vi "main 1.17b DEBUG.vi"() -> ()   [LabVIEW 2015]
uses:
  subvi/PHOIBOS/DEFINITIONS/DEF_dev_state.ctl
  subvi/PHOIBOS/DEFINITIONS/DEF_dev_type.ctl
  <vilib>/Analysis/_algsub.llb/Real Vector Norm.vi
  <vilib>/Analysis/1siggen.llb/Ramp Pattern by Samples.vi
  <vilib>/DAQmx/create/channels.llb/DAQmx Create Channel (DI-Digital Input).vi
  <userlib>/caLab/Private/Put_DBL_PV.vi
  <vilib>/Utility/file.llb/Write Delimited Spreadsheet (string).vi
  <vilib>/Utility/file.llb/Read Delimited Spreadsheet (string).vi
  <userlib>/caLab/Private/Get_PV.vi
  <vilib>/Utility/file.llb/Write Delimited Spreadsheet (DBL).vi
  subvi/Newport ESP301/Newport ESP301.lvlib
  subvi/sp_manip.llb/sp_manip_lib.lvlib
  subvi/sp_manip.llb/tcp_gateway.lvlib
  <vilib>/Analysis/NI_AALBase.lvlib
  <vilib>/Analysis/NI_AALPro.lvlib
  subvi/ZaberTSeries/ZaberTSeries.lvlib
panel:
  in  "file path (use dialog)":path=path "C:/Users/femtolab_admin/Desktop/debug.txt"
  out "Pics L":i32=200
  out "Waveform Chart":dbl(graph)
  out "G2 X":cluster{dbl[], "Ramp Pattern":dbl[]}(graph)={array[344 elements], "Ramp Pattern"=[0.0, 0.0, 0.0, 0.0, 0.0, 0.0, 0.0, 0.0, 0.0, 0.0, 0.0, 0.0, 0.0, 0.0, 0.0, 0.0, 0.0, 0.0, 0.0, 0.0, 0.0, 12.377241379310345, 41.64689655172414, 18.335172413793103, 0.0, 0.0, 0.0, 0.0, 0.0, 0.0, 0.0, 0.0, 0.0, 0.0, 0.0, 0.0, 0.0, 0.0, 0.0, 0.0, 0.0, 0.0, 0.0, 0.0, 0.0, 0.0, 0.0, 0.0, 0.0, 0.0, 0.0, 0.0, 0.0, 0.0, 0.0, 0.0, 0.0, 0.0, 0.0, 0.0, 0.0, 0.0, 0.0, 0.0, 0.0, 0.0, 0.0, 0.0, 0.0, 0.0, 0.0, 0.0, 0.0, 0.0, 0.0, 0.0, 0.0, 0.0, 0.0, 0.0, 0.0, 0.0, 0.0, 0.0, 0.0, 0.0, 0.0, 0.0, 0.0, 0.0, 0.0, 0.0, 0.0, 0.0, 0.0, 0.0, 0.0, 0.0, 0.0, 0.0, 0.0, 0.0, 0.0, 0.0, 0.0, 0.0, 0.0, 0.0, 0.0, 0.0, 0.0, 0.0, 0.0, 0.0, 0.0, 17.495517241379314, 48.13413793103449, 27.429999999999996, 0.0, 0.0, 0.0, 0.0, 0.0, 0.0, 0.0, 0.0, 0.0, 0.0, 0.0, 0.0, 0.0, 0.0, 0.0, 0.0, 0.0, 0.0, 0.0, 0.0, 0.0, 0.0, 0.0, 0.0, 0.0, 0.0, 0.0, 0.0, 0.0, 0.0, 0.0, 0.0, 0.0, 0.0, 0.0, 0.0, 0.0, 0.0, 0.0, 0.0, 0.0, 0.0, 0.0, 0.0, 0.0, 0.0, 0.0, 0.0, 0.0, 0.0, 0.0, 0.0, 0.0, 0.0, 0.0, 0.0, 0.0, 0.0, 0.0, 0.0, 0.0, 0.0, 0.0, 0.0, 17.760344827586206, 28.923448275862068, 17.532068965517244, 0.0, 0.0, 0.0, 0.0, 0.0, 0.0, 0.0, 0.0, 0.0, 0.0, 0.0, 0.0, 0.0, 0.0, 0.0, 0.0, 0.0, 0.0, 0.0, 0.0, 0.0, 0.0, 0.0, 0.0, 0.0, 0.0, 0.0, 0.0, 0.0, 0.0, 0.0, 0.0, 0.0, 0.0, 0.0, 0.0, 0.0, 0.0, 0.0, 0.0, 0.0, 0.0, 0.0, 0.0, 0.0, 2.201724137931034, 1.9948275862068956, 0.0, 0.0, 0.0, 0.0, 0.0, 0.0, 0.0, 0.0, 0.0, 0.0, 0.0, 0.0, 0.0, 0.0, 0.0, 0.0, 0.0, 0.0, 0.0, 0.0, 0.0, 0.0, 0.0, 0.0, 0.0, 0.0, 0.0, 0.0, 0.0, 0.0, 0.0, 0.0, 0.0, 0.0, 0.0, 0.0, 0.0, 0.0, 0.0, 0.0, 0.0, 0.0, 0.0, 0.0, 0.0, 0.0, 0.0, 0.0, 0.0, 0.0, 0.0, 0.0, 0.0, 0.0, 0.0, 0.0, 0.0, 0.0, 0.0, 0.0, 0.0, 0.0, 0.0, 0.0, 0.0, 0.0, 0.0, 0.0, 0.0, 0.0, 0.0, 0.0, 0.0, 0.0, 0.0, 0.0, 0.0, 0.0, 0.0, 0.0, 0.0, 0.0, 0.0, 0.0, 0.0, 0.0, 0.0, 0.0, 0.0, 0.0, 0.0, 0.0, 0.0, 0.0, 0.0, 0.0, 0.0, 0.0, 0.0, 0.0, 0.0, 0.0, 0.0, 0.0, 0.0, 0.0, 0.0, 0.0, 0.0, 0.0, 0.0, 0.0]}
  in  "reset every n pics":bool=TRUE
  in  "pics2avg":i32=50
  in  "abort acq.":bool
  out "G2 Y":cluster{dbl[], "Ramp Pattern":dbl[]}(graph)={[0.0, 0.0, 0.0, 0.0, 0.0, 0.0, 0.0, 0.0, 0.0, 0.0, 0.0, 0.0, 0.0, 0.0, 0.0, 0.0, 0.0, 0.0, 0.0, 0.0, 0.0, 0.0, 0.0, 0.0, 0.0, 0.0, 0.0, 0.0, 0.0, 0.0, 0.0, 0.0, 0.0, 0.0, 0.0, 0.0, 0.0, 0.0, 0.0, 0.0, 0.0, 0.0, 0.0, 0.0, 0.0, 0.0, 0.0, 0.0, 0.0, 0.0, 0.0, 0.0, 0.0, 0.0, 0.0, 0.0, 0.0, 0.0, 0.0, 0.0, 0.0, 0.0, 0.0, 0.0, 0.0, 0.0, 0.0, 0.0, 0.0, 0.0, 0.0, 0.0, 0.0, 0.0, 0.0, 0.0, 0.0, 0.0, 0.0, 0.0, 0.0, 0.0, 0.0, 0.0, 0.0, 0.0, 0.0, 0.0, 0.0, 0.0, 0.0, 0.0, 0.0, 0.0, 0.0, 0.0, 0.0, 0.0, 0.0, 0.0, 0.0, 0.0, 0.0, 0.0, 0.0, 0.0, 0.0, 0.0, 0.0, 0.0, 0.0, 0.0, 0.0, 0.0, 0.0, 0.0, 0.0, 0.0, 0.0, 0.0, 0.0, 0.0, 0.0, 0.0, 0.0, 0.0, 0.0, 0.0, 0.0, 0.0, 0.0, 0.0, 0.0, 0.0, 0.0, 0.0, 0.0, 0.0, 0.0, 0.0, 0.0, 0.0, 0.0, 0.0, 0.0, 0.0, 0.0, 0.0, 0.0, 0.0, 0.0, 0.0, 0.0, 0.0, 0.0, 0.0, 0.0, 0.0, 0.0, 0.0, 0.0, 0.0, 0.0, 0.0, 0.0, 0.0, 0.0, 0.0, 0.0, 0.0, 0.0, 0.0, 0.0, 0.0, 0.0, 0.0, 0.0, 0.0, 0.0, 0.0, 0.0, 0.0, 0.0, 0.0, 0.0, 0.0, 0.0, 0.0, 0.0, 0.0, 0.0, 0.0, 0.0, 0.0, 0.0, 0.0, 0.0, 0.0, 0.0, 0.0, 0.0, 0.0, 0.0, 0.0, 0.0, 0.0, 0.0, 0.0, 0.0, 0.0, 0.0, 0.0, 0.0, 0.0, 0.0, 0.0, 0.0, 0.0, 0.0, 0.0, 0.0, 0.0, 0.0, 0.0, 0.0, 0.0, 0.0, 0.0, 0.0, 0.0, 0.0, 0.0, 0.0, 0.0, 0.0, 0.0, 0.0, 0.0, 0.0, 0.0, 0.0, 0.0, 0.0, 0.0, 0.0, 0.0, 0.0, 0.0, 0.0, 0.0, 0.0, 0.0, 0.0, 0.0, 0.0, 0.0], "Ramp Pattern"=[0.0, 1.003921568627451, 2.007843137254902, 3.011764705882353, 4.015686274509804, 5.019607843137255, 6.023529411764706, 7.027450980392157, 8.031372549019608, 9.035294117647059, 10.03921568627451, 11.04313725490196, 12.047058823529412, 13.050980392156863, 14.054901960784314, 15.058823529411764, 16.062745098039215, 17.066666666666666, 18.070588235294117, 19.07450980392157, 20.07843137254902, 21.08235294117647, 22.08627450980392, 23.090196078431372, 24.094117647058823, 25.098039215686274, 26.101960784313725, 27.105882352941176, 28.109803921568627, 29.113725490196078, 30.11764705882353, 31.12156862745098, 32.12549019607843, 33.129411764705885, 34.13333333333333, 35.13725490196079, 36.141176470588235, 37.14509803921569, 38.14901960784314, 39.15294117647059, 40.15686274509804, 41.16078431372549, 42.16470588235294, 43.168627450980395, 44.17254901960784, 45.1764705882353, 46.180392156862744, 47.1843137254902, 48.188235294117646, 49.1921568627451, 50.19607843137255, 51.2, 52.20392156862745, 53.207843137254905, 54.21176470588235, 55.21568627450981, 56.219607843137254, 57.22352941176471, 58.227450980392156, 59.23137254901961, 60.23529411764706, 61.23921568627451, 62.24313725490196, 63.247058823529414, 64.25098039215686, 65.25490196078431, 66.25882352941177, 67.26274509803922, 68.26666666666667, 69.27058823529411, 70.27450980392157, 71.27843137254902, 72.28235294117647, 73.28627450980392, 74.29019607843138, 75.29411764705883, 76.29803921568627, 77.30196078431372, 78.30588235294118, 79.30980392156863, 80.31372549019608, 81.31764705882352, 82.32156862745099, 83.32549019607843, 84.32941176470588, 85.33333333333333, 86.33725490196079, 87.34117647058824, 88.34509803921569, 89.34901960784313, 90.3529411764706, 91.35686274509804, 92.36078431372549, 93.36470588235294, 94.3686274509804, 95.37254901960785, 96.37647058823529, 97.38039215686274, 98.3843137254902, 99.38823529411765, 100.3921568627451, 101.39607843137254, 102.4, 103.40392156862745, 104.4078431372549, 105.41176470588235, 106.41568627450981, 107.41960784313726, 108.4235294117647, 109.42745098039215, 110.43137254901961, 111.43529411764706, 112.43921568627451, 113.44313725490196, 114.44705882352942, 115.45098039215686, 116.45490196078431, 117.45882352941176, 118.46274509803922, 119.46666666666667, 120.47058823529412, 121.47450980392156, 122.47843137254903, 123.48235294117647, 124.48627450980392, 125.49019607843137, 126.49411764705883, 127.49803921568628, 128.50196078431372, 129.50588235294117, 130.50980392156862, 131.51372549019607, 132.51764705882354, 133.521568627451, 134.52549019607844, 135.52941176470588, 136.53333333333333, 137.53725490196078, 138.54117647058823, 139.54509803921567, 140.54901960784315, 141.5529411764706, 142.55686274509804, 143.5607843137255, 144.56470588235294, 145.5686274509804, 146.57254901960783, 147.57647058823528, 148.58039215686276, 149.5843137254902, 150.58823529411765, 151.5921568627451, 152.59607843137255, 153.6, 154.60392156862744, 155.6078431372549, 156.61176470588236, 157.6156862745098, 158.61960784313726, 159.6235294117647, 160.62745098039215, 161.6313725490196, 162.63529411764705, 163.6392156862745, 164.64313725490197, 165.64705882352942, 166.65098039215687, 167.65490196078431, 168.65882352941176, 169.6627450980392, 170.66666666666666, 171.6705882352941, 172.67450980392158, 173.67843137254903, 174.68235294117648, 175.68627450980392, 176.69019607843137, 177.69411764705882, 178.69803921568626, 179.7019607843137, 180.7058823529412, 181.70980392156864, 182.71372549019608, 183.71764705882353, 184.72156862745098, 185.72549019607843, 186.72941176470587, 187.73333333333332, 188.7372549019608, 189.74117647058824, 190.7450980392157, 191.74901960784314, 192.75294117647059, 193.75686274509803, 194.76078431372548, 195.76470588235293, 196.7686274509804, 197.77254901960785, 198.7764705882353, 199.78039215686275, 200.7843137254902, 201.78823529411764, 202.7921568627451, 203.79607843137254, 204.8, 205.80392156862746, 206.8078431372549, 207.81176470588235, 208.8156862745098, 209.81960784313725, 210.8235294117647, 211.82745098039214, 212.83137254901962, 213.83529411764707, 214.8392156862745, 215.84313725490196, 216.8470588235294, 217.85098039215686, 218.8549019607843, 219.85882352941175, 220.86274509803923, 221.86666666666667, 222.87058823529412, 223.87450980392157, 224.87843137254902, 225.88235294117646, 226.8862745098039, 227.89019607843136, 228.89411764705883, 229.89803921568628, 230.90196078431373, 231.90588235294118, 232.90980392156862, 233.91372549019607, 234.91764705882352, 235.92156862745097, 236.92549019607844, 237.9294117647059, 238.93333333333334, 239.93725490196078, 240.94117647058823, 241.94509803921568, 242.94901960784313, 243.95294117647057, 244.95686274509805, 245.9607843137255, 246.96470588235294, 247.9686274509804, 248.97254901960784, 249.9764705882353, 250.98039215686273, 251.98431372549018, 252.98823529411766, 253.9921568627451, 254.99607843137255, 256.0]}
  out "ETA":timestamp=timestamp(3655133644.4615793 s since 1904-01-01) format="%<%H:%M:%S>T"
  out "acq. imgs":i32=200
  out "snap_prog":dbl(slide)=1.0 scale=0.0..1.0
  in  "BasePath":path=path "T:/trARPES/PESData"
  in  "cam_liveavg":bool=TRUE caption="live average"
  out "cam_fps":dbl=19.690658487387566 caption="FPS" format="%.1g"
  out "sideimg":dbl[][](graph)
  out "RunNumber":u16=3091
  out "sum":dbl format="%#.2g"
  out "max":dbl=22.774482758620692
  out "mainimg":dbl[][](graph)
  out "ESP_con?":bool=TRUE caption="ESP301"
  out "phoib_con?":bool caption="PHOIBOS"
  out "manip_con?":bool=TRUE caption="manipulator"
  out "cam_con?":bool caption="camera"
  in  "main_close":bool=TRUE
  in  "Tab Control":enum32{"live", "scan", "devices"}(tab)=enum."devices"
  in  "wattpilot_set":bool
  out "Readback_wattpilot":dbl=304.89
  in  "Set Powet (%)":dbl
  out "Readback":dbl=340.0
  out "In Range":bool
  in  "setpoint_set":bool
  in  "Setpoint":dbl=302.0
  out "TB":dbl=304.91
  out "TA":dbl=304.49
  in  "phoib_I_10s":dbl
  out "phoib_I_10":dbl caption="Mesh Back"
  in  "mirr_go":bool
  in  "ESP_opent0file":bool
  in  "mirr_rel":i32=1 caption="relative [steps]"
  in  "mirr_Y-":bool
  in  "mirr_Y+":bool
  in  "mirr_X+":bool
  in  "mirr_X-":bool
  in  "manip_deltas":dbl[](array[numeric])=[0.0, 0.0, 5.0, 0.0, 0.0, 0.0] caption="delta" format="%#.5g"
  in  "aq.mode":enum32{"Radio Selection 1", "Radio Selection 2"}(radio)=enum."Radio Selection 2"
  in  "dark avg":i32=100
  in  "cam_avgs":i32=20 caption="N"
  in  "ESP_delta":dbl caption="relative [mm]"
  in  "ESP_-":bool
  in  "ESP_+":bool
  in  "ESP_go":bool
  in  "ESP_dest_t":dbl=728236.1319443199 caption="[fs]"
  in  "ESP_dest":dbl=-35.84015 caption="[mm]"
  in  "ESP_set_t0":bool
  in  "phoib_I_6s":dbl=3200.0
  in  "phoib_I_5s":dbl=1500.0
  in  "phoib_I_4s":dbl=4.558
  in  "phoib_I_3s":dbl=-10.0
  in  "phoib_I_2s":dbl=35.0
  in  "phoib_I_1s":dbl=21.0
  in  "phoib_standby":bool
  in  "phoib_set":bool
  out "phoib_I_6":dbl=3200.0 caption="Screen Voltage"
  out "phoib_I_5":dbl=1500.0 caption="Detctor Voltage"
  out "phoib_I_4":dbl=4.558 caption="Work Function"
  out "phoib_I_3":dbl=-10.0 caption="Coil Current"
  out "phoib_I_2":dbl=35.0 caption="Pass Energy"
  out "phoib_I_1":dbl=21.0 caption="Kinetic Energy"
  out "Saved Positions":string[][](table)=[["ertwertwert", "-2.299945", "-2.030214", "38.900024", "50.000762", "0.000887", "-97.998082"], ["uztgugt", "-14.999451", "-13.638894", "442.380066", "13.998380", "-1.893758", "-76.305838"], ["asdf", "-14.999451", "-13.638894", "442.380066", "13.998380", "-1.893758", "-76.305838"], ["test3", "-14.999451", "-13.638894", "441.380066", "13.998380", "-1.893758", "-76.305838"]]
  in  "Save Pos":bool
  in  "Load":bool
  in  "Delete":bool
  in  "ManipRel +":bool
  in  "ManipRel -":bool
  in  "Move Abs":bool
  in  "stop manip":bool
  in  "dest":dbl[](array[numeric])=[1.794011231344732, -4.007411134769244, 35.099853515625, 337.9843004481455, 2.0, 140.61656469713384] caption="destination" format="%#.5g"
  out "axis":string[](array[string])=["x", "y", "z", "polar", "tilt", "azimut"]
  out "pos":dbl[](array[numeric])=[1.794011231344732, -4.007411134769244, 35.099853515625, 337.9843004481455, 1.998632949125299, 140.61656469713384] caption="position" format="%.5f"
  in  "ana_mode":T1(ring)=enum."WideAngleMode"
  in  "ana_voltrange":enum16{"3.5kV", "1.5kV", "400V", "100V", "10V"}(ring)=enum."400V"
  out "ESP_pos":dbl=-35.84015 caption="Position"
  out "ESP_delay":dbl=-0.3335640952092252 caption="Delay"
  out "ESP_t0":dbl=-35.8401 caption="Time Zero @"
  out "phoib_I_7":dbl=-30.0 caption="Conversion Voltage"
  in  "phoib_I_7s":dbl=-30.0
  in  "phoib_I_8s":dbl=0.0039
  in  "phoib_I_9s":dbl
  out "phoib_I_8":dbl=0.0039 caption="FD1"
  out "phoib_I_9":dbl caption="Mesh Front"
  in  "gain":bool
  in  "cam_exp":u32=50 caption="exposure [ms]"
  in  "binning":u16(ring)=2 items=["X 1", "X 2", "X 4", "X 8"]
  in  "cam_dark?":bool=TRUE caption="subtract dark?"
  in  "cam_dark":bool
  in  "cam_saveimg":bool
  in  "e-size":u8
  in  "lower threshold":i32=50
  in  "count?":bool
  in  "ROI Left":i32=1
  in  "ROI Right":i32=43
  in  "ROI Top":i32=1
  in  "ROI Bottom":i32=33
  out "moving?":bool[](array[boolean])
  out "mirr_posX":i32=1955 caption="X"
  out "mirr_posY":i32=2950 caption="Y"
  in  "mirr_dest":i32[](array[numeric])=[60782, 121383]
  out "waveplate position":dbl format="%.6g"
  out "stage2 position":dbl format="%.6g"
  out "current scan 2":i32=3
  out "scan 1":dbl(slide)=1.0 scale=0.0..1.0
  in  "Tab Control 2":enum32{"setup", "data"}(tab)
  in  "scan_selector 2":T2(tab)
  in  "scan_manip_start 2":dbl[](array[numeric])=[1.794011231344732, -4.007411134769244, 35.099853515625, 337.9843004481455, 2.000390761745462, 140.61656469713384] caption="start position" format="%#.5g"
  in  "scan_manip_deltas 2":dbl[](array[numeric])=[0.0, 0.0, 0.0, 0.0, 1.0, 0.0] caption="direction vector\n(gets normalized)" format="%#.5g"
  in  "scan_manip_setstart 2":bool
  in  "scan_mirr_start 2":i32[](array[numeric])=[60782, 121383] caption="scan_mirr_start"
  in  "scan_mirr_deltas 2":i32[](array[numeric])=[1, 0] caption="direction vector\n(gets normalized)"
  in  "scan_mirr_setstart 2":bool
  in  "wait addional  2":dbl caption="s"
  in  "Wait for T 2":bool=TRUE
  in  "scan_volt_parameter 2":string(combo)="Kinetic Energy"
  in  "waypointsD2":string[][](table)
  in  "waypointsD1":string[][](table)=[["302", "1"], ["304", ""], ["", ""]]
  in  "load waypoints 1":bool
  in  "meas_iter":i32=1 caption="Iterations"
  in  "scan_selector":T2(tab)=enum."delay"
  in  "scan_manip_setstart":bool
  in  "scan_manip_start":dbl[](array[numeric])=[1.794011231344732, -4.007411134769244, 35.099853515625, 337.9843004481455, 2.000390761745462, 140.61656469713384] caption="start position" format="%#.5g"
  in  "scan_manip_deltas":dbl[](array[numeric])=[0.0, 0.0, 0.0, 0.0, 1.0, 0.0] caption="direction vector\n(gets normalized)" format="%#.5g"
  in  "scan_mirr_start":i32[](array[numeric])=[60782, 121383]
  in  "scan_mirr_deltas":i32[](array[numeric])=[1, 0] caption="direction vector\n(gets normalized)"
  in  "scan_mirr_setstart":bool
  in  "wait addional":dbl caption="s"
  in  "Wait for T":bool=TRUE
  in  "scan_volt_parameter":string(combo)="Kinetic Energy"
  in  "clear waypoints 1":bool
  in  "load waypoints 2":bool
  in  "clear waypoints 2":bool
  out "intensitygraph":cluster{"Array":dbl[], "Intensity Chart":dbl[]}(graph)={"Array"=[302.0, 303.0, 304.0], "Intensity Chart"=[1937.88, 12704.590000000002, 4640.840000000001]}
  out "energygraph":dbl[][](graph)=[[0.0, 0.0, 0.0, 64.28999999999999, 120.06, 0.0, 0.0, 0.0, 0.0, 0.0, 0.0, 0.0, 0.0, 0.0, 0.0, 0.0, 0.0, 0.0, 0.0, 0.0, 0.0, 0.0, 0.0, 0.0, 0.0, 0.0, 0.0, 0.0, 0.0, 0.0, 0.0, 0.0, 0.0, 0.0, 0.0, 0.0, 0.0, 0.0, 0.0, 0.0, 0.0, 0.0, 0.0, 0.0, 0.0, 0.0, 0.0, 0.0, 0.0, 384.53999999999996, 1103.3799999999999, 448.21000000000004, 0.0, 0.0, 0.0, 0.0, 0.0, 0.0, 0.0, 0.0, 0.0, 0.0, 0.0, 0.0, 0.0, 0.0, 0.0, 0.0, 0.0, 120.82, 0.0, 261.04, 195.1, 253.87, 199.70999999999998, 127.75, 87.50999999999999, 0.0, 52.54, 0.0, 0.0, 51.78, 55.73, 0.0, 0.0, 0.0, 0.0, 0.0, 0.0, 0.0, 0.0, 0.0, 0.0, 0.0, 0.0, 0.0, 0.0, 0.0, 0.0, 0.0, 0.0, 0.0, 0.0, 0.0, 0.0, 0.0, 0.0, 0.0, 0.0, 0.0, 0.0, 0.0, 0.0, 332.90999999999997, 1106.25, 934.74, 0.0, 156.76, 62.65, 0.0, 0.0, 0.0, 0.0, 0.0, 0.0, 54.62, 0.0, 0.0, 0.0, 0.0, 0.0, 0.0, 0.0, 0.0, 0.0, 0.0, 0.0, 0.0, 0.0, 0.0, 0.0, 0.0, 0.0, 0.0, 65.85, 165.75, 0.0, 0.0, 0.0, 0.0, 0.0, 0.0, 0.0, 0.0, 0.0, 0.0, 0.0, 0.0, 0.0, 0.0, 0.0, 0.0, 0.0, 266.63, 591.5, 261.64, 0.0, 391.9, 527.29, 82.87, 123.75, 286.74, 151.72, 0.0, 0.0, 0.0, 0.0, 0.0, 0.0, 0.0, 0.0, 0.0, 0.0, 0.0, 0.0, 0.0, 0.0, 0.0, 0.0, 0.0, 0.0, 0.0, 396.37, 721.0900000000001, 353.5, 83.97999999999999, 104.77000000000001, 0.0, 57.83, 60.98, 182.28, 128.78, 0.0, 0.0, 0.0, 465.25, 624.3399999999999, 348.62, 0.0, 0.0, 0.0, 0.0, 0.0, 0.0, 0.0, 0.0, 0.0, 0.0, 0.0, 0.0, 119.7, 217.91, 120.56, 0.0, 0.0, 0.0, 0.0, 0.0, 0.0, 0.0, 58.89, 0.0, 0.0, 0.0, 202.23999999999998, 149.79000000000002, 0.0, 117.82, 212.51999999999998, 534.74, 421.98, 50.97, 0.0, 0.0, 0.0, 0.0, 362.15999999999997, 656.04, 265.02, 0.0, 0.0, 0.0, 0.0, 0.0, 0.0, 0.0, 0.0, 0.0, 0.0, 0.0, 0.0, 0.0, 0.0, 0.0, 0.0, 0.0, 0.0, 0.0, 0.0, 0.0, 0.0, 0.0, 0.0, 0.0, 0.0, 0.0, 0.0, 0.0, 0.0, 0.0, 0.0, 0.0, 0.0, 0.0, 0.0, 0.0, 0.0, 0.0, 0.0, 0.0, 0.0, 0.0, 0.0, 0.0, 0.0, 0.0, 0.0, 0.0, 0.0, 0.0, 0.0, 0.0, 0.0, 0.0, 0.0, 0.0, 0.0, 0.0, 0.0, 0.0, 0.0, 0.0, 0.0, 237.67999999999998, 286.08, 130.9, 0.0, 0.0, 0.0, 0.0, 0.0, 0.0, 0.0, 0.0, 0.0, 0.0, 0.0, 0.0, 0.0, 0.0, 0.0, 0.0, 0.0, 0.0, 0.0, 0.0, 0.0, 0.0, 0.0, 0.0, 0.0, 0.0, 0.0, 0.0], [0.0, 0.0, 0.0, 0.0, 0.0, 0.0, 0.0, 0.0, 0.0, 0.0, 0.0, 0.0, 0.0, 0.0, 0.0, 0.0, 0.0, 485.13, 1279.2, 234.71, 0.0, 0.0, 0.0, 0.0, 0.0, 0.0, 0.0, 0.0, 0.0, 0.0, 0.0, 0.0, 50.5, 654.4200000000001, 511.98, 0.0, 0.0, 0.0, 0.0, 0.0, 0.0, 0.0, 0.0, 0.0, 0.0, 0.0, 0.0, 0.0, 0.0, 0.0, 0.0, 0.0, 0.0, 0.0, 0.0, 0.0, 0.0, 0.0, 63.72, 693.84, 574.54, 0.0, 0.0, 0.0, 68.68, 1054.28, 1010.9499999999999, 0.0, 0.0, 0.0, 0.0, 0.0, 0.0, 0.0, 0.0, 0.0, 0.0, 0.0, 56.57, 971.76, 1333.73, 330.0, 0.0, 0.0, 0.0, 0.0, 0.0, 349.33000000000004, 292.7, 0.0, 0.0, 0.0, 0.0, 0.0, 0.0, 82.77000000000001, 1059.23, 1069.87, 156.47, 0.0, 0.0, 0.0, 0.0, 293.91, 333.47, 551.4, 493.64, 73.72999999999999, 0.0, 0.0, 0.0, 0.0, 0.0, 0.0, 0.0, 0.0, 0.0, 0.0, 0.0, 0.0, 0.0, 0.0, 286.01, 543.0699999999999, 251.94, 0.0, 0.0, 0.0, 0.0, 0.0, 233.63, 968.4799999999999, 771.53, 109.94, 0.0, 123.07, 499.72999999999996, 431.4, 0.0, 0.0, 60.85, 69.5, 0.0, 0.0, 0.0, 0.0, 0.0, 0.0, 0.0, 0.0, 0.0, 0.0, 0.0, 0.0, 0.0, 0.0, 52.01, 0.0, 0.0, 0.0, 0.0, 0.0, 0.0, 0.0, 0.0, 0.0, 0.0, 0.0, 0.0, 0.0, 0.0, 0.0, 0.0, 0.0, 0.0, 0.0, 0.0, 0.0, 0.0, 0.0, 0.0, 0.0, 0.0, 0.0, 0.0, 0.0, 0.0, 0.0, 0.0, 0.0, 52.95, 478.8, 870.47, 572.83, 61.67, 268.19, 1143.4, 1804.2599999999998, 1145.6100000000001, 739.22, 904.59, 1109.3000000000002, 1233.6599999999999, 212.92, 0.0, 0.0, 105.95, 448.76000000000005, 1306.3500000000001, 1005.5900000000001, 68.8, 0.0, 57.94, 0.0, 0.0, 0.0, 0.0, 0.0, 0.0, 0.0, 0.0, 0.0, 0.0, 0.0, 0.0, 0.0, 0.0, 0.0, 0.0, 0.0, 0.0, 0.0, 0.0, 0.0, 0.0, 0.0, 0.0, 159.01, 520.94, 925.5600000000001, 1641.53, 2261.26, 1259.83, 0.0, 0.0, 0.0, 0.0, 0.0, 0.0, 136.69, 398.81, 382.02, 0.0, 0.0, 0.0, 0.0, 0.0, 0.0, 421.01, 1376.5800000000002, 1425.75, 268.07, 0.0, 345.84000000000003, 396.77, 0.0, 0.0, 0.0, 0.0, 0.0, 216.93, 727.65, 830.9, 774.2299999999999, 839.3900000000001, 309.97, 0.0, 0.0, 0.0, 0.0, 0.0, 0.0, 0.0, 100.57, 459.66, 305.86, 0.0, 0.0, 0.0, 0.0, 0.0, 0.0, 0.0, 0.0, 0.0, 0.0, 0.0, 0.0, 0.0, 0.0, 0.0, 0.0, 0.0, 0.0, 0.0, 0.0, 0.0, 0.0, 0.0, 0.0, 0.0, 64.97999999999999, 379.62, 337.15999999999997, 83.6, 463.66, 399.03999999999996, 0.0, 0.0, 0.0, 0.0, 0.0, 0.0, 0.0, 0.0, 0.0, 0.0, 0.0, 0.0, 0.0, 0.0, 0.0, 0.0, 0.0, 0.0, 0.0, 0.0, 0.0, 0.0, 0.0, 0.0, 0.0, 0.0, 0.0], [0.0, 0.0, 0.0, 0.0, 0.0, 0.0, 0.0, 0.0, 0.0, 0.0, 0.0, 0.0, 0.0, 0.0, 0.0, 165.83, 124.99, 78.27000000000001, 0.0, 0.0, 0.0, 765.77, 1457.88, 293.67, 0.0, 0.0, 0.0, 0.0, 0.0, 0.0, 0.0, 0.0, 0.0, 0.0, 0.0, 0.0, 0.0, 0.0, 0.0, 0.0, 0.0, 0.0, 0.0, 0.0, 0.0, 0.0, 0.0, 0.0, 0.0, 85.5, 116.32, 0.0, 0.0, 0.0, 0.0, 0.0, 0.0, 0.0, 0.0, 0.0, 0.0, 0.0, 0.0, 0.0, 0.0, 0.0, 0.0, 0.0, 179.01, 123.78999999999999, 64.69, 0.0, 433.57000000000005, 1457.15, 661.49, 0.0, 0.0, 0.0, 0.0, 0.0, 0.0, 171.38, 497.28999999999996, 835.47, 1797.0300000000002, 1202.25, 169.95, 0.0, 0.0, 0.0, 0.0, 383.74, 496.08, 196.89999999999998, 0.0, 0.0, 0.0, 0.0, 719.08, 1717.5100000000002, 1360.8, 163.65, 118.56, 798.75, 610.32, 0.0, 0.0, 0.0, 0.0, 73.12, 51.75, 0.0, 0.0, 0.0, 0.0, 0.0, 0.0, 0.0, 0.0, 0.0, 0.0, 0.0, 233.35000000000002, 1128.3, 1138.8400000000001, 207.43, 0.0, 0.0, 50.52, 0.0, 0.0, 0.0, 0.0, 0.0, 0.0, 0.0, 0.0, 0.0, 0.0, 0.0, 0.0, 0.0, 0.0, 0.0, 0.0, 0.0, 0.0, 0.0, 0.0, 0.0, 0.0, 122.82, 66.93, 184.87, 606.35, 1065.2, 616.33, 82.97, 0.0, 0.0, 0.0, 0.0, 0.0, 0.0, 0.0, 0.0, 0.0, 0.0, 0.0, 210.77, 369.49, 0.0, 0.0, 0.0, 0.0, 0.0, 0.0, 0.0, 0.0, 0.0, 0.0, 0.0, 0.0, 0.0, 0.0, 0.0, 0.0, 0.0, 0.0, 61.71, 492.70000000000005, 501.67999999999995, 50.9, 0.0, 0.0, 0.0, 0.0, 0.0, 0.0, 0.0, 0.0, 0.0, 0.0, 0.0, 0.0, 0.0, 0.0, 0.0, 0.0, 0.0, 0.0, 0.0, 0.0, 0.0, 0.0, 0.0, 0.0, 0.0, 0.0, 0.0, 0.0, 0.0, 0.0, 0.0, 0.0, 0.0, 0.0, 0.0, 0.0, 0.0, 0.0, 0.0, 0.0, 0.0, 0.0, 0.0, 0.0, 0.0, 0.0, 0.0, 0.0, 0.0, 0.0, 0.0, 0.0, 0.0, 0.0, 0.0, 0.0, 0.0, 0.0, 0.0, 0.0, 0.0, 0.0, 0.0, 0.0, 0.0, 0.0, 0.0, 0.0, 0.0, 0.0, 0.0, 0.0, 0.0, 0.0, 0.0, 0.0, 0.0, 191.69, 347.02, 262.31, 325.89, 168.79, 0.0, 0.0, 52.9, 53.13, 0.0, 0.0, 0.0, 0.0, 0.0, 0.0, 0.0, 0.0, 0.0, 0.0, 0.0, 0.0, 0.0, 0.0, 0.0, 0.0, 0.0, 0.0, 0.0, 0.0, 0.0, 0.0, 0.0, 0.0, 0.0, 0.0, 327.12, 491.83000000000004, 242.02999999999997, 0.0, 0.0, 0.0, 0.0, 0.0, 0.0, 0.0, 676.6, 975.77, 229.86, 0.0, 144.15, 151.75, 0.0, 0.0, 0.0, 0.0, 0.0, 0.0, 0.0, 0.0, 0.0, 0.0, 0.0, 0.0, 0.0, 0.0, 0.0, 0.0, 0.0, 0.0, 0.0, 0.0, 0.0, 0.0, 0.0]]
  out "anglegraph":dbl[][](graph)=[[0.0, 0.0, 0.0, 0.0, 0.0, 0.0, 0.0, 0.0, 0.0, 0.0, 0.0, 0.0, 0.0, 0.0, 0.0, 0.0, 0.0, 0.0, 0.0, 0.0, 0.0, 0.0, 0.0, 0.0, 0.0, 0.0, 0.0, 307.98, 204.45, 0.0, 0.0, 0.0, 0.0, 0.0, 0.0, 0.0, 0.0, 0.0, 0.0, 0.0, 0.0, 0.0, 0.0, 0.0, 0.0, 0.0, 0.0, 0.0, 0.0, 0.0, 0.0, 0.0, 0.0, 0.0, 0.0, 0.0, 0.0, 0.0, 0.0, 0.0, 0.0, 0.0, 0.0, 0.0, 0.0, 0.0, 0.0, 0.0, 0.0, 0.0, 0.0, 0.0, 0.0, 0.0, 0.0, 0.0, 0.0, 0.0, 0.0, 0.0, 0.0, 0.0, 0.0, 0.0, 0.0, 0.0, 0.0, 0.0, 0.0, 0.0, 0.0, 0.0, 0.0, 0.0, 0.0, 0.0, 0.0, 0.0, 0.0, 0.0, 0.0, 0.0, 0.0, 0.0, 0.0, 0.0, 0.0, 0.0, 0.0, 0.0, 0.0, 0.0, 0.0, 0.0, 0.0, 0.0, 0.0, 0.0, 0.0, 0.0, 0.0, 0.0, 0.0, 0.0, 0.0, 0.0, 0.0, 0.0, 0.0, 0.0, 0.0, 0.0, 0.0, 0.0, 0.0, 0.0, 0.0, 0.0, 0.0, 0.0, 0.0, 0.0, 0.0, 0.0, 0.0, 0.0, 0.0, 0.0, 0.0, 0.0, 0.0, 0.0, 0.0, 0.0, 0.0, 0.0, 640.8800000000001, 550.45, 91.89, 0.0, 0.0, 0.0, 0.0, 0.0, 0.0, 0.0, 0.0, 0.0, 0.0, 0.0, 0.0, 0.0, 0.0, 0.0, 0.0, 69.94, 60.96, 0.0, 0.0, 0.0, 0.0, 0.0, 0.0, 0.0, 0.0, 0.0, 0.0, 0.0, 0.0, 0.0, 0.0, 0.0, 0.0, 0.0, 0.0, 0.0, 115.87, 235.84, 172.04999999999998, 0.0, 0.0, 0.0, 0.0, 0.0, 0.0, 0.0, 0.0, 0.0, 0.0, 0.0, 0.0, 0.0, 0.0, 0.0, 0.0, 0.0, 0.0, 0.0, 0.0, 0.0, 0.0, 0.0, 0.0, 0.0, 0.0, 0.0, 0.0, 0.0, 0.0, 0.0, 0.0, 0.0, 0.0, 0.0, 0.0, 0.0, 0.0, 0.0, 0.0, 0.0, 0.0, 0.0, 0.0, 0.0, 0.0, 0.0, 0.0, 0.0, 0.0, 0.0, 0.0, 0.0, 0.0, 0.0, 0.0, 0.0], [0.0, 0.0, 0.0, 0.0, 0.0, 0.0, 0.0, 0.0, 0.0, 0.0, 0.0, 0.0, 0.0, 0.0, 0.0, 0.0, 54.97, 1426.6399999999999, 1312.94, 180.81, 0.0, 0.0, 0.0, 0.0, 0.0, 0.0, 0.0, 465.48, 989.61, 293.56, 0.0, 0.0, 0.0, 0.0, 0.0, 0.0, 0.0, 0.0, 0.0, 0.0, 0.0, 0.0, 0.0, 0.0, 0.0, 0.0, 0.0, 0.0, 0.0, 0.0, 0.0, 0.0, 0.0, 0.0, 0.0, 0.0, 0.0, 0.0, 0.0, 331.78, 944.91, 463.28, 0.0, 0.0, 0.0, 0.0, 143.70999999999998, 402.81, 196.09, 0.0, 0.0, 0.0, 483.82, 433.7, 0.0, 0.0, 0.0, 0.0, 0.0, 0.0, 89.85, 513.2, 263.03999999999996, 0.0, 0.0, 0.0, 0.0, 0.0, 0.0, 0.0, 0.0, 104.84, 0.0, 226.86, 214.93, 235.13, 0.0, 0.0, 0.0, 0.0, 0.0, 0.0, 0.0, 0.0, 0.0, 0.0, 0.0, 0.0, 0.0, 0.0, 0.0, 0.0, 0.0, 0.0, 0.0, 0.0, 0.0, 0.0, 0.0, 0.0, 0.0, 0.0, 0.0, 0.0, 0.0, 0.0, 0.0, 0.0, 0.0, 0.0, 0.0, 0.0, 0.0, 0.0, 0.0, 0.0, 0.0, 0.0, 0.0, 380.83, 649.96, 229.04, 0.0, 0.0, 0.0, 276.21000000000004, 441.79999999999995, 228.29, 0.0, 0.0, 0.0, 0.0, 0.0, 0.0, 0.0, 0.0, 0.0, 0.0, 0.0, 0.0, 0.0, 0.0, 0.0, 0.0, 0.0, 0.0, 0.0, 0.0, 123.92000000000002, 1311.81, 1454.81, 600.87, 0.0, 0.0, 0.0, 0.0, 0.0, 0.0, 0.0, 0.0, 0.0, 0.0, 0.0, 0.0, 0.0, 0.0, 0.0, 0.0, 0.0, 0.0, 0.0, 0.0, 0.0, 0.0, 0.0, 0.0, 0.0, 0.0, 0.0, 0.0, 0.0, 0.0, 654.53, 894.22, 410.35, 0.0, 0.0, 0.0, 0.0, 0.0, 0.0, 0.0, 0.0, 0.0, 0.0, 0.0, 0.0, 0.0, 0.0, 0.0, 0.0, 0.0, 0.0, 0.0, 0.0, 0.0, 0.0, 0.0, 0.0, 0.0, 0.0, 0.0, 0.0, 0.0, 0.0, 0.0, 0.0, 0.0, 0.0, 0.0, 0.0, 0.0, 0.0, 0.0, 0.0, 0.0, 0.0, 0.0, 0.0, 0.0, 0.0, 0.0, 0.0, 0.0, 0.0, 0.0], [0.0, 0.0, 0.0, 0.0, 0.0, 0.0, 0.0, 0.0, 0.0, 0.0, 0.0, 0.0, 0.0, 0.0, 0.0, 0.0, 0.0, 0.0, 0.0, 0.0, 0.0, 0.0, 0.0, 0.0, 0.0, 0.0, 0.0, 0.0, 0.0, 125.9, 1017.51, 504.48, 0.0, 0.0, 0.0, 0.0, 0.0, 0.0, 0.0, 0.0, 0.0, 0.0, 0.0, 0.0, 0.0, 0.0, 0.0, 0.0, 0.0, 0.0, 0.0, 0.0, 0.0, 0.0, 0.0, 0.0, 0.0, 0.0, 0.0, 0.0, 0.0, 0.0, 0.0, 0.0, 0.0, 0.0, 0.0, 0.0, 0.0, 0.0, 0.0, 0.0, 109.81, 66.88, 0.0, 0.0, 733.48, 806.32, 342.43, 0.0, 0.0, 0.0, 0.0, 0.0, 0.0, 0.0, 0.0, 0.0, 0.0, 0.0, 0.0, 0.0, 0.0, 0.0, 0.0, 0.0, 0.0, 0.0, 0.0, 0.0, 0.0, 0.0, 0.0, 0.0, 0.0, 174.07999999999998, 275.74, 429.21, 301.15999999999997, 0.0, 0.0, 0.0, 0.0, 0.0, 0.0, 0.0, 0.0, 0.0, 0.0, 0.0, 0.0, 0.0, 0.0, 0.0, 0.0, 0.0, 0.0, 0.0, 0.0, 0.0, 0.0, 0.0, 0.0, 0.0, 0.0, 0.0, 0.0, 0.0, 0.0, 0.0, 0.0, 0.0, 0.0, 0.0, 0.0, 0.0, 0.0, 0.0, 0.0, 0.0, 0.0, 0.0, 0.0, 0.0, 0.0, 0.0, 0.0, 0.0, 0.0, 0.0, 0.0, 0.0, 0.0, 0.0, 0.0, 0.0, 0.0, 0.0, 0.0, 0.0, 0.0, 0.0, 0.0, 0.0, 0.0, 252.98000000000002, 303.56, 60.91, 52.9, 53.13, 0.0, 0.0, 0.0, 0.0, 0.0, 0.0, 0.0, 0.0, 0.0, 0.0, 0.0, 0.0, 0.0, 0.0, 0.0, 0.0, 0.0, 0.0, 0.0, 0.0, 0.0, 0.0, 0.0, 0.0, 0.0, 0.0, 0.0, 0.0, 0.0, 0.0, 0.0, 0.0, 0.0, 61.05, 350.49, 266.71000000000004, 0.0, 0.0, 0.0, 0.0, 0.0, 0.0, 0.0, 0.0, 0.0, 0.0, 0.0, 0.0, 0.0, 0.0, 0.0, 0.0, 0.0, 0.0, 0.0, 0.0, 0.0, 0.0, 0.0, 0.0, 0.0, 0.0, 0.0, 0.0, 0.0, 0.0, 0.0, 0.0, 0.0, 0.0, 0.0, 0.0, 0.0, 0.0, 0.0, 0.0]]
  in  "stop after iteration":bool
  in  "time/step [s]":dbl=10.787117004394531
  out "current iteration":i32=1
  out "current scan":i32=3
  out "iteration":dbl(slide)=1.0 scale=0.0..1.0
  out "scan 2":dbl(slide)=1.0 scale=0.0..1.0
  in  "stop after step":bool
  in  "scan_go":bool
  out "measpoints":i32=3
  out "total steps":i32=3
  out "RAM [MB]":dbl=1.6590000000000003
  out "disk [MB]":dbl=1.6590000000000003
  out "duration [HH:MM:SS]":dbl=32.361351013183594 format="%<%H:%M:%S>t"
  out "ETA 2":timestamp
  in  "WattPilot EPICS chanel readback":string="trARPES:Wattpilot:PumpPercent_RBV"
  in  "WattPilot EPICS chanel set":string="trARPES:Wattpilot:PumpPercent"
  in  "ESP patch":i32[](array[numeric])=[3, 2, 1]
  in  "LS310  EPICS Heater":string="trARPES:Carving:HT-RNG"
  in  "LS310  EPICS SP":string="trARPES:Carving:TEMP"
  in  "LS310  EPICS chanel B":string="trARPES:Carving:TEMP-B"
  in  "mm/s":dbl
  in  "Set Speed to":bool
  in  "ESP Axis waveplate":i32=2 min=1 max=3
  in  "mirr_init":bool
  in  "mirr_release":bool
  in  "mirr_Y#":u8=2
  in  "manip_init":bool
  in  "manip_release":bool
  in  "phoib_init":bool
  in  "phoib_release":bool
  in  "ESP_init":bool
  in  "ESP_release":bool
  in  "ESP301 VISA":refnum<visa-resource-name>="COM4"
  in  "board number":i32
  in  "cam_init":bool
  in  "cam_release":bool
  out "cam_error":errorcluster
  out "phoib_error":errorcluster
  out "state":T3=1 items=["Off"=-1, "Standby"=0, "On"=1]
  in  "ESP Axis delay":i32=3 min=1 max=3
  out "error out":errorcluster={"status"=FALSE, "code"=1073676418, "source"="VISA Close in Newport ESP301.lvlib:Close.vi->main 1.17a beta.vi"}
  out "error out 2":errorcluster={"status"=TRUE, "code"=1, "source"="TCP Write in sp_manip_lib.lvlib:sp_manip_disconnect.vi->main 1.17a beta.vi"}
  out "mirr_Error":errorcluster={"status"=FALSE, "code"=1073676418, "source"="VISA Close in ZaberTSeries.lvlib:Close.vi->main 1.17a beta.vi"}
  in  "mirr_VISA":refnum<visa-resource-name>="COM7"
  in  "mirr_X#":u8=1
  in  "Operating mode\nHP & QE / HS & DiCam Pro":u32=1
  in  "Frame trigger \n(High Performance and QE only)":u16
  in  "LS310  EPICS chanel A":string="trARPES:Carving:TEMP_RBV"
  in  "Status EPICS chanel":string="trARPES:Carving:TEMP-STAT"
  # "camera"
  # "analyzer"
  # "manipulator"
  # "temperature"
  # "aquisition"
  # "delay stage"
  # "Position"
  # "Destination"
  # "WattPilot"
  # "- no settings -"
  # "waypoints are absolute values"
  # "- no settings -"
  # "waypoints are absolute values"
  # "- no settings -"
  # "waypoints are absolute values"
  # "- no settings -"
  # "waypoints are absolute values"
  # "X\nY\nZ\npolar\ntilt\nazimut"
  # "waypoint \"0\" is start position"
  # "X\nY"
  # "waypoint \"0\" is start position"
  # "waypoints are absolute values"
  # "- no settings -"
  # "waypoints are absolute values"
  # "- no settings -"
  # "waypoints are absolute values"
  # "- no settings -"
  # "waypoints are absolute values"
  # "- no settings -"
  # "waypoints are absolute values"
  # "X\nY\nZ\npolar\ntilt\nazimut"
  # "waypoint \"0\" is start position"
  # "X\nY"
  # "waypoint \"0\" is start position"
  # "waypoints are absolute values"
  # "camera"
  # "phoibos"
  # "ESP301"
  # "manipulator"
  # "mirror"
  # "delay"
  # "waveplate"
  # "stage2"
  # "0 = sequential\n1 = simultaneous"
  # "0 = internal\n1 = external rising\n2 = external falling"
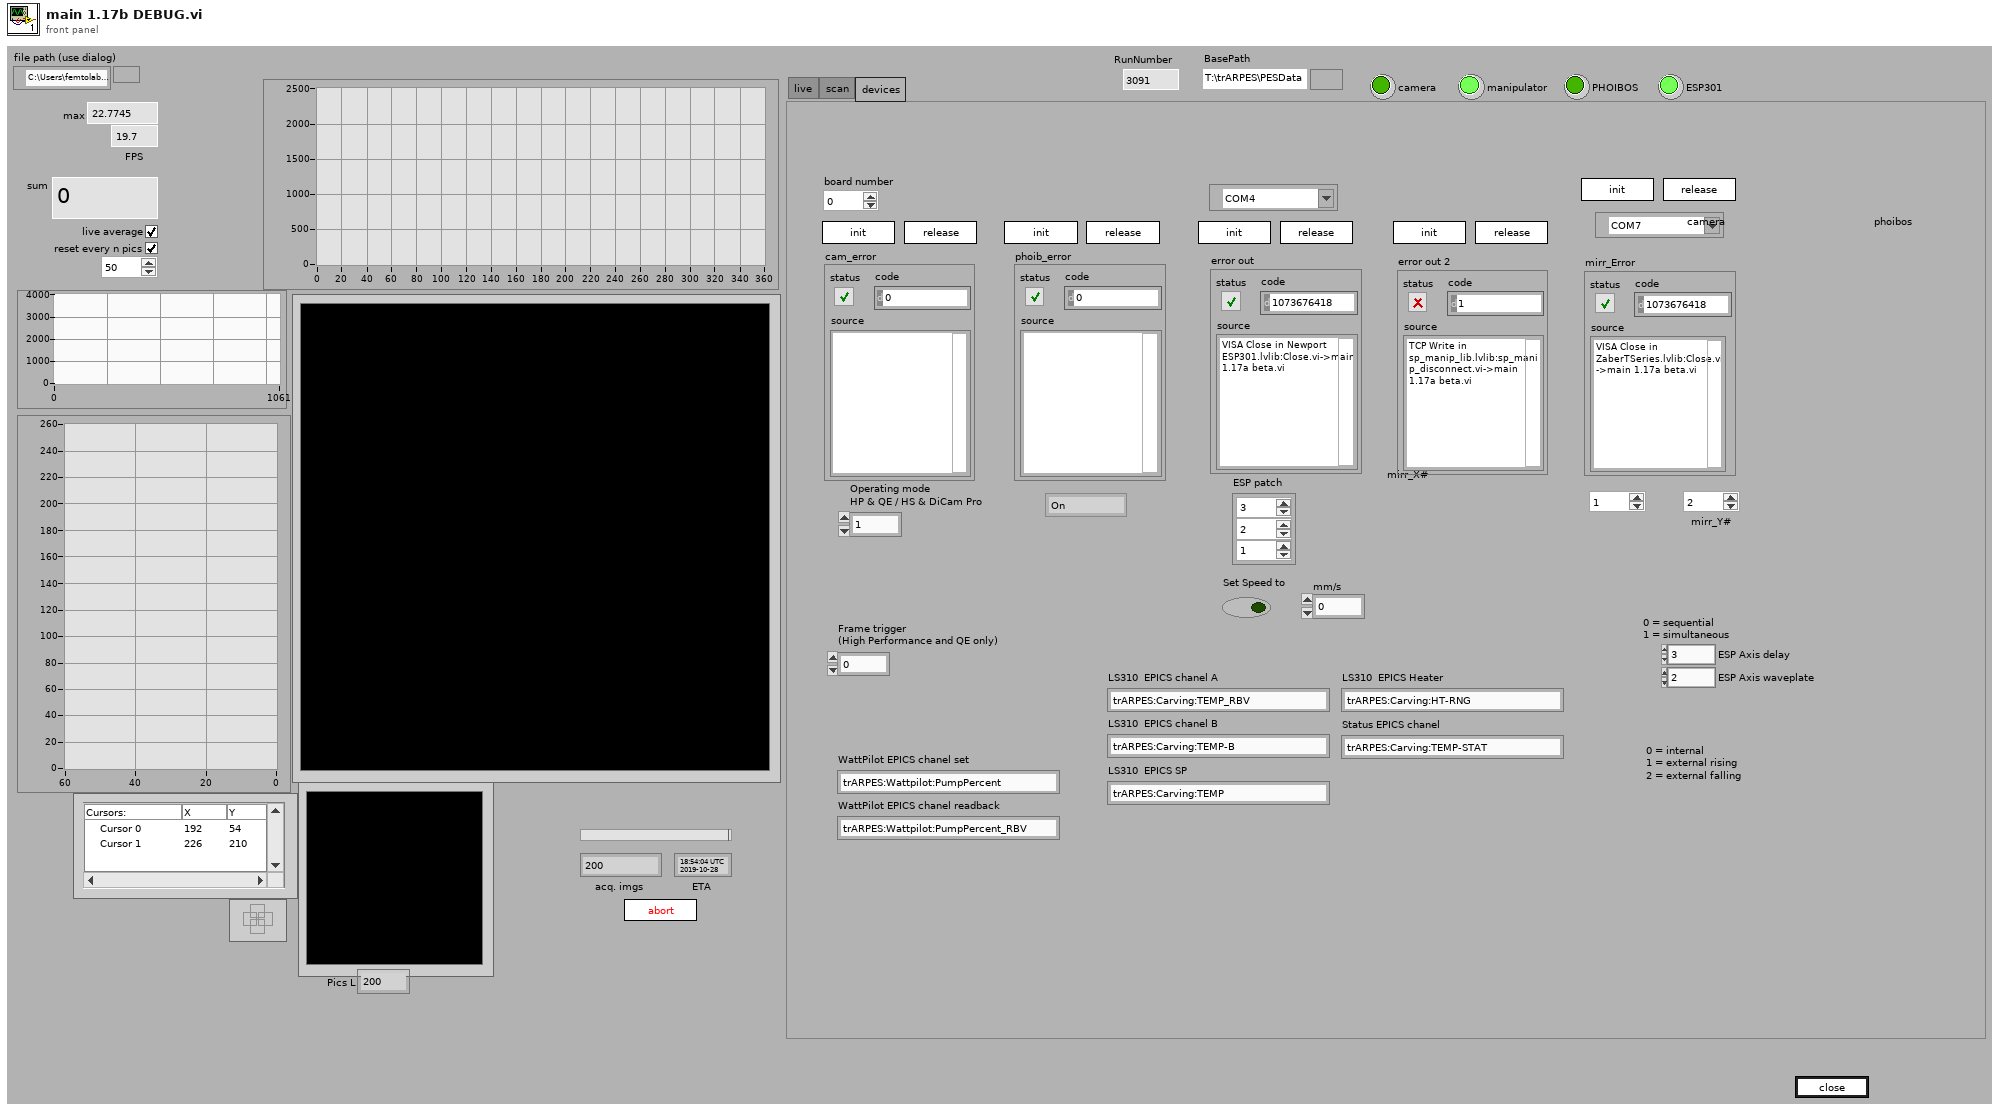
[diagram p1: front panel]
types:
  T1 = enum16{"HighMagnification", "MediumMagnification", "LowMagnification", "HighAngularDispersion", "MediumAngularDispersion", "LowAngularDispersion", "WideAngleMode", "LargeArea", "MediumArea", "SmallArea", "HighMagnification2", "SmallArea2"}
  T2 = enum32{"none", "delay", "wattpilot", "waveplate", "stage2", "manipulator", "mirror", "temperature", "voltage"}
  T3 = typedef "DEF_dev_state.ctl" = i32
  T4 = cluster{"queue out":refnum<queue>, "queue out":refnum<queue>, "queue out":refnum<queue>, "queue out":refnum<queue>, "queue out":refnum<queue>, "queue out":refnum<queue>, "queue out":refnum<queue>}
  T5 = typedef "LVCursorListTypeDef.ctl" = cluster{"Name":string, "Color":u32, "Style":u8, "Point Style":u8, "Name Visible":bool, "Allow Drag":bool, "Cursor Mode":u32, "Plot":i32, "Index":i32, "Position":cluster{"X":dbl, "Y":dbl}, "X Scale":u32, "Y Scale":u32, "Watch Plots":i32[], "Watch All Plots":bool, "Plot Area":i32, "Label Offset":cluster{"X":dbl, "Y":dbl}}[]
  T6 = cluster{"mirr_X#":u8, "Command":u8, dbl, "Response Count":i32}
  T7 = cluster{"mirr_Y#":u8, "Command":u8, dbl, "Response Count":i32}
  T8 = cluster{i32, "Command":u8, i32, "Response Count":i32}
  T9 = cluster{"Axis_Name":string, "Axis_Type":string, "Axis_Position":dbl, "continous":bool, "moving":bool}[]
  T10 = typedef "DEF_dev_type.ctl" = enum32{"devA (analyzer)", "devD (detector)"}
  T11 = cluster{"Camera type":u32, "Operating mode\nHP & QE / HS & DiCam Pro ":u32, "Frame trigger \n(High Performance and QE only)":u16, "Sequence trigger":u16, "Low Light\n(QE only)":bool, "Gain":bool, "Horzontal\nbinning":u16, "Vertical\nbinning ":u16, "ROI Left":i32, "ROI Right":i32, "ROI Top":i32, "ROI Bottom":i32}
  T12 = cluster{"Name":string, "Color":u32, "Style":u8, "Point Style":u8, "Name Visible":bool, "Allow Drag":bool, "Cursor Mode":u32, "Plot":i32, "Index":i32, "Position":cluster{"X":dbl, "Y":dbl}, "X Scale":u32, "Y Scale":u32, "Watch Plots":i32[], "Watch All Plots":bool, "Plot Area":i32, "Label Offset":cluster{"X":dbl, "Y":dbl}}
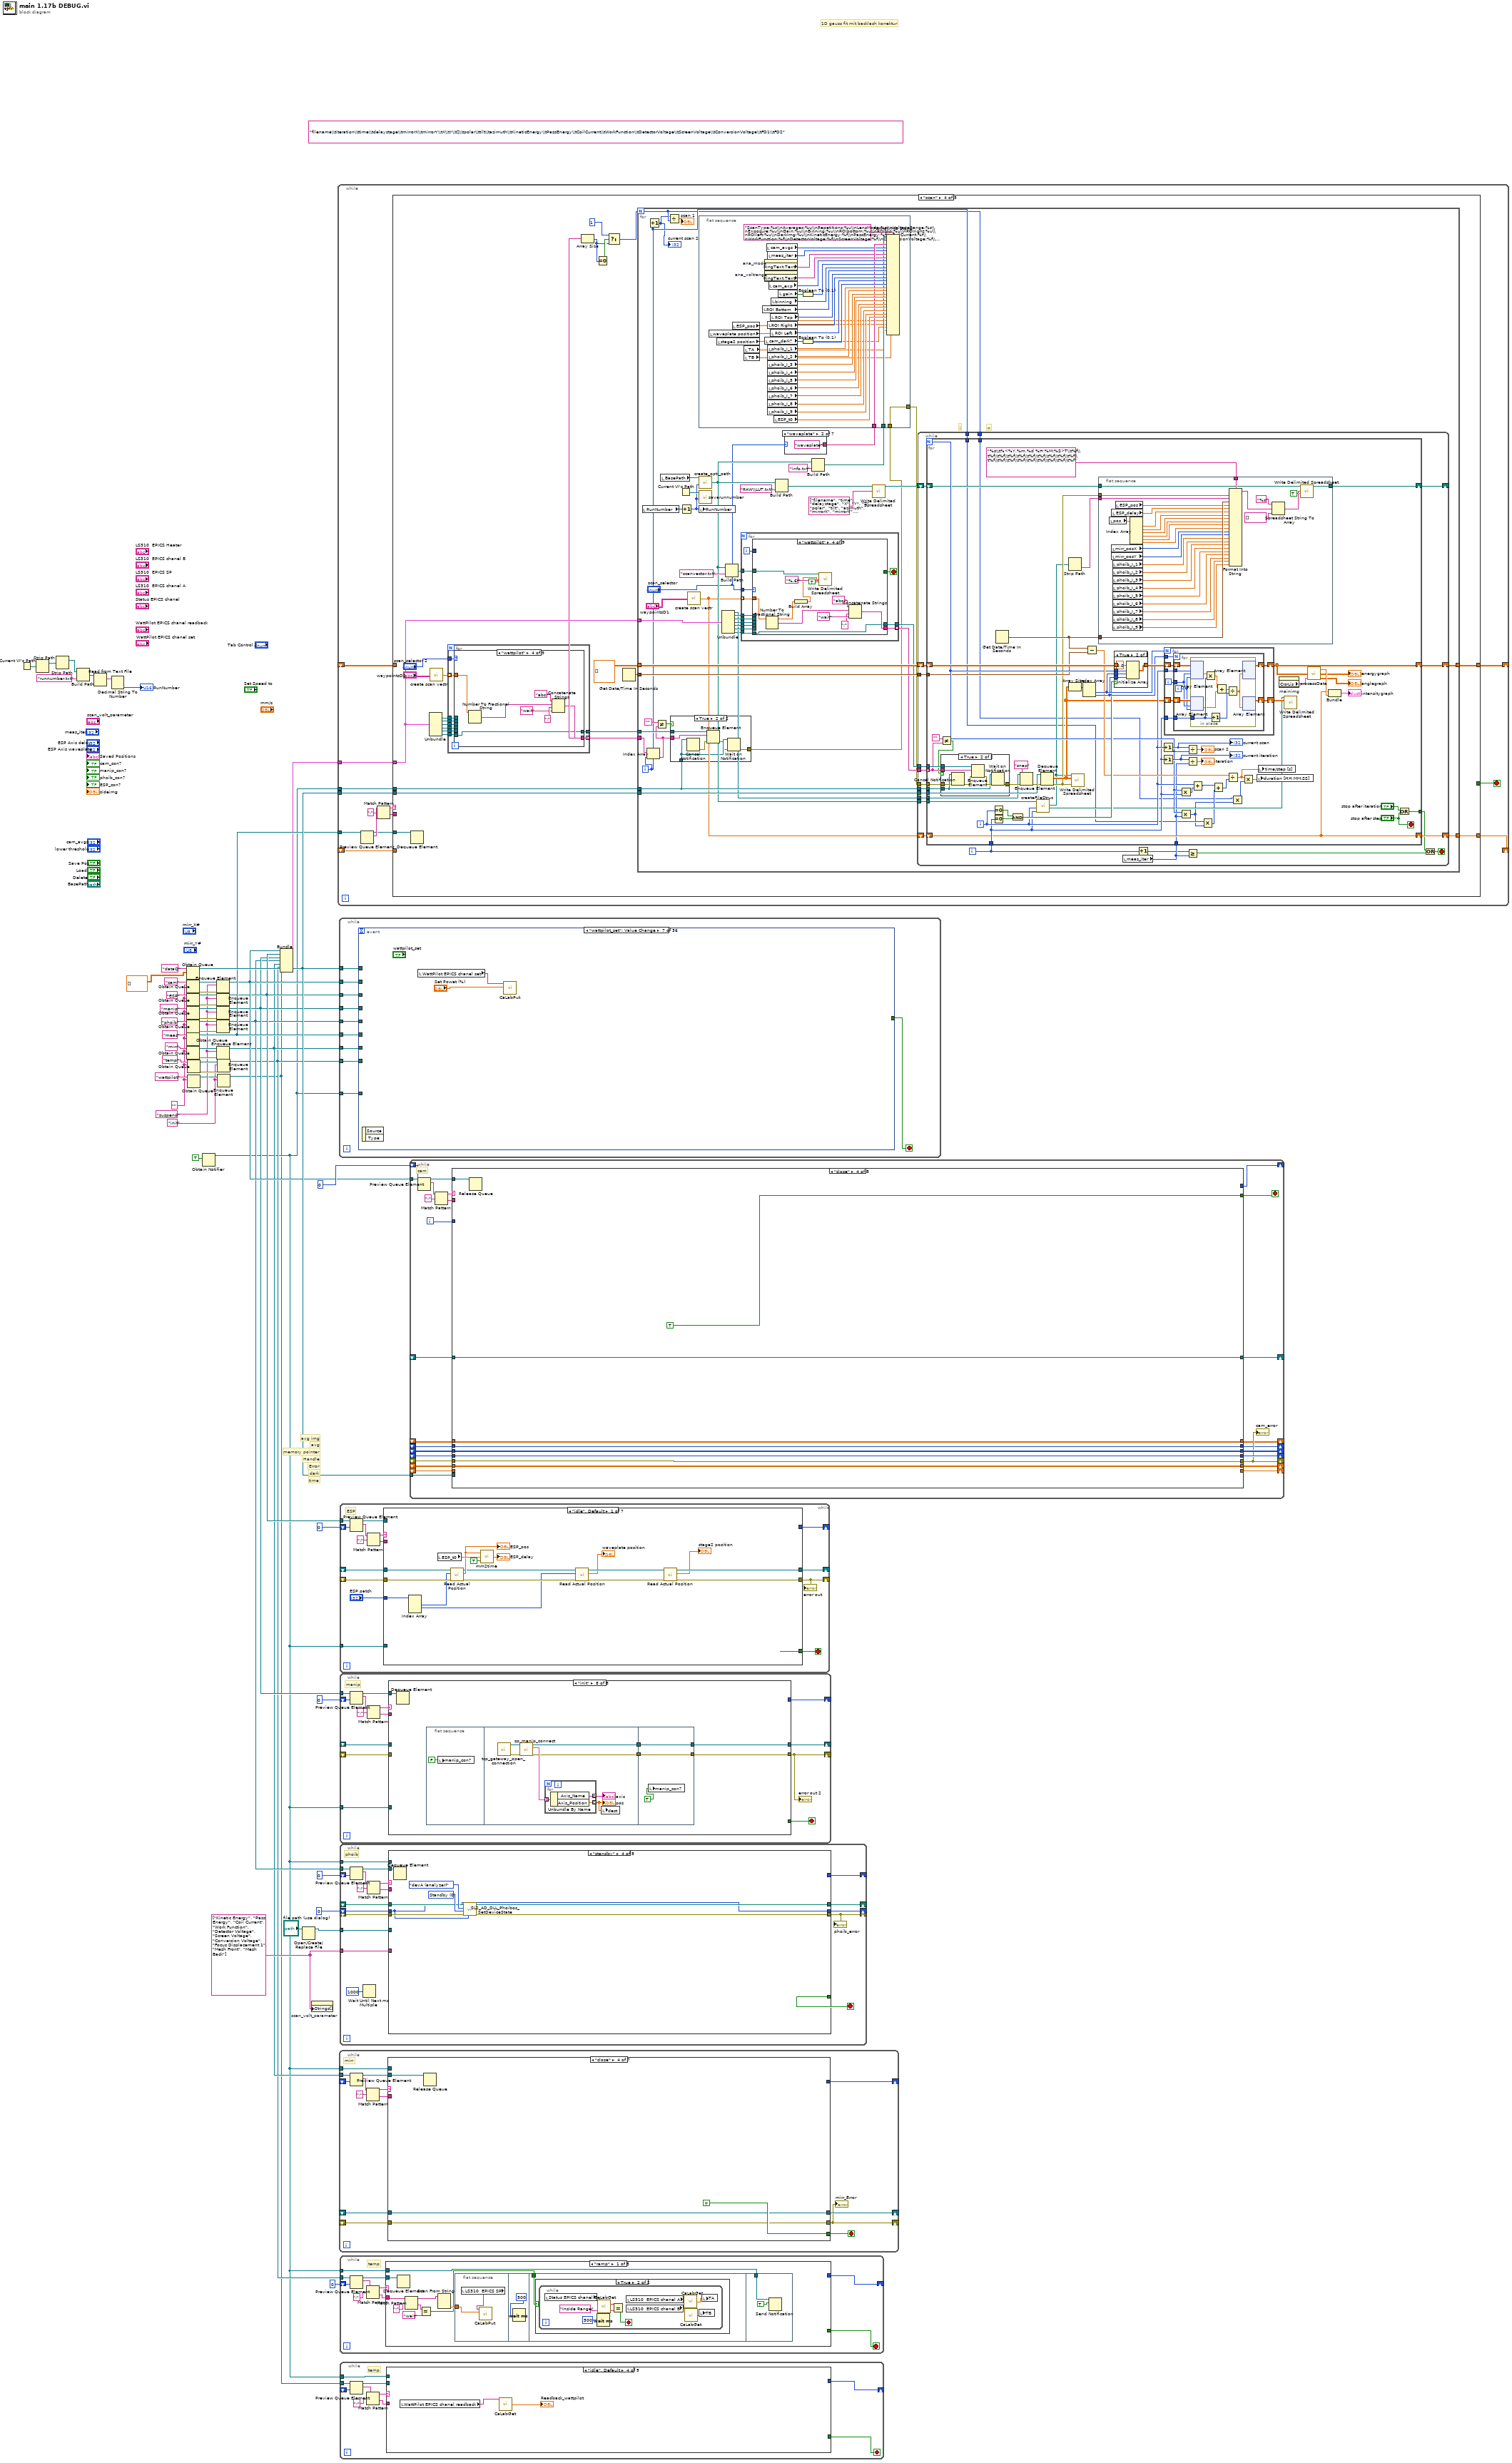
[diagram p0: block diagram]
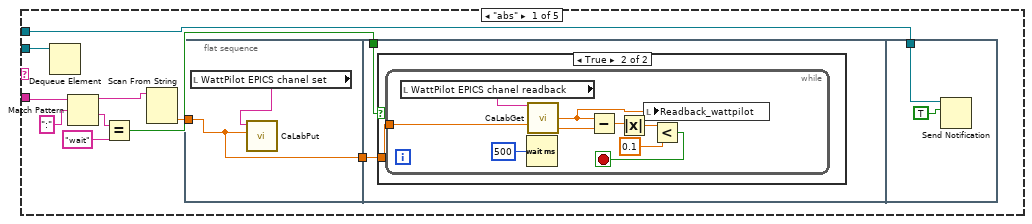
[diagram p2: hidden frame]
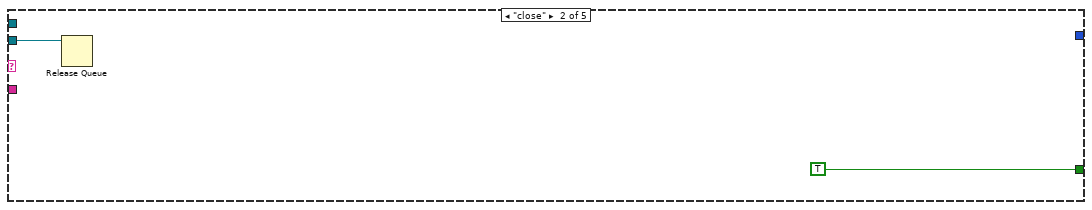
[diagram p4: hidden frame]
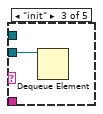
[diagram p5: hidden frame]
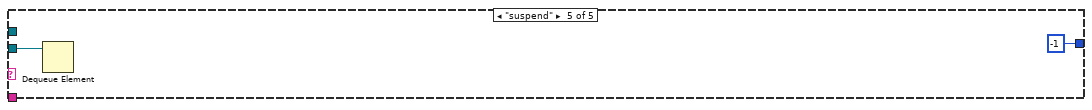
[diagram p6: hidden frame]
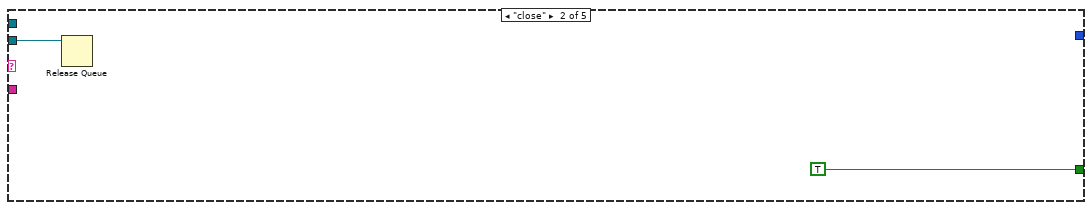
[diagram p8: hidden frame]
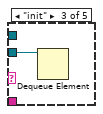
[diagram p9: hidden frame]
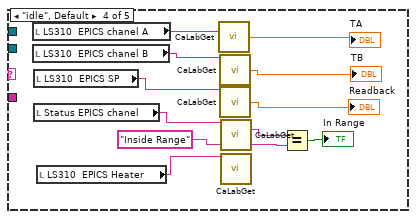
[diagram p10: hidden frame]
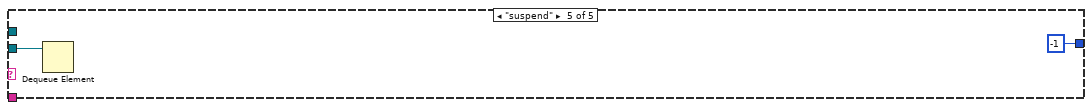
[diagram p11: hidden frame]
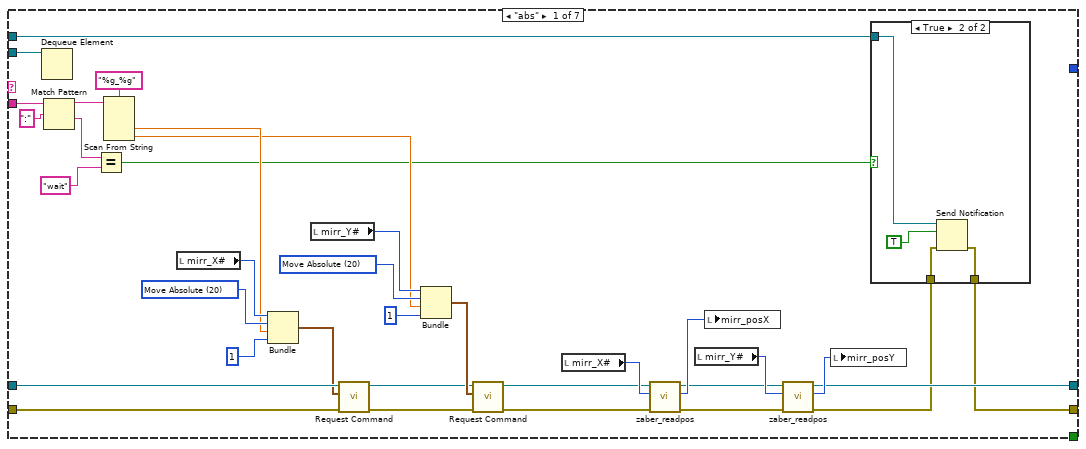
[diagram p12: hidden frame]
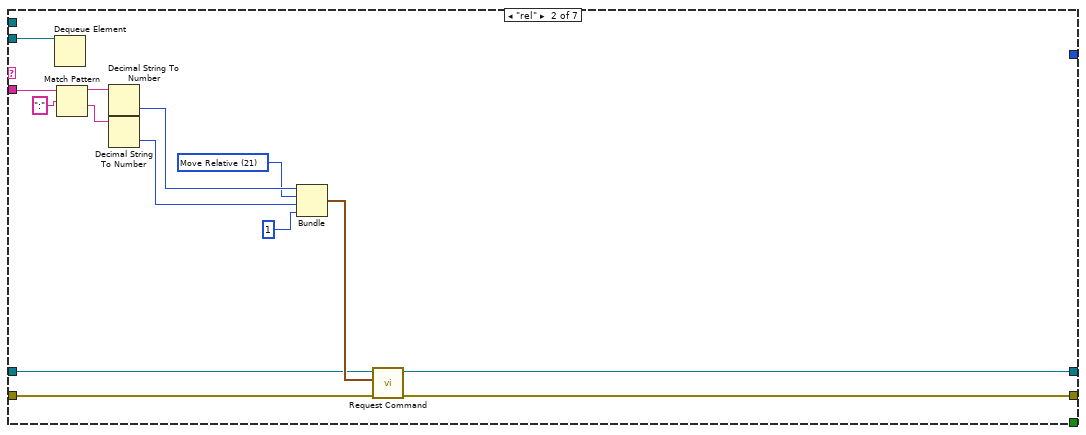
[diagram p14: hidden frame]
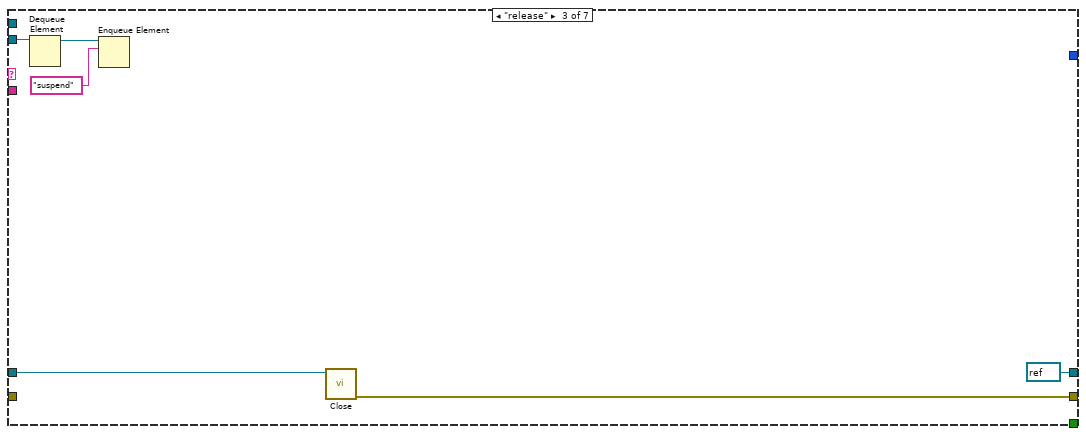
[diagram p15: hidden frame]
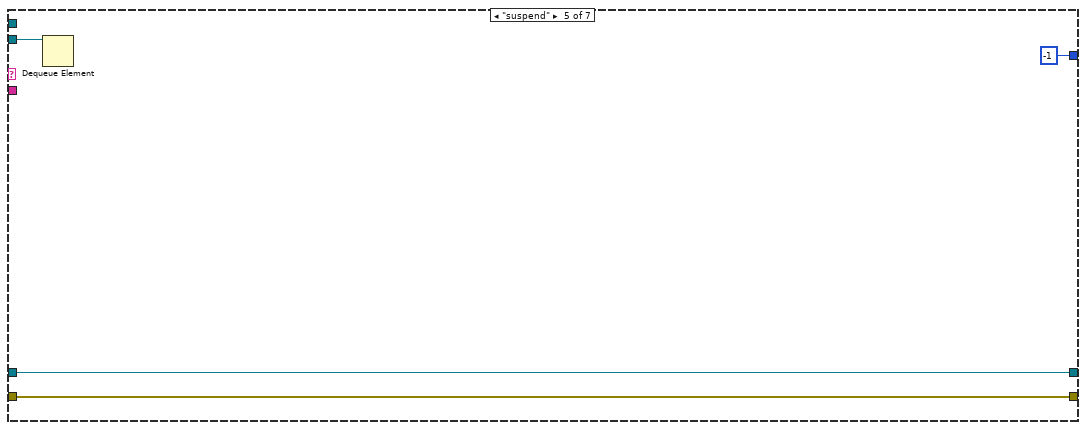
[diagram p16: hidden frame]
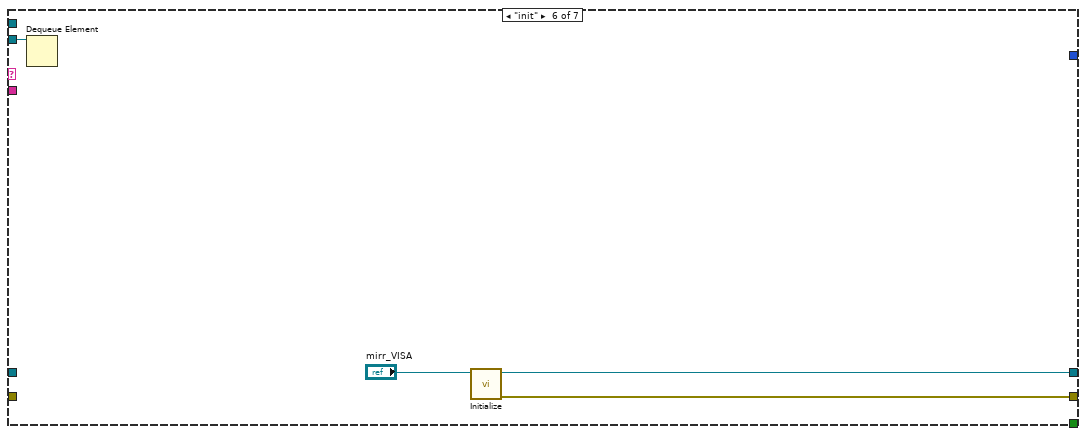
[diagram p17: hidden frame]
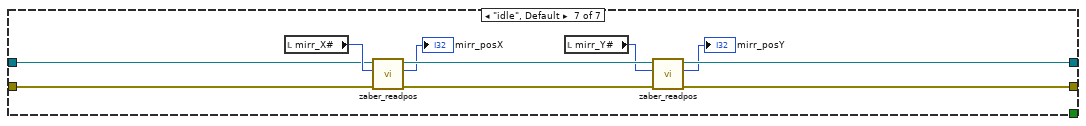
[diagram p18: hidden frame]
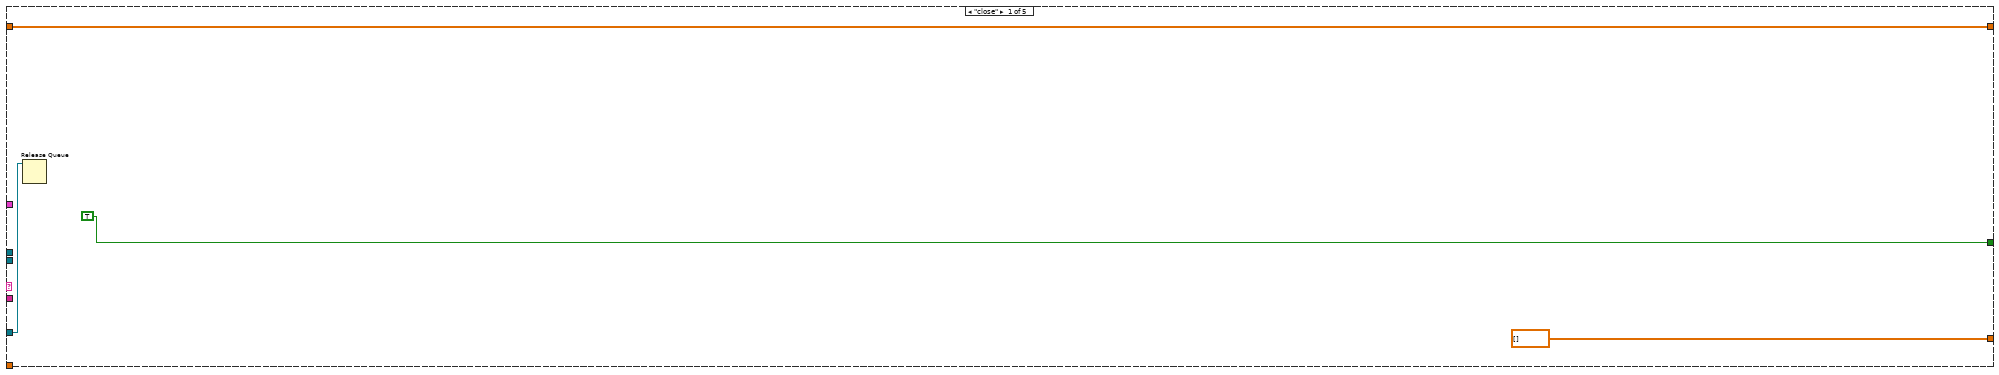
[diagram p19: hidden frame]
diagram:
  (unwired) "filename\\titeration\\ttime\\tdelaystage\\tmirrorX\\tmirrorY\\tX\\tY\\tZ\\tpolar\\ttilt\\tazimuth\\tKineticEnergy\\tPassEnergy\\tCoilCurrent\\tWorkFunction\\tDetectorVoltage\\tScreenVoltage\\tConversionVoltage\\tFD1\\tFD2"
  w20 = string[] ["Kinetic Energy", "Pass Energy", "Coil Current", "Work Function", "Detector Voltage", "Screen Voltage", "Conversion Voltage", "Focus Displacement 1", "Mesh Front", "Mesh Back"]
  w3 = "init" ("name (unnamed)")
  w10 = "suspend" ("name (unnamed)")
  w4 = "" ("name (unnamed)")
  # "1D gauss fit mit backlash korrektur"
  # "avg img"
  # "avg"
  # "time"
  # "dark"
  # "Error"
  # "Handle"
  # "memory pointer"
  n1 = Current VI's Path() -> (path=w28:path)
  n2 = Strip Path(path=w28) -> (stripped path=w32:path)  [unwired: 1 out]
  n3 = Strip Path(path=w32) -> (stripped path=w33:path)  [unwired: 1 out]
  n4 = Build Path(base path=w33, name or relative path="runnumber.txt") -> (appended path=w30:path)
  n5 = Read from Text File(file (use dialog)=w30) -> (text=w31:string)  [unwired: 3 in, 3 out]
  n6 = Decimal String To Number(string=w31) -> (number=→"RunNumber":i32)  [unwired: 2 in, 1 out]
  n7 = Obtain Queue(name (unnamed)="dataQ", element data type=dbl[][] []) -> (queue out=w34:refnum<queue>)  [unwired: 3 in, 2 out]
  n8 = Obtain Queue(name (unnamed)="cam", element data type=w4) -> (queue out=w53:refnum<queue>, error out=w52:errorcluster)  [unwired: 3 in, 1 out]
  n9 = Obtain Queue(name (unnamed)="ESP", element data type=w4) -> (queue out=w50:refnum<queue>, error out=w51:errorcluster)  [unwired: 3 in, 1 out]
  n10 = Obtain Queue(name (unnamed)="manip", element data type=w4) -> (queue out=w47:refnum<queue>, error out=w46:errorcluster)  [unwired: 3 in, 1 out]
  n11 = Obtain Queue(name (unnamed)="phoib", element data type=w4) -> (queue out=w44:refnum<queue>, error out=w45:errorcluster)  [unwired: 3 in, 1 out]
  n12 = Obtain Queue(name (unnamed)="meas", element data type=w4) -> (queue out=w27:refnum<queue>)  [unwired: 3 in, 2 out]
  n13 = Obtain Queue(name (unnamed)="mirr", element data type=w4) -> (queue out=w18:refnum<queue>, error out=w17:errorcluster)  [unwired: 3 in, 1 out]
  n14 = Obtain Queue(name (unnamed)="temp", element data type=w4) -> (queue out=w13:refnum<queue>, error out=w12:errorcluster)  [unwired: 3 in, 1 out]
  n15 = Obtain Queue(name (unnamed)="wattpilot", element data type=w4) -> (queue out=w7:refnum<queue>)  [unwired: 3 in, 2 out]
  n16 = Obtain Notifier(notification data type=TRUE) -> (notifier out=w8:refnum<notifier>)  [unwired: 3 in, 2 out]
  n17 = Enqueue Element(queue=w53, element=w10, error in (no error)=w52) -> (queue out=w25:refnum<queue>)  [unwired: 1 in, 2 out]
  n18 = Enqueue Element(queue=w50, element=w10, error in (no error)=w51) -> (queue out=w24:refnum<queue>)  [unwired: 1 in, 2 out]
  n19 = Enqueue Element(queue=w47, element=w10, error in (no error)=w46) -> (queue out=w23:refnum<queue>)  [unwired: 1 in, 2 out]
  n20 = Enqueue Element(queue=w44, element=w10, error in (no error)=w45) -> (queue out=w22:refnum<queue>)  [unwired: 1 in, 2 out]
  n21 = Enqueue Element(queue=w18, element=w10, error in (no error)=w17) -> (queue out=w15:refnum<queue>)  [unwired: 1 in, 2 out]
  n22 = Enqueue Element(queue=w13, element=w3, error in (no error)=w12) -> (queue out=w9:refnum<queue>)  [unwired: 1 in, 2 out]
  n23 = Enqueue Element(queue=w7, element=w3) -> (queue out=w6:refnum<queue>)  [unwired: 2 in, 2 out]
  n24 = Bundle("queue out"=w25, "queue out"=w24, "queue out"=w23, "queue out"=w22, "queue out"=w15, "queue out"=w9, "queue out"=w6) -> (w26:T4)  [unwired: 1 in]
  n25 = Open/Create/Replace File(file path (use dialog)="file path (use dialog)") -> (refnum out=w1:refnum<file>)  [unwired: 5 in, 2 out]
  n26 = property on="scan_volt_parameter" class="CmbBox"("Strings[]"=w20) -> ()  [unwired: 2 in, 2 out]
  n27 = while {
    tunnel: w34 -> [w68]
    tunnel: w27 -> [w65]
    tunnel: w26 -> [w61]
    shift-right: [w59] -> _
    shift-left: _ -> [w58]
    tunnel: w8 -> [w57]
    shift-right: [w56] -> _
    shift-left: _ -> [w55]
    stop <- w60 stop-if-true
    n28 = Preview Queue Element(queue=w65) -> (queue out=w62:refnum<queue>, element=w67:string)  [unwired: 2 in, 2 out]
    n29 = Match Pattern(string=w67, regular expression=":") -> (before substring=w64:string, after substring=w63:string)  [unwired: 1 in, 2 out]
    n30 = case shown="\"scan\"" w64 {
      tunnel: w68 -> [_ _ w124 w148 _]
      tunnel: w63 -> [_ _ _ _ _]
      tunnel: w62 -> [w72 _ w125 w144 w628]
      tunnel: [TRUE _ _ _ _] -> w60
      tunnel: w61 -> [_ _ w112 w141 _]
      tunnel: [w70 w74 w110 w146 w634] -> w59
      tunnel: w58 -> [w70 w74 w110 _ w634]
      tunnel: w57 -> [_ _ _ w145 _]
      tunnel: [dbl[] [] ("Array") w73 w82 w142 w630] -> w56
      tunnel: w55 -> [_ w73 w82 _ w630]
      frame "close" {
        n31 = Release Queue(queue=w72) -> ()  [unwired: 2 in, 3 out]
      }
      frame "idle", Default {
      }
      frame "single" {
        n32 = Dequeue Element(queue=w125) -> ()  [unwired: 2 in, 4 out]
        n33 = local read "RunNumber"() -> (w119:u16)
        n34 = local read "BasePath"() -> (w120:path)
        n35 = Unbundle(w112) -> ("queue out"=w111:refnum<queue>)  [unwired: 6 out]
        n36 = Increment(x=w119) -> (x+1=w121:u16)
        n37 = Current VI's Path() -> (path=w118:path)
        n38 = call "saverunnumber.vi"("RunNumber"=w121, "VI path"=w118) -> ()  [unwired: 10 in]
        n39 = local write "RunNumber"(w121) -> ()
        n40 = call "create_opti_path.vi"("RunNumber"=w121, "base path"=w120) -> ("Path"=w114:path)  [unwired: 2 in]
        n41 = Enqueue Element(queue=w111, element="snap" ("string")) -> (error out=w122:errorcluster)  [unwired: 2 in, 2 out]
        n42 = Build Path(base path=w114, name or relative path="info.txt") -> (appended path=w83:path)
        n43 = Build Path(base path=w114, name or relative path="AVG\\000.tsv") -> (appended path=w116:path)
        n44 = Dequeue Element(queue=w124, error in (no error)=w122) -> (element=w113:dbl[][])  [unwired: 1 in, 3 out]
        n45 = call-poly <vilib>:"Write Delimited Spreadsheet.vi"("file path (dialog if empty)"=w116, "2D data"=w113) -> ()  [unwired: 12 in, 2 out]
        n46 = local read "ROI Bottom"() -> (w90:i32)
        n47 = property on="ana_mode" class="Enum (strict)"() -> ("RingText.Text"=w105:string)  [unwired: 2 in, 2 out]
        n48 = property on="ana_voltrange" class="Enum (strict)"() -> ("RingText.Text"=w104:string)  [unwired: 2 in, 2 out]
        n49 = local read "cam_dark?"() -> (w86:bool)
        n50 = local read "cam_avgs"() -> (w107:i32)
        n51 = local read "meas_iter"() -> (w106:i32)
        n52 = local read "phoib_I_1"() -> (w103:dbl)
        n53 = local read "phoib_I_2"() -> (w102:dbl)
        n54 = local read "phoib_I_3"() -> (w101:dbl)
        n55 = local read "phoib_I_4"() -> (w100:dbl)
        n56 = local read "phoib_I_5"() -> (w99:dbl)
        n57 = local read "phoib_I_6"() -> (w98:dbl)
        n58 = local read "phoib_I_7"() -> (w97:dbl)
        n59 = local read "phoib_I_8"() -> (w96:dbl)
        n60 = local read "phoib_I_9"() -> (w95:dbl)
        n61 = local read "ROI Right"() -> (w88:i32)
        n62 = local read "cam_exp"() -> (w94:u32)
        n63 = local read "ROI Top"() -> (w89:i32)
        n64 = local read "ROI Left"() -> (w87:i32)
        n65 = local read "binning"() -> (w91:u16)
        n66 = local read "pos"() -> (w81:dbl[])
        n67 = local read "gain"() -> (w93:bool)
        n68 = Get Date/Time In Seconds() -> (seconds since 1Jan1904=w84:timestamp)
        n69 = Boolean To (0,1)(Boolean=w93) -> (0, 1=w92:i16)
        n70 = Boolean To (0,1)(Boolean=w86) -> (0, 1=w85:i16)
        n71 = Index Array(array=w81) -> (element #1=w80:dbl, element #2=w79:dbl, element #3=w78:dbl, element #4=w77:dbl, element #5=w76:dbl, element #6=w75:dbl)  [unwired: 6 in]
        n72 = Format Into String(format string="ScanType=%s\\nAverages=%u\\nRepetitions=%u\\nLensMode=%s\\nVoltageRange=%s\\nKineticEnergy=%f\\nPassEnergy=%f\\nCoilCurrent=%f\\nWorkFunction=%f\\nDetectorVoltage=%f\\nScreenVoltage=%f\\nConversionVoltage=%f\\nFocusDisplacement1=%f\\nFocusDisplacement2=%f\\nExposure=%u\\nGain=%u\\nBinning=%u\\nROIbottom=%u\\nROItop=%u\\nROIright=%u\\nROIleft=%u\\nDarkImg=%u\\nStartTime=%<%Y.%m.%d %H:%M:%S>T\\n\nX=%f\\n\nY=%f\\n\nZ=%f\\n\nPolar=%f\\n\nTilt=%f\\n\nAzimuth=%f\\n", initial string=w83, "single" ("input 1"), w107, w106, w105, w104, w103, w102, w101, w100, w99, w98, w97, w96, w95, w94, w92, w91, w90, w89, w88, w87, w85, w84, w80, w79, w78, w77, w76, w75) -> ()  [unwired: 1 in, 2 out]
      }
      frame "scan" {
        n73 = Dequeue Element(queue=w144) -> ()  [unwired: 2 in, 4 out]
        n74 = Unbundle(w141) -> ("queue out"=w140:refnum<queue>, "queue out"=w139:refnum<queue>, "queue out"=w138:refnum<queue>, "queue out"=w137:refnum<queue>, "queue out"=w136:refnum<queue>, "queue out"=w126:refnum<queue>)  [unwired: 1 out]
        n75 = call "create scan vectr.vi"("Table Control"="waypointsD2") -> ("Array"=w134:dbl[])
        n76 = for {
          tunnel: "scan_selector 2" -> [w158]
          tunnel: w140 -> [w157]
          tunnel: w139 -> [w156]
          tunnel: w138 -> [w155]
          tunnel: w137 -> [w154]
          tunnel: w136 -> [w153]
          tunnel: [w152] -> w131 mode=indexing
          tunnel: [w151] -> w135
          tunnel: w134 -> [w150] mode=indexing
          tunnel: w126 -> [w149]
          n77 = case shown="\"wattpilot\"" w158 {
            tunnel: ["" w162 w173 w184 w190 w201 w219 w233 w245] -> w152
            tunnel: w157 -> [w159 w161 w175 _ w189 _ _ _ _]
            tunnel: w156 -> [_ _ _ _ _ w200 _ _ _]
            tunnel: w155 -> [_ _ _ _ _ _ _ _ w244]
            tunnel: w154 -> [_ _ _ _ _ _ w218 _ _]
            tunnel: w153 -> [_ _ _ _ _ _ _ w232 _]
            tunnel: [w159 w161 w175 w183 w189 w200 w218 w232 w244] -> w151
            tunnel: w150 -> [_ w163 w174 w185 w191 w202 w217 w235 w246]
            tunnel: w149 -> [_ _ _ w183 _ _ _ _ _]
            frame "none", Default {
            }
            frame "delay" {
              w166 = ":" ("string")
              n78 = local read "ESP_t0"() -> (w170:dbl)
              n79 = call "time2mm.vi"("fs[1]/ps[0]"=TRUE, "Offset (mm)"=w170, "time"=w163) -> ("position (mm)"=w171:dbl)
              n80 = Number To Decimal String(number=0) -> (decimal integer string=w168:string)  [unwired: 1 in]
              n81 = Number To Fractional String(number=w171) -> (F-format string=w164:string)  [unwired: 3 in]
              n82 = Concatenate Strings("abs:" ("string"), w168, w166, w164, w166, "wait" ("string")) -> (w162:string)
            }
            frame "waveplate" {
              w181 = ":" ("string")
              n83 = Number To Fractional String(number=w174) -> (F-format string=w176:string)  [unwired: 3 in]
              n84 = Number To Decimal String(number=1) -> (decimal integer string=w179:string)  [unwired: 1 in]
              n85 = Concatenate Strings("abs:" ("string"), w179, w181, w176, w181, "wait" ("string")) -> (w173:string)
            }
            frame "wattpilot" {
              n86 = Number To Fractional String(number=w185) -> (F-format string=w186:string)  [unwired: 3 in]
              n87 = Concatenate Strings("abs:" ("string"), w186, ":" ("string"), "wait" ("string")) -> (w184:string)
            }
            frame "stage2" {
              w196 = ":" ("string")
              n88 = Number To Decimal String(number=2) -> (decimal integer string=w193:string)  [unwired: 1 in]
              n89 = Number To Fractional String(number=w191) -> (F-format string=w192:string)  [unwired: 3 in]
              n90 = Concatenate Strings("abs:" ("string"), w193, w196, w192, w196, "wait" ("string")) -> (w190:string)
            }
            frame "manipulator" {
              n91 = call-poly <vilib>:"Vector Norm.vi"("Input Vector"="scan_manip_deltas 2") -> ("norm"=w203:dbl)  [unwired: 9 in, 1 out]
              n92 = Divide(x="scan_manip_deltas 2", y=w203) -> (x/y=w204:dbl[])
              n93 = Multiply(x=w204, y=w202) -> (x*y=w215:dbl[])
              n94 = Add(x="scan_manip_start 2", y=w215) -> (x+y=w216:dbl[])
              n95 = Index Array(array=w216) -> (element #1=w213:dbl, element #2=w212:dbl, element #3=w211:dbl, element #4=w210:dbl, element #5=w209:dbl, element #6=w208:dbl)  [unwired: 6 in]
              n96 = Format Into String(format string="%g_%g_%g_%g_%g_%g", w213, w212, w211, w210, w209, w208) -> (resulting string=w206:string)  [unwired: 2 in, 1 out]
              n97 = Concatenate Strings("abs:" ("string"), w206, ":wait" ("string")) -> (w201:string)
            }
            frame "mirror" {
              n98 = call-poly <vilib>:"Vector Norm.vi"("Input Vector"="scan_mirr_deltas 2") -> ("norm"=w222:dbl)  [unwired: 9 in, 1 out]
              n99 = Divide(x="scan_mirr_deltas 2", y=w222) -> (x/y=w223:dbl[])
              n100 = Multiply(x=w223, y=w217) -> (x*y=w230:dbl[])
              n101 = Add(x="scan_mirr_start 2", y=w230) -> (x+y=w231:dbl[])
              n102 = Index Array(array=w231) -> (element #1=w227:dbl, element #2=w226:dbl)  [unwired: 2 in]
              n103 = Format Into String(format string="%g_%g", w227, w226) -> (resulting string=w224:string)  [unwired: 2 in, 1 out]
              n104 = Concatenate Strings("abs:" ("string"), w224, ":wait" ("string")) -> (w219:string)
            }
            frame "temperature" {
              n105 = Number To Fractional String(number=w235) -> (F-format string=w237:string)  [unwired: 3 in]
              n106 = Concatenate Strings("ramp:" ("string"), w237) -> (w238:string)
              n107 = case shown="True" "Wait for T 2" {
                tunnel: w238 -> [w240 w243]
                tunnel: ":wait" ("string") -> [_ w242]
                tunnel: [w240 w241] -> w233
                frame False {
                }
                frame True {
                  n108 = Concatenate Strings(w243, w242) -> (w241:string)
                }
              }
            }
            frame "voltage" {
              n109 = Number To Fractional String(number=w246) -> (F-format string=w250:string)  [unwired: 3 in]
              n110 = Concatenate Strings("setsgl:" ("string"), "scan_volt_parameter 2", ":" ("string"), w250) -> (w245:string)
            }
          }
        }
        n111 = Array Size(array=w131) -> (size(s)=w128:i32)
        n112 = Equal To 0?(x=w128) -> (x = 0?=w130:bool)
        n113 = Select(t=1, s=w130, f=w128) -> (s? t:f=w127:i32)
        n114 = Get Date/Time In Seconds() -> (seconds since 1Jan1904=w143:timestamp)
        n115 = for {
          N: w127 -> [w252]
          tunnel: w148 -> [w294]
          tunnel: dbl[][][] [] -> [w293]
          tunnel: [w292] -> w146
          tunnel: w145 -> [w289]
          tunnel: w143 -> [w291]
          tunnel: [w290] -> w142
          tunnel: w141 -> [w281]
          tunnel: w131 -> [w256]
          tunnel: w135 -> [w262]
          i -> [w254]
          # "i"
          # "n"
          n116 = local read "RunNumber"() -> (w274:u16)
          n117 = Index Array(array=w256, index=w254) -> (element=w255:string)
          n118 = Increment(x=w254) -> (x+1=w251:i32)
          "current scan 2" <- w251
          n119 = Not Equal?(x="", y=w255) -> (x != y?=w287:bool)
          n120 = local read "BasePath"() -> (w273:path)
          n121 = Divide(x=w251, y=w252) -> (x/y=→"scan 1":dbl)
          n122 = case shown="True" w287 {
            tunnel: w262 -> [_ w477]
            tunnel: w255 -> [_ w476]
            tunnel: w289 -> [_ w475]
            tunnel: [errorcluster {"status"=FALSE, "code"=0, "source"=""} ("error out") w472] -> w261
            frame False {
            }
            frame True {
              n123 = Cancel Notification(0:w475) -> (11:w474:errorcluster)  [unwired: 1 in, 2 out]
              n124 = Enqueue Element(queue=w477, element=w476, error in (no error)=w474) -> (error out=w473:errorcluster)  [unwired: 1 in, 2 out]
              n125 = Wait on Notification(notifier=w475, error in (no error)=w473) -> (error out=w472:errorcluster)  [unwired: 2 in, 3 out]
            }
          }
          n126 = Current VI's Path() -> (path=w275:path)
          n127 = Increment(x=w274) -> (x+1=w272:u16)
          n128 = call "create scan vectr.vi"("Table Control"="waypointsD1") -> ("Array"=w263:dbl[])
          n129 = flat-sequence {
            tunnel: w277 -> [w309]
            tunnel: w264 -> [w301]
            tunnel: w261 -> [w295]
            tunnel: [w295] -> w260
            frame #0 {
              n130 = local read "waveplate position"() -> (w298:dbl)
              n131 = local read "stage2 position"() -> (w297:dbl)
              n132 = local read "ESP_pos"() -> (w299:dbl)
              n133 = local read "TA"() -> (w300:dbl)
              n134 = local read "TB"() -> (w296:dbl)
              n135 = local read "ROI Bottom"() -> (w313:i32)
              n136 = property on="ana_mode" class="Enum (strict)"() -> ("RingText.Text"=w305:string)  [unwired: 2 in, 2 out]
              n137 = property on="ana_voltrange" class="Enum (strict)"() -> ("RingText.Text"=w306:string)  [unwired: 2 in, 2 out]
              n138 = local read "cam_dark?"() -> (w308:bool)
              n139 = local read "cam_avgs"() -> (w303:i32)
              n140 = local read "meas_iter"() -> (w304:i32)
              n141 = local read "ROI Right"() -> (w315:i32)
              n142 = local read "phoib_I_1"() -> (w318:dbl)
              n143 = local read "phoib_I_2"() -> (w319:dbl)
              n144 = local read "phoib_I_3"() -> (w320:dbl)
              n145 = local read "phoib_I_4"() -> (w321:dbl)
              n146 = local read "phoib_I_5"() -> (w322:dbl)
              n147 = local read "phoib_I_6"() -> (w323:dbl)
              n148 = local read "phoib_I_7"() -> (w324:dbl)
              n149 = local read "phoib_I_8"() -> (w325:dbl)
              n150 = local read "phoib_I_9"() -> (w326:dbl)
              n151 = local read "cam_exp"() -> (w310:u32)
              n152 = local read "ROI Top"() -> (w314:i32)
              n153 = local read "ROI Left"() -> (w316:i32)
              n154 = local read "binning"() -> (w312:u16)
              n155 = local read "ESP_t0"() -> (w327:dbl)
              n156 = local read "gain"() -> (w307:bool)
              n157 = Boolean To (0,1)(Boolean=w307) -> (0, 1=w311:i16)
              n158 = Boolean To (0,1)(Boolean=w308) -> (0, 1=w317:i16)
              n159 = Format Into String(format string="ScanType:%s\\nAverages:%u\\nRepetitions:%u\\nLensMode:%s\\nVoltageRange:%s\\nExposure:%u\\nGain:%u\\nBinning:%u\\nROIbottom:%u\\nROItop:%u\\nROIright:%u\\nROIleft:%u\\nDarkImg:%u\\nKineticEnergy:%f\\nPassEnergy:%f\\nCoilCurrent:%f\\nWorkFunction:%f\\nDetectorVoltage:%f\\nScreenVoltage:%f\\nConversionVoltage:%f\\nFocusDisplacement1:%f\\nFocusDisplacement2:%f\\nTimeZero:%f\\nDelayStage:%f\\nWaveplate:%f\\n2ndStage:%f\\nTempA:%f\\nTempB:%f\\n", initial string=w301, w309, w303, w304, w305, w306, w310, w311, w312, w313, w314, w315, w316, w317, w318, w319, w320, w321, w322, w323, w324, w325, w326, w327, w299, w298, w297, w300, w296) -> ()  [unwired: 1 in, 2 out]
            }
          }
          n160 = call "create_opti_path.vi"("RunNumber"=w272, "base path"=w273) -> ("Path"=w265:path)  [unwired: 2 in]
          n161 = call "saverunnumber.vi"("RunNumber"=w272, "VI path"=w275) -> ()  [unwired: 10 in]
          n162 = local write "RunNumber"(w272) -> ()
          n163 = Unbundle(w281) -> ("queue out"=w280:refnum<queue>, "queue out"=w282:refnum<queue>, "queue out"=w283:refnum<queue>, "queue out"=w284:refnum<queue>, "queue out"=w285:refnum<queue>, "queue out"=w286:refnum<queue>, "queue out"=w253:refnum<queue>)
          n164 = Build Path(base path=w265, name or relative path="scanvector.txt") -> (appended path=w267:path)
          n165 = for {
            tunnel: [w347] -> w279 mode=indexing
            tunnel: [w346] -> w278
            tunnel: w282 -> [w345]
            tunnel: w283 -> [w344]
            tunnel: w284 -> [w343]
            tunnel: w285 -> [w342]
            tunnel: w267 -> [w341]
            tunnel: w286 -> [w340]
            tunnel: w263 -> [w339] mode=indexing
            tunnel: "scan_selector" -> [w337]
            tunnel: w253 -> [w335]
            i -> [w336]
            stop <- w338 stop-if-true
            n166 = case shown="\"wattpilot\"" w337 {
              tunnel: w339 -> [w356 _ w370 w384 w392 w423 w435 w452 w461]
              tunnel: [w354 w364 w367 w381 w393 w411 w432 w450 w465] -> w346
              tunnel: [w359 "" w371 w385 w394 w412 w433 w445 w466] -> w347
              tunnel: w345 -> [w354 w364 w367 _ w393 _ _ _ _]
              tunnel: w344 -> [_ _ _ _ _ w411 _ _ _]
              tunnel: w343 -> [_ _ _ _ _ _ _ _ w465]
              tunnel: w342 -> [_ _ _ _ _ _ w432 _ _]
              tunnel: w341 -> [w349 _ w369 w383 w391 w407 w429 w453 w462]
              tunnel: w340 -> [_ _ _ _ _ _ _ w450 _]
              tunnel: [_ TRUE _ _ _ _ _ _ _] -> w338
              tunnel: w336 -> [_ _ _ _ _ _ _ _ _]
              tunnel: w335 -> [_ _ _ w381 _ _ _ _ _]
              frame "delay" {
                w361 = ":" ("string")
                n167 = local read "ESP_t0"() -> (w355:dbl)
                n168 = call "time2mm.vi"("fs[1]/ps[0]"=TRUE, "Offset (mm)"=w355, "time"=w356) -> ("position (mm)"=w351:dbl)
                n169 = Build Array(w351) -> (w350:dbl[])
                n170 = Number To Decimal String(number=0) -> (decimal integer string=w358:string)  [unwired: 1 in]
                n171 = Number To Fractional String(number=w351) -> (F-format string=w363:string)  [unwired: 3 in]
                n172 = call-poly <vilib>:"Write Delimited Spreadsheet.vi"("file path (dialog if empty)"=w349, "format (%.3f)"="%.6f", "1D data"=w350, "append to file? (F)"=TRUE) -> ()  [unwired: 10 in, 2 out]
                n173 = Concatenate Strings("abs:" ("string"), w358, w361, w363, w361, "wait" ("string")) -> (w359:string)
              }
              frame "none", Default {
              }
              frame "waveplate" {
                w368 = ":" ("string")
                n174 = Number To Fractional String(number=w370) -> (F-format string=w379:string)  [unwired: 3 in]
                n175 = Build Array(w370) -> (w373:dbl[])
                n176 = Number To Decimal String(number=1) -> (decimal integer string=w376:string)  [unwired: 1 in]
                n177 = call-poly <vilib>:"Write Delimited Spreadsheet.vi"("file path (dialog if empty)"=w369, "format (%.3f)"="%.6f", "1D data"=w373, "append to file? (F)"=TRUE) -> ()  [unwired: 10 in, 2 out]
                n178 = Concatenate Strings("abs:" ("string"), w376, w368, w379, w368, "wait" ("string")) -> (w371:string)
              }
              frame "wattpilot" {
                n179 = Number To Fractional String(number=w384) -> (F-format string=w390:string)  [unwired: 3 in]
                n180 = Build Array(w384) -> (w386:dbl[])
                n181 = call-poly <vilib>:"Write Delimited Spreadsheet.vi"("file path (dialog if empty)"=w383, "format (%.3f)"="%.6f", "1D data"=w386, "append to file? (F)"=TRUE) -> ()  [unwired: 10 in, 2 out]
                n182 = Concatenate Strings("abs:" ("string"), w390, ":" ("string"), "wait" ("string")) -> (w385:string)
              }
              frame "stage2" {
                w396 = ":" ("string")
                n183 = Build Array(w392) -> (w401:dbl[])
                n184 = Number To Decimal String(number=2) -> (decimal integer string=w402:string)  [unwired: 1 in]
                n185 = Number To Fractional String(number=w392) -> (F-format string=w403:string)  [unwired: 3 in]
                n186 = call-poly <vilib>:"Write Delimited Spreadsheet.vi"("file path (dialog if empty)"=w391, "format (%.3f)"="%.6f", "1D data"=w401, "append to file? (F)"=TRUE) -> ()  [unwired: 10 in, 2 out]
                n187 = Concatenate Strings("abs:" ("string"), w402, w396, w403, w396, "wait" ("string")) -> (w394:string)
              }
              frame "manipulator" {
                n188 = call-poly <vilib>:"Vector Norm.vi"("Input Vector"="scan_manip_deltas") -> ("norm"=w425:dbl)  [unwired: 9 in, 1 out]
                n189 = Divide(x="scan_manip_deltas", y=w425) -> (x/y=w424:dbl[])
                n190 = Multiply(x=w424, y=w423) -> (x*y=w410:dbl[])
                n191 = Add(x="scan_manip_start", y=w410) -> (x+y=w406:dbl[])
                n192 = call-poly <vilib>:"Write Delimited Spreadsheet.vi"("file path (dialog if empty)"=w407, "format (%.3f)"="%.6f", "1D data"=w406, "append to file? (F)"=TRUE) -> ()  [unwired: 10 in, 2 out]
                n193 = Index Array(array=w406) -> (element #1=w414:dbl, element #2=w415:dbl, element #3=w416:dbl, element #4=w417:dbl, element #5=w418:dbl, element #6=w419:dbl)  [unwired: 6 in]
                n194 = Format Into String(format string="%g_%g_%g_%g_%g_%g", w414, w415, w416, w417, w418, w419) -> (resulting string=w421:string)  [unwired: 2 in, 1 out]
                n195 = Concatenate Strings("abs:" ("string"), w421, ":wait" ("string")) -> (w412:string)
              }
              frame "mirror" {
                n196 = call-poly <vilib>:"Vector Norm.vi"("Input Vector"="scan_mirr_deltas") -> ("norm"=w443:dbl)  [unwired: 9 in, 1 out]
                n197 = Divide(x="scan_mirr_deltas", y=w443) -> (x/y=w442:dbl[])
                n198 = Multiply(x=w442, y=w435) -> (x*y=w431:dbl[])
                n199 = Add(x="scan_mirr_start", y=w431) -> (x+y=w428:dbl[])
                n200 = call-poly <vilib>:"Write Delimited Spreadsheet.vi"("file path (dialog if empty)"=w429, "format (%.3f)"="%.6f", "1D data"=w428, "append to file? (F)"=TRUE) -> ()  [unwired: 10 in, 2 out]
                n201 = Index Array(array=w428) -> (element #1=w438:dbl, element #2=w439:dbl)  [unwired: 2 in]
                n202 = Format Into String(format string="%g_%g", w438, w439) -> (resulting string=w441:string)  [unwired: 2 in, 1 out]
                n203 = Concatenate Strings("abs:" ("string"), w441, ":wait" ("string")) -> (w433:string)
              }
              frame "temperature" {
                n204 = Build Array(w452) -> (w451:dbl[])
                n205 = Number To Fractional String(number=w452) -> (F-format string=w449:string)  [unwired: 3 in]
                n206 = Concatenate Strings("ramp:" ("string"), w449) -> (w447:string)
                n207 = case shown="True" "Wait for T" {
                  tunnel: w447 -> [w456 w459]
                  tunnel: ":wait" ("string") -> [_ w458]
                  tunnel: [w456 w457] -> w445
                  frame False {
                  }
                  frame True {
                    n208 = Concatenate Strings(w459, w458) -> (w457:string)
                  }
                }
                n209 = call-poly <vilib>:"Write Delimited Spreadsheet.vi"("file path (dialog if empty)"=w453, "format (%.3f)"="%.6f", "1D data"=w451, "append to file? (F)"=TRUE) -> ()  [unwired: 10 in, 2 out]
              }
              frame "voltage" {
                n210 = local read "scan_volt_parameter"() -> (w469:string)
                n211 = Build Array(w461) -> (w460:dbl[])
                n212 = Number To Fractional String(number=w461) -> (F-format string=w467:string)  [unwired: 3 in]
                n213 = Concatenate Strings("setsgl:" ("string"), w469, ":" ("string"), w467) -> (w466:string)
                n214 = call-poly <vilib>:"Write Delimited Spreadsheet.vi"("file path (dialog if empty)"=w462, "format (%.3f)"="%.6f", "1D data"=w460, "append to file? (F)"=TRUE) -> ()  [unwired: 10 in, 2 out]
              }
            }
          }
          n215 = Build Path(base path=w265, name or relative path="RAW\\LUT.txt") -> (appended path=w276:path)
          n216 = case shown="\"waveplate\"" "scan_selector" {
            tunnel: ["delay" ("input 1") "waveplate" ("input 1") "stage2" ("input 1") "manipulator" ("input 1") "temperature" "mirror" ("input 1") "voltage" ("input 1")] -> w277
            frame "delay", Default {
            }
            frame "waveplate" {
            }
            frame "stage2" {
            }
            frame "manipulator" {
            }
            frame "temperature" {
            }
            frame "mirror" {
            }
            frame "voltage" {
            }
          }
          n217 = Build Path(base path=w265, name or relative path="info.txt") -> (appended path=w264:path)
          n218 = call-poly <vilib>:"Write Delimited Spreadsheet.vi"("file path (dialog if empty)"=w276, "1D data"=string[] ["filename", "time", "delaystage", "X", "Y", "Z", "polar", "tilt", "azimuth", "mirrorX", "mirrorY", "KineticEnergy", "PassEnergy", "CoilCurrent", "WorkFunction", "DetectorVoltage", "ScreenVoltage", "ConversionVoltage", "FD1", "FD2"]) -> ("new file path (Not A Path if cancelled)"=w268:path)  [unwired: 12 in, 1 out]
          n219 = while {
            tunnel: w265 -> [w499]
            tunnel: w294 -> [w498]
            shift-right: [w497] -> w292
            shift-left: w293 -> [w496]
            tunnel: w289 -> [w495]
            tunnel: w291 -> [w494]
            tunnel: w278 -> [w493]
            tunnel: w279 -> [w492]
            tunnel: w280 -> [w491]
            shift-right: [w489] -> _
            shift-left: w268 -> [w490]
            shift-right: [w488] -> w290
            shift-left: w263 -> [w487]
            tunnel: w260 -> [w480]
            tunnel: w252 -> [w479]
            tunnel: w254 -> [w478]
            i -> [w486]
            stop <- w483 stop-if-true
            n220 = local read "meas_iter"() -> (w485:i32)
            n221 = for {
              N -> [w536]
              tunnel: w499 -> [w534]
              tunnel: w498 -> [w555]
              tunnel: w486 -> [w532]
              shift-right: [w546] -> w497
              shift-left: w496 -> [w551]
              tunnel: w495 -> [w548]
              tunnel: w494 -> [w535]
              tunnel: w493 -> [w528]
              tunnel: w492 -> [w508] mode=indexing
              tunnel: w491 -> [w527]
              shift-right: [w523] -> w489
              shift-left: w490 -> [w524]
              shift-right: [w519] -> w488
              shift-left: w487 -> [w519]
              tunnel: [w516] -> w482
              tunnel: w485 -> [w515]
              tunnel: w480 -> [w510]
              tunnel: w479 -> [w502]
              tunnel: w478 -> [w506]
              i -> [w533]
              stop <- "stop after step" stop-if-true
              n222 = Not Equal?(x="", y=w508) -> (x != y?=w507:bool)
              n223 = case shown="True" w507 {
                tunnel: [w560 w566] -> w550
                tunnel: w548 -> [_ w564]
                tunnel: w528 -> [_ w563]
                tunnel: w508 -> [_ w562]
                tunnel: w510 -> [w560 w561]
                frame False {
                }
                frame True {
                  n224 = Cancel Notification(0:w564, 3:w561) -> (11:w565:errorcluster)  [unwired: 2 out]
                  n225 = Enqueue Element(queue=w563, element=w562, error in (no error)=w565) -> (error out=w567:errorcluster)  [unwired: 1 in, 2 out]
                  n226 = Wait on Notification(notifier=w564, error in (no error)=w567) -> (error out=w566:errorcluster)  [unwired: 2 in, 3 out]
                }
              }
              n227 = Equal To 0?(x=w533) -> (x = 0?=w554:bool)
              n228 = Equal To 0?(x=w532) -> (x = 0?=w553:bool)
              n229 = Get Date/Time In Seconds() -> (seconds since 1Jan1904=w525:timestamp)
              n230 = And(x=w554, y=w553) -> (x .and. y?=w552:bool)
              n231 = Enqueue Element(queue=w527, element="snap", error in (no error)=w550) -> (error out=w549:errorcluster)  [unwired: 1 in, 2 out]
              n232 = call "createFileStruc.vi"("i_iter"=w532, "i_delay"=w533, "meas_path"=w534) -> ("AVG file"=w529:path, "RAW file"=w521:path)  [unwired: 7 in]
              n233 = Dequeue Element(queue=w555, error in (no error)=w549) -> (element=w531:dbl[][], error out=w522:errorcluster)  [unwired: 1 in, 2 out]
              n234 = Strip Path(path=w521) -> (name=w520:string)  [unwired: 1 out]
              n235 = Array Size(array=w531) -> (size(s)=w559:i32[])
              n236 = call-poly <vilib>:"Write Delimited Spreadsheet.vi"("file path (dialog if empty)"=w521, "2D data"=w531, "error in (no error)"=w522) -> ()  [unwired: 11 in, 2 out]
              n237 = Index Array(array=w559) -> (element #1=w557:i32, element #2=w556:i32)  [unwired: 2 in]
              n238 = Subtract(x=w525, y=w535) -> (x-y=w538:dbl)
              n239 = flat-sequence {
                tunnel: "%s\\t%<%Y.%m.%d %H:%M:%S>T\\t%f\\t%f\\t%f\\t%f\\t%f\\t%f\\t%f\\t%f\\t%f\\t%f\\t%f\\t%f\\t%f\\t%f\\t%f\\t%f\\t%f\\t%f\\t%f" -> [w597]
                tunnel: w525 -> [w596]
                tunnel: w524 -> [w573]
                tunnel: [w572] -> w523
                tunnel: w522 -> [w569]
                tunnel: w520 -> [w568]
                frame #0 {
                  n240 = local read "pos"() -> (w598:dbl[])
                  n241 = local read "mirr_posX"() -> (w585:i32)
                  n242 = local read "mirr_posY"() -> (w586:i32)
                  n243 = local read "ESP_delay"() -> (w578:dbl)
                  n244 = local read "phoib_I_1"() -> (w587:dbl)
                  n245 = local read "phoib_I_2"() -> (w588:dbl)
                  n246 = local read "phoib_I_3"() -> (w589:dbl)
                  n247 = local read "phoib_I_4"() -> (w590:dbl)
                  n248 = local read "phoib_I_5"() -> (w591:dbl)
                  n249 = local read "phoib_I_6"() -> (w592:dbl)
                  n250 = local read "phoib_I_7"() -> (w593:dbl)
                  n251 = local read "phoib_I_8"() -> (w594:dbl)
                  n252 = local read "phoib_I_9"() -> (w595:dbl)
                  n253 = local read "ESP_pos"() -> (w577:dbl)
                  n254 = Index Array(array=w598) -> (element #1=w579:dbl, element #2=w580:dbl, element #3=w581:dbl, element #4=w582:dbl, element #5=w583:dbl, element #6=w584:dbl)  [unwired: 6 in]
                  n255 = Format Into String(format string=w597, error in=w569, w568, w596, w577, w578, w579, w580, w581, w582, w583, w584, w585, w586, w587, w588, w589, w590, w591, w592, w593, w594, w595) -> (resulting string=w575:string)  [unwired: 1 in, 1 out]
                  n256 = Spreadsheet String To Array(format string="%s", spreadsheet string=w575, array type (2D Dbl)=string[] []) -> (array=w571:string[])  [unwired: 1 in]
                  n257 = call-poly <vilib>:"Write Delimited Spreadsheet.vi"("file path (dialog if empty)"=w573, "1D data"=w571, "append to file? (F)"=TRUE) -> ("new file path (Not A Path if cancelled)"=w572:path)  [unwired: 11 in, 1 out]
                }
              }
              n258 = case shown="True" w552 {
                tunnel: w536 -> [_ w604]
                tunnel: [w599 w602] -> w558
                tunnel: w551 -> [w599 _]
                tunnel: w557 -> [_ w601]
                tunnel: w556 -> [_ w600]
                frame False {
                }
                frame True {
                  n259 = Initialize Array(0.0 ("element"), w604, w601, w600) -> (w602:dbl[][][])
                }
              }
              n260 = Increment(x=w533) -> (x+1=w542:i32)
              "current scan" <- w542
              n261 = Increment(x=w532) -> (x+1=w541:i32)
              "current iteration" <- w541
              n262 = for {
                N: w557 -> [_]
                tunnel: w533 -> [w611]
                shift-right: [w609] -> w546
                shift-left: w558 -> [w612]
                tunnel: w532 -> [w607]
                shift-right: [w606] -> w530
                shift-left: w531 -> [w608]
                tunnel: w556 -> [w605]
                i -> [w610]
                n263 = for {
                  N: w605 -> [_]
                  tunnel: w611 -> [w619]
                  tunnel: w610 -> [w616]
                  shift-right: [w618] -> w609
                  shift-left: w612 -> [w620]
                  tunnel: w607 -> [w614]
                  shift-right: [w613] -> w606
                  shift-left: w608 -> [w617]
                  i -> [w615]
                  n264 = in-place {
                    in-place-border: w614 -> [w626]
                    n265 = in-place-array #1(w620, w619, w616, w615) -> (w627:dbl)
                    n266 = in-place-array #2(w617, w616, w615) -> (w624:dbl)
                    n267 = Multiply(x=w627, y=w626) -> (x*y=w625:dbl)
                    n268 = Increment(x=w626) -> (x+1=w622:i32)
                    n269 = Add(x=w625, y=w624) -> (x+y=w623:dbl)
                    n270 = Divide(x=w623, y=w622) -> (x/y=w621:dbl)
                    n271 = in-place-array #1(w621) -> (w618:dbl[][][])  [unwired: 3 out]
                    n272 = in-place-array #2(w621) -> (w613:dbl[][])  [unwired: 2 out]
                  }
                }
              }
              n273 = Multiply(x=w536, y=w532) -> (x*y=w537:i32)
              n274 = Multiply(x=w536, y=w515) -> (x*y=w501:i32)
              n275 = Divide(x=w542, y=w536) -> (x/y=→"scan 2":dbl)
              n276 = Divide(x=w541, y=w515) -> (x/y=→"iteration":dbl)
              n277 = Add(x=w533, y=w537) -> (x+y=w504:i32)
              n278 = Multiply(x=w506, y=w501) -> (x*y=w505:i32)
              n279 = Add(x=w504, y=w505) -> (x+y=w503:i32)
              n280 = Divide(x=w538, y=w503) -> (x/y=w511:dbl)
              n281 = Multiply(x=w502, y=w501) -> (x*y=w500:i32)
              n282 = Multiply(x=w511, y=w500) -> (x*y=w514:dbl)
              n283 = local write "duration [HH:MM:SS]"(w514) -> ()
              n284 = local write "time/step [s]"(w511) -> ()
              n285 = property on="mainimg" class="IntGraph (strict)"() -> ("CrsrLis"=w545:T5)  [unwired: 2 in, 2 out]
              n286 = call-poly <vilib>:"Write Delimited Spreadsheet.vi"("file path (dialog if empty)"=w529, "2D data"=w530) -> ()  [unwired: 12 in, 2 out]
              n287 = call "processData.vi"("Cursor List"=w545, "data in"=w546) -> ("Angle Chart"=→"anglegraph":dbl[][], "Energy Chart"=→"energygraph":dbl[][], "Intensity Chart"=w544:dbl[])  [unwired: 1 in]
              n288 = Bundle("Array"=w519, "Intensity Chart"=w544) -> (→"intensitygraph":cluster{"Array":dbl[], "Intensity Chart":dbl[]})  [unwired: 1 in]
              n289 = Or(x="stop after iteration", y="stop after step") -> (x .or. y?=w516:bool)
            }
            n290 = Increment(x=w486) -> (x+1=w484:i32)
            n291 = Greater Or Equal?(x=w484, y=w485) -> (x >= y?=w481:bool)
            n292 = Or(x=w482, y=w481) -> (x .or. y?=w483:bool)
          }
        }
      }
      frame "refresh" {
        n293 = Dequeue Element(queue=w628) -> ()  [unwired: 2 in, 4 out]
        n294 = property on="mainimg" class="IntGraph (strict)"() -> ("CrsrLis"=w635:T5)  [unwired: 2 in, 2 out]
        n295 = call "processData.vi"("Cursor List"=w635, "data in"=w634) -> ("Angle Chart"=w632:dbl[][], "Energy Chart"=w633:dbl[][], "Intensity Chart"=w629:dbl[])  [unwired: 1 in]
        n296 = Bundle("Array"=w630, "Intensity Chart"=w629) -> (w631:cluster{"Array":dbl[], "Intensity Chart":dbl[]})  [unwired: 1 in]
        n297 = local write "energygraph"(w633) -> ()
        n298 = local write "intensitygraph"(w631) -> ()
        n299 = local write "anglegraph"(w632) -> ()
      }
    }
  }
  n300 = while {
    tunnel: w25 -> [w644]
    tunnel: w24 -> [w643]
    tunnel: w23 -> [w642]
    tunnel: w22 -> [w641]
    tunnel: w27 -> [w639]
    tunnel: w34 -> [w640]
    tunnel: w8 -> [w638]
    tunnel: w15 -> [w637]
    tunnel: w9 -> [w636]
    stop <- w645 stop-if-true
    n301 = event shown="[6] \"wattpilot_set\": Value Change" {
      selector: _ -> [_ _ _ _ _ _ _ _ _ _ _ _ _ _ _ _ _ _ _ _ _ _ _ _ _ _ _ _ _ _ _ _ _ _ _ _]
      dyn-events: _ -> [_ _ _ _ _ _ _ _ _ _ _ _ _ _ _ _ _ _ _ _ _ _ _ _ _ _ _ _ _ _ _ _ _ _ _ _]
      timeout: _ -> [_ _ _ _ _ _ _ _ _ _ _ _ _ _ _ _ _ _ _ _ _ _ _ _ _ _ _ _ _ _ _ _ _ _ _ _]
      tunnel: [_ TRUE _ _ _ _ _ _ _ _ _ _ _ _ _ _ _ _ _ _ _ _ _ _ _ _ _ _ _ _ _ _ _ _ _ _] -> w645
      tunnel: w644 -> [_ w660 w672 _ _ _ _ _ _ _ w702 w704 _ _ _ _ _ _ _ _ _ _ _ _ _ _ _ _ _ _ _ _ _ _ _ _]
      tunnel: w643 -> [_ w659 _ w676 _ _ _ _ _ _ _ _ _ _ _ _ _ _ _ _ _ _ _ w783 _ _ w805 _ _ _ _ _ _ _ _ _]
      tunnel: w642 -> [_ w658 _ _ w682 _ _ _ _ _ _ _ _ _ _ _ _ _ _ _ w757 w773 w775 _ _ _ _ _ _ _ _ _ _ _ _ _]
      tunnel: w641 -> [_ w657 _ _ _ _ _ w692 w698 w699 _ _ _ _ _ _ _ _ _ _ _ _ _ _ _ _ _ _ _ _ _ _ _ _ _ _]
      tunnel: w640 -> [_ w665 _ _ _ _ _ _ _ _ _ _ _ _ _ _ _ _ _ _ _ _ _ _ _ _ _ _ _ _ _ _ _ _ _ _]
      tunnel: w639 -> [_ w656 _ _ _ _ _ _ _ _ _ _ w706 w708 _ _ _ _ _ _ _ _ _ _ _ _ _ _ _ _ _ _ _ w829 _ _]
      tunnel: w638 -> [_ w664 _ _ _ _ _ _ _ _ _ _ _ _ _ _ _ _ _ _ _ _ _ _ _ _ _ _ _ _ _ _ _ _ _ _]
      tunnel: w637 -> [_ w655 _ _ _ _ _ _ _ _ _ _ _ _ _ w731 _ _ _ _ _ _ _ _ _ _ _ _ _ _ _ _ _ _ w831 w852]
      tunnel: w636 -> [_ w648 _ _ _ _ _ _ _ _ _ _ _ _ _ _ _ _ _ _ _ _ _ _ _ _ _ _ _ _ _ _ _ _ _ _]
      event Timeout {
        n302 = event-data() -> ()  [unwired: 1 in, 1 out]
      }
      event "main_close": Value Change {
        w646 = "close" ("element")
        w661 = "release" ("element")
        n303 = event-data() -> ()  [unwired: 1 in, 1 out]
        n304 = Flush Queue(queue=w660) -> (queue out=w654:refnum<queue>)  [unwired: 1 in, 2 out]
        n305 = Flush Queue(queue=w659) -> (queue out=w653:refnum<queue>)  [unwired: 1 in, 2 out]
        n306 = Flush Queue(queue=w658) -> (queue out=w652:refnum<queue>)  [unwired: 1 in, 2 out]
        n307 = Flush Queue(queue=w657) -> (queue out=w651:refnum<queue>)  [unwired: 1 in, 2 out]
        n308 = Flush Queue(queue=w656) -> (queue out=w650:refnum<queue>)  [unwired: 1 in, 2 out]
        n309 = Flush Queue(queue=w655) -> (queue out=w649:refnum<queue>)  [unwired: 1 in, 2 out]
        n310 = Flush Queue(queue=w648) -> (queue out=w647:refnum<queue>)  [unwired: 1 in, 2 out]
        n311 = Release Notifier(notifier=w664) -> ()  [unwired: 2 in, 3 out]
        n312 = Release Queue(queue=w665) -> ()  [unwired: 2 in, 3 out]
        n313 = Enqueue Element(queue=w654, element=w661) -> (queue out=w669:refnum<queue>)  [unwired: 2 in, 2 out]
        n314 = Enqueue Element(queue=w653, element=w661) -> (queue out=w668:refnum<queue>)  [unwired: 2 in, 2 out]
        n315 = Enqueue Element(queue=w652, element=w661) -> (queue out=w667:refnum<queue>)  [unwired: 2 in, 2 out]
        n316 = Enqueue Element(queue=w651, element=w661) -> (queue out=w666:refnum<queue>)  [unwired: 2 in, 2 out]
        n317 = Enqueue Element(queue=w649, element=w661) -> (queue out=w663:refnum<queue>, error out=w662:errorcluster)  [unwired: 2 in, 1 out]
        n318 = Enqueue Element(queue=w669, element=w646) -> ()  [unwired: 2 in, 3 out]
        n319 = Enqueue Element(queue=w668, element=w646) -> ()  [unwired: 2 in, 3 out]
        n320 = Enqueue Element(queue=w667, element=w646) -> ()  [unwired: 2 in, 3 out]
        n321 = Enqueue Element(queue=w666, element=w646) -> ()  [unwired: 2 in, 3 out]
        n322 = Enqueue Element(queue=w650, element=w646) -> ()  [unwired: 2 in, 3 out]
        n323 = Enqueue Element(queue=w663, element=w646, error in (no error)=w662) -> ()  [unwired: 1 in, 3 out]
        n324 = Enqueue Element(queue=w647, element=w646) -> ()  [unwired: 2 in, 3 out]
      }
      event "cam_release", "cam_init": Value Change {
        n325 = event-data() -> ()  [unwired: 1 in, 2 out]
        n326 = Select(t="init" ("name (unnamed)"), s="cam_init", f="release" ("name (unnamed)")) -> (s? t:f=w671:string)
        n327 = Enqueue Element(queue=w672, element=w671) -> ()  [unwired: 2 in, 3 out]
      }
      event "ESP_release", "ESP_init": Value Change {
        n328 = event-data() -> ()  [unwired: 1 in, 2 out]
        n329 = Select(t="init" ("name (unnamed)"), s="ESP_init", f="release" ("name (unnamed)")) -> (s? t:f=w680:string)
        n330 = Enqueue Element(queue=w676, element=w680) -> ()  [unwired: 2 in, 3 out]
      }
      event "manip_init", "manip_release": Value Change {
        n331 = event-data() -> ()  [unwired: 1 in, 2 out]
        n332 = Flush Queue(queue=w682) -> (queue out=w681:refnum<queue>)  [unwired: 1 in, 2 out]
        n333 = Select(t="init" ("name (unnamed)"), s="manip_init", f="release" ("name (unnamed)")) -> (s? t:f=w684:string)
        n334 = Enqueue Element(queue=w681, element=w684) -> ()  [unwired: 2 in, 3 out]
      }
      event "setpoint_set": Value Change {
        n335 = event-data() -> ()  [unwired: 1 in, 2 out]
        n336 = local read "LS310  EPICS SP"() -> (w688:string)
        n337 = call-poly <userlib>:"CaLabPut.vi"("Value"="Setpoint", "PV Name"=w688) -> ()  [unwired: 6 in, 4 out]
      }
      event "wattpilot_set": Value Change {
        n338 = event-data() -> ()  [unwired: 1 in, 2 out]
        n339 = local read "WattPilot EPICS chanel set"() -> (w690:string)
        n340 = call-poly <userlib>:"CaLabPut.vi"("Value"="Set Powet (%)", "PV Name"=w690) -> ()  [unwired: 6 in, 4 out]
      }
      event "phoib_release", "phoib_init": Value Change {
        n341 = event-data() -> ()  [unwired: 1 in, 2 out]
        n342 = Flush Queue(queue=w692) -> (queue out=w691:refnum<queue>)  [unwired: 1 in, 2 out]
        n343 = Select(t="init" ("name (unnamed)"), s="phoib_init", f="release" ("name (unnamed)")) -> (s? t:f=w694:string)
        n344 = Enqueue Element(queue=w691, element=w694) -> ()  [unwired: 2 in, 3 out]
      }
      event "phoib_standby": Value Change {
        n345 = event-data() -> ()  [unwired: 1 in, 2 out]
        n346 = Enqueue Element(queue=w698, element="standby") -> ()  [unwired: 2 in, 3 out]
      }
      event "phoib_set": Value Change {
        n347 = event-data() -> ()  [unwired: 1 in, 2 out]
        n348 = Enqueue Element(queue=w699, element="set") -> ()  [unwired: 2 in, 3 out]
      }
      event "cam_dark": Value Change {
        n349 = event-data() -> ()  [unwired: 1 in, 2 out]
        n350 = Enqueue Element(queue=w702, element="dark") -> ()  [unwired: 2 in, 3 out]
      }
      event "ROI Left", "ROI Right", "ROI Top", "ROI Bottom", "cam_exp", "binning", "gain": Value Change {
        n351 = event-data() -> ()  [unwired: 1 in, 1 out]
        n352 = Enqueue Element(queue=w704, element="set") -> ()  [unwired: 2 in, 3 out]
      }
      event "cam_saveimg": Value Change {
        n353 = event-data() -> ()  [unwired: 1 in, 1 out]
        n354 = Enqueue Element(queue=w706, element="single") -> ()  [unwired: 2 in, 3 out]
      }
      event "scan_go": Value Change {
        n355 = event-data() -> ()  [unwired: 1 in, 1 out]
        n356 = Enqueue Element(queue=w708, element="scan") -> ()  [unwired: 2 in, 3 out]
      }
      event "meas_iter", "waypointsD1", "waypointsD2": Value Change {
        n357 = event-data() -> ()  [unwired: 1 in, 6 out]
        n358 = local read "waypointsD2"() -> (w719:string[][])
        n359 = local read "waypointsD1"() -> (w729:string[][])
        n360 = call "create scan vectr.vi"("Table Control"=w719) -> ("Array"=w718:dbl[])
        n361 = call "create scan vectr.vi"("Table Control"=w729) -> ("Array"=w728:dbl[])
        n362 = Array Size(array=w718) -> (size(s)=w716:i32)
        n363 = Array Size(array=w728) -> (size(s)=w712:i32)
        n364 = local read "meas_iter"() -> (w724:i32)
        n365 = local read "binning"() -> (w726:u16)
        n366 = Equal To 0?(x=w716) -> (x = 0?=w717:bool)
        n367 = Select(t=1, s=w717, f=w716) -> (s? t:f=w714:i32)
        n368 = Index Array(array=dbl[] [8.79, 2.2, 0.553, 0.138], index=w726) -> (element=w723:dbl)
        n369 = Multiply(x=w714, y=w712) -> (x*y=w713:i32)
        "measpoints" <- w713
        n370 = Multiply(x=w713, y=w724) -> (x*y=w721:i32)
        "total steps" <- w721
        n371 = Get Date/Time In Seconds() -> (seconds since 1Jan1904=w711:timestamp)
        n372 = Multiply(x=w721, y=w723) -> (x*y=→"disk [MB]":dbl)
        n373 = Multiply(x=w721, y="time/step [s]") -> (x*y=w710:dbl)
        "duration [HH:MM:SS]" <- w710
        n374 = Multiply(x=w712, y=w723) -> (x*y=→"RAM [MB]":dbl)
        n375 = Add(x=w711, y=w710) -> (x+y=→"ETA 2":timestamp)
      }
      event "mirr_go": Value Change {
        n376 = event-data() -> ()  [unwired: 1 in, 1 out]
        n377 = Index Array(array="mirr_dest") -> (element #1=w736:i32, element #2=w735:i32)  [unwired: 2 in]
        n378 = Format Into String(format string="%g_%g", w736, w735) -> (resulting string=w733:string)  [unwired: 2 in, 1 out]
        n379 = Concatenate Strings("abs:" ("string"), w733) -> (w730:string)
        n380 = Enqueue Element(queue=w731, element=w730) -> ()  [unwired: 2 in, 3 out]
      }
      event "scan_manip_setstart": Value Change {
        n381 = event-data() -> ()  [unwired: 1 in, 1 out]
        n382 = local read "pos"() -> (w738:dbl[])
        n383 = local write "scan_manip_start"(w738) -> ()
      }
      event "scan_manip_setstart 2": Value Change {
        n384 = event-data() -> ()  [unwired: 1 in, 1 out]
        n385 = local read "pos"() -> (w739:dbl[])
        n386 = local write "scan_manip_start 2"(w739) -> ()
      }
      event "scan_mirr_setstart": Value Change {
        n387 = event-data() -> ()  [unwired: 1 in, 1 out]
        n388 = local read "mirr_posX"() -> (w742:i32)
        n389 = local read "mirr_posY"() -> (w741:i32)
        n390 = Build Array(w742, w741) -> (w740:i32[])
        n391 = local write "scan_mirr_start"(w740) -> ()
      }
      event "scan_mirr_setstart 2": Value Change {
        n392 = event-data() -> ()  [unwired: 1 in, 1 out]
        n393 = local read "mirr_posX"() -> (w745:i32)
        n394 = local read "mirr_posY"() -> (w744:i32)
        n395 = Build Array(w745, w744) -> (w743:i32[])
        n396 = local write "scan_mirr_start 2"(w743) -> ()
      }
      event "Move Abs": Value Change {
        n397 = event-data() -> ()  [unwired: 1 in, 1 out]
        n398 = Index Array(array="dest") -> (element #1=w755:dbl, element #2=w754:dbl, element #3=w753:dbl, element #4=w752:dbl, element #5=w751:dbl, element #6=w750:dbl)  [unwired: 6 in]
        n399 = Format Into String(format string="%g_%g_%g_%g_%g_%g", w755, w754, w753, w752, w751, w750) -> (resulting string=w748:string)  [unwired: 2 in, 1 out]
        n400 = Concatenate Strings("abs:" ("string"), w748) -> (w747:string)
        n401 = Enqueue Element(queue=w757, element=w747) -> ()  [unwired: 2 in, 3 out]
      }
      event "ManipRel +", "ManipRel -": Value Change {
        n402 = event-data() -> ()  [unwired: 1 in, 2 out]
        n403 = Negate(x="manip_deltas") -> (-x=w761:dbl[])
        n404 = Select(t="manip_deltas", s="ManipRel +", f=w761) -> (s? t:f=w759:dbl[])
        n405 = Index Array(array=w759) -> (element #1=w765:dbl, element #2=w766:dbl, element #3=w767:dbl, element #4=w768:dbl, element #5=w769:dbl, element #6=w770:dbl)  [unwired: 6 in]
        n406 = Format Into String(format string="%g_%g_%g_%g_%g_%g", w765, w766, w767, w768, w769, w770) -> (resulting string=w772:string)  [unwired: 2 in, 1 out]
        n407 = Concatenate Strings("rel:" ("string"), w772, ":wait" ("string")) -> (w763:string)
        n408 = Enqueue Element(queue=w773, element=w763) -> ()  [unwired: 2 in, 3 out]
      }
      event "stop manip": Value Change {
        n409 = event-data() -> ()  [unwired: 1 in, 1 out]
        n410 = Enqueue Element(queue=w775, element="stop") -> ()  [unwired: 2 in, 3 out]
      }
      event "ESP_go": Value Change {
        w777 = ":" ("string")
        n411 = event-data() -> ()  [unwired: 1 in, 1 out]
        n412 = Number To Decimal String(number=0) -> (decimal integer string=w779:string)  [unwired: 1 in]
        n413 = Number To Fractional String(number="ESP_dest") -> (F-format string=w778:string)  [unwired: 3 in]
        n414 = Concatenate Strings("abs:" ("string"), w779, w777, w778, w777) -> (w782:string)
        n415 = Enqueue Element(queue=w783, element=w782) -> ()  [unwired: 2 in, 3 out]
      }
      event "ESP_set_t0": Value Change {
        n416 = event-data() -> ()  [unwired: 1 in, 1 out]
        n417 = Current VI's Path() -> (path=w794:path)
        n418 = Strip Path(path=w794) -> (stripped path=w792:path)  [unwired: 1 out]
        n419 = Strip Path(path=w792) -> (stripped path=w791:path)  [unwired: 1 out]
        n420 = local read "ESP_pos"() -> (w793:dbl)
        "ESP_t0" <- w793
        n421 = Number To Fractional String(number=w793) -> (F-format string=w786:string)  [unwired: 3 in]
        n422 = Build Path(base path=w791, name or relative path="t0.txt") -> (appended path=w788:path)
        n423 = Get Date/Time In Seconds() -> (seconds since 1Jan1904=w790:timestamp)
        n424 = Format Date/Time String(time format string (%c)="%Y.%m.%d %H:%M", seconds (now)=w790) -> (date/time string=w787:string)  [unwired: 1 in]
        n425 = Build Array(w787, w786) -> (w785:string[])
        n426 = call-poly <vilib>:"Write Delimited Spreadsheet.vi"("file path (dialog if empty)"=w788, "1D data"=w785, "append to file? (F)"=TRUE) -> ()  [unwired: 11 in, 2 out]
      }
      event "ESP_opent0file": Value Change {
        n427 = event-data() -> ()  [unwired: 1 in, 6 out]
        n428 = Current VI's Path() -> (path=w798:path)
        n429 = Strip Path(path=w798) -> (stripped path=w797:path)  [unwired: 1 out]
        n430 = Strip Path(path=w797) -> (stripped path=w799:path)  [unwired: 1 out]
        n431 = call <vilib>:"System Exec.vi"("wait until completion? (T)"=FALSE, "working directory"=w799, "command line"="notepad t0.txt") -> ()  [unwired: 5 in, 4 out]
      }
      event "ESP_+", "ESP_-": Value Change {
        n432 = event-data() -> ()  [unwired: 1 in, 6 out]
        n433 = Negate(x="ESP_delta") -> (-x=w808:dbl)
        n434 = Select(t="ESP_delta", s="ESP_+", f=w808) -> (s? t:f=w806:dbl)
        n435 = Number To Decimal String(number=0) -> (decimal integer string=w804:string)  [unwired: 1 in]
        n436 = Number To Fractional String(number=w806) -> (F-format string=w802:string)  [unwired: 3 in]
        n437 = Concatenate Strings("rel:" ("string"), w804, ":" ("string"), w802) -> (w811:string)
        n438 = Enqueue Element(queue=w805, element=w811) -> ()  [unwired: 2 in, 3 out]
      }
      event "ESP_dest": Value Change {
        n439 = event-data() -> ()  [unwired: 1 in, 6 out]
        n440 = local read "ESP_dest"() -> (w815:dbl)
        n441 = local read "ESP_t0"() -> (w814:dbl)
        n442 = call "mm2time.vi"("fs?"=TRUE ("fs[1]/ps[0]"), "Offset (mm)"=w814, "distance (mm)"=w815) -> ("time in fs/ps seconds"=w812:dbl)
        n443 = local write "ESP_dest_t"(w812) -> ()
      }
      event "ESP_dest_t": Value Change {
        n444 = event-data() -> ()  [unwired: 1 in, 1 out]
        n445 = local read "ESP_t0"() -> (w818:dbl)
        n446 = call "time2mm.vi"("fs[1]/ps[0]"=TRUE, "Offset (mm)"=w818, "time"="ESP_dest_t") -> ("position (mm)"=w816:dbl)
        n447 = local write "ESP_dest"(w816) -> ()
      }
      event "load waypoints 1": Value Change {
        n448 = event-data() -> ()  [unwired: 1 in, 6 out]
        n449 = call-poly <vilib>:"Read Delimited Spreadsheet.vi"() -> ("all rows"=w821:string[][], "error out"=w820:errorcluster)  [unwired: 10 in, 4 out]
        n450 = case shown="No Error" w820 {
          tunnel: w821 -> [w822 _]
          frame No Error {
            n451 = local write "waypointsD1"(w822) -> ()
          }
          frame Error {
          }
        }
      }
      event "load waypoints 2": Value Change {
        n452 = event-data() -> ()  [unwired: 1 in, 6 out]
        n453 = call-poly <vilib>:"Read Delimited Spreadsheet.vi"() -> ("all rows"=w824:string[][], "error out"=w823:errorcluster)  [unwired: 10 in, 4 out]
        n454 = case shown="No Error" w823 {
          tunnel: w824 -> [w825 _]
          frame No Error {
            n455 = local write "waypointsD2"(w825) -> ()
          }
          frame Error {
          }
        }
      }
      event "clear waypoints 1": Value Change {
        n456 = event-data() -> ()  [unwired: 1 in, 6 out]
        n457 = local write "waypointsD1"(string[][] []) -> ()
      }
      event "clear waypoints 2": Value Change {
        n458 = event-data() -> ()  [unwired: 1 in, 6 out]
        n459 = local write "waypointsD2"(string[][] []) -> ()
      }
      event "mainimg": Cursor Release {
        n460 = event-data() -> ()  [unwired: 1 in, 1 out]
        n461 = Enqueue Element(queue=w829, element="refresh") -> ()  [unwired: 2 in, 3 out]
      }
      event "mirr_init", "mirr_release": Value Change {
        n462 = event-data() -> ()  [unwired: 1 in, 6 out]
        n463 = Flush Queue(queue=w831) -> (queue out=w832:refnum<queue>)  [unwired: 1 in, 2 out]
        n464 = Select(t="init" ("name (unnamed)"), s="mirr_init", f="release" ("name (unnamed)")) -> (s? t:f=w833:string)
        n465 = Enqueue Element(queue=w832, element=w833) -> ()  [unwired: 2 in, 3 out]
      }
      event "mirr_X-", "mirr_X+", "mirr_Y+", "mirr_Y-": Value Change {
        n466 = event-data() -> ()  [unwired: 1 in, 1 out]
        n467 = local read "mirr_X#"() -> (w843:u8)
        n468 = local read "mirr_Y#"() -> (w842:u8)
        n469 = Or(x="mirr_X+", y="mirr_X-") -> (x .or. y?=w844:bool)
        n470 = Or(x="mirr_X-", y="mirr_Y-") -> (x .or. y?=w850:bool)
        n471 = Negate(x="mirr_rel") -> (-x=w849:i32)
        n472 = Select(t=w843, s=w844, f=w842) -> (s? t:f=w841:u8)
        n473 = Select(t=w849, s=w850, f="mirr_rel") -> (s? t:f=w838:i32)
        n474 = Number To Decimal String(number=w841) -> (decimal integer string=w840:string)  [unwired: 1 in]
        n475 = Number To Decimal String(number=w838) -> (decimal integer string=w837:string)  [unwired: 1 in]
        n476 = Concatenate Strings("rel:" ("string"), w840, ":" ("string"), w837) -> (w836:string)
        n477 = Enqueue Element(queue=w852, element=w836) -> ()  [unwired: 2 in, 3 out]
      }
    }
  }
  n478 = while {
    tunnel: w15 -> [w861]
    shift-right: [w858] -> _
    shift-left: _ -> [w859]
    tunnel: w8 -> [w857]
    shift-right: [w856] -> _
    shift-left: _ -> [w855]
    shift-right: [w853] -> _
    shift-left: _ -> [w854]
    stop <- w860 stop-if-true
    # "mirr"
    n479 = Preview Queue Element(queue=w861, timeout in ms (-1)=w859) -> (queue out=w864:refnum<queue>, element=w865:string)  [unwired: 1 in, 2 out]
    n480 = Match Pattern(string=w865, regular expression=":") -> (before substring=w863:string, after substring=w862:string)  [unwired: 1 in, 2 out]
    n481 = case shown="\"close\"" w863 {
      tunnel: w864 -> [w900 w910 w925 w929 w932 w937 _]
      tunnel: w862 -> [w894 w911 _ _ _ _ _]
      tunnel: [_ _ _ TRUE _ _ _] -> w860
      tunnel: [_ _ _ _ -1 _ _] -> w858
      tunnel: w857 -> [w867 _ _ _ _ _ _]
      tunnel: [w886 w907 refnum<visa-resource-name> refnum ("VISA resource name out") w927 w931 w936 w942] -> w856
      tunnel: w855 -> [w899 w909 w924 w927 w931 _ w946]
      tunnel: [w871 w906 w923 w926 w930 w935 w941] -> w853
      tunnel: w854 -> [w898 w908 _ w926 w930 _ w945]
      frame "abs" {
        w882 = u8 20 items=["Echo"=55, "Home"=1, "Move Absolute"=20, "Move Relative"=21, "Move at Constant Speed"=22, "Renumber"=2, "Restore Settings"=36, "Stop"=23] ("Command")
        w897 = u8 20 items=["Echo"=55, "Home"=1, "Move Absolute"=20, "Move Relative"=21, "Move at Constant Speed"=22, "Renumber"=2, "Restore Settings"=36, "Stop"=23] ("Command")
        n482 = Dequeue Element(queue=w900) -> ()  [unwired: 2 in, 4 out]
        n483 = Match Pattern(string=w894, regular expression=":") -> (before substring=w884:string, after substring=w870:string)  [unwired: 1 in, 2 out]
        n484 = Equal?(x=w870, y="wait") -> (x = y?=w868:bool)
        n485 = Scan From String(format string="%g_%g", input string=w884) -> (output 1=w879:dbl, output 2=w878:dbl)  [unwired: 4 in, 3 out]
        n486 = local read "mirr_X#"() -> (w881:u8)
        n487 = Bundle("mirr_X#"=w881, "Command"=w897, w879, "Response Count"=1) -> (w893:T6)  [unwired: 1 in]
        n488 = local read "mirr_Y#"() -> (w880:u8)
        n489 = call "Request Command.vi"("error in (no error)"=w898, "Request"=w893, "VISA resource name"=w899) -> ("error out"=w875:errorcluster, "VISA resource name out"=w876:refnum<visa-resource-name>)  [unwired: 5 in, 2 out]
        n490 = Bundle("mirr_Y#"=w880, "Command"=w882, w878, "Response Count"=1) -> (w877:T7)  [unwired: 1 in]
        n491 = call "Request Command.vi"("error in (no error)"=w875, "Request"=w877, "VISA resource name"=w876) -> ("error out"=w873:errorcluster, "VISA resource name out"=w874:refnum<visa-resource-name>)  [unwired: 5 in, 2 out]
        n492 = local read "mirr_X#"() -> (w891:u8)
        n493 = call "zaber_readpos.vi"("error in (no error)"=w873, "axis"=w891, "VISA in"=w874) -> ("error out"=w887:errorcluster, "position"=w892:i32, "VISA out"=w888:refnum<visa-resource-name>)  [unwired: 6 in]
        n494 = local read "mirr_Y#"() -> (w889:u8)
        n495 = local write "mirr_posX"(w892) -> ()
        n496 = call "zaber_readpos.vi"("error in (no error)"=w887, "axis"=w889, "VISA in"=w888) -> ("error out"=w872:errorcluster, "position"=w890:i32, "VISA out"=w886:refnum<visa-resource-name>)  [unwired: 6 in]
        n497 = local write "mirr_posY"(w890) -> ()
        n498 = case shown="True" w868 {
          tunnel: w872 -> [w901 w905]
          tunnel: [w901 w904] -> w871
          tunnel: w867 -> [_ w903]
          frame False {
          }
          frame True {
            n499 = Send Notification(notification=TRUE, notifier=w903, error in (no error)=w905) -> (error out=w904:errorcluster)  [unwired: 1 out]
          }
        }
      }
      frame "rel" {
        w914 = u8 21 items=["Echo"=55, "Home"=1, "Move Absolute"=20, "Move Relative"=21, "Move at Constant Speed"=22, "Renumber"=2, "Restore Settings"=36, "Stop"=23] ("Command")
        n500 = Dequeue Element(queue=w910) -> ()  [unwired: 2 in, 4 out]
        n501 = Match Pattern(string=w911, regular expression=":") -> (before substring=w916:string, after substring=w915:string)  [unwired: 1 in, 2 out]
        n502 = Decimal String To Number(string=w916) -> (number=w918:i32)  [unwired: 2 in, 1 out]
        n503 = Decimal String To Number(string=w915) -> (number=w919:i32)  [unwired: 2 in, 1 out]
        n504 = Bundle(w918, "Command"=w914, w919, "Response Count"=1) -> (w912:T8)  [unwired: 1 in]
        n505 = call "Request Command.vi"("error in (no error)"=w908, "Request"=w912, "VISA resource name"=w909) -> ("error out"=w906:errorcluster, "VISA resource name out"=w907:refnum<visa-resource-name>)  [unwired: 5 in, 2 out]
      }
      frame "release" {
        n506 = Dequeue Element(queue=w925) -> (queue out=w921:refnum<queue>)  [unwired: 2 in, 3 out]
        n507 = Enqueue Element(queue=w921, element="suspend") -> ()  [unwired: 2 in, 3 out]
        n508 = call "Close.vi"("VISA resource name"=w924) -> ("error out"=w923:errorcluster)  [unwired: 9 in, 1 out]
      }
      frame "close" {
        n509 = Release Queue(queue=w929) -> ()  [unwired: 2 in, 3 out]
      }
      frame "suspend" {
        n510 = Dequeue Element(queue=w932) -> ()  [unwired: 2 in, 4 out]
      }
      frame "init" {
        n511 = Dequeue Element(queue=w937) -> ()  [unwired: 2 in, 4 out]
        n512 = call "Initialize.vi"("VISA resource name"="mirr_VISA") -> ("error out"=w935:errorcluster, "VISA resource name out"=w936:refnum<visa-resource-name>)  [unwired: 8 in, 1 out]
      }
      frame "idle", Default {
        n513 = local read "mirr_X#"() -> (w947:u8)
        n514 = call "zaber_readpos.vi"("error in (no error)"=w945, "axis"=w947, "VISA in"=w946) -> ("error out"=w943:errorcluster, "position"=→"mirr_posX":i32, "VISA out"=w944:refnum<visa-resource-name>)  [unwired: 6 in]
        n515 = local read "mirr_Y#"() -> (w940:u8)
        n516 = call "zaber_readpos.vi"("error in (no error)"=w943, "axis"=w940, "VISA in"=w944) -> ("error out"=w941:errorcluster, "position"=→"mirr_posY":i32, "VISA out"=w942:refnum<visa-resource-name>)  [unwired: 6 in]
      }
    }
    "mirr_Error" <- w853
  }
  n517 = while {
    tunnel: w24 -> [w957]
    shift-right: [w955] -> _
    shift-left: _ -> [w953]
    shift-right: [w954] -> _
    shift-left: _ -> [w952]
    shift-right: [w950] -> _
    shift-left: 0 -> [w951]
    tunnel: w8 -> [w949]
    stop <- w956 stop-if-true
    # "ESP"
    n518 = Preview Queue Element(queue=w957, timeout in ms (-1)=w951) -> (queue out=w960:refnum<queue>, element=w961:string)  [unwired: 1 in, 2 out]
    n519 = Match Pattern(string=w961, regular expression=":") -> (before substring=w959:string, after substring=w958:string)  [unwired: 1 in, 2 out]
    n520 = case shown="\"idle\", Default" w959 {
      tunnel: w960 -> [_ w983 w1003 w1043 w1046 w1053 w1058]
      tunnel: w958 -> [_ w987 w1009 _ _ _ _]
      tunnel: [_ _ _ _ _ TRUE _] -> w956
      tunnel: [w966 w989 w1004 w1041 refnum<visa-resource-name> refnum ("VISA resource name out") w1050 w1057] -> w955
      tunnel: [w967 w990 w1002 w1040 w1048 w1051 w1056] -> w954
      tunnel: w953 -> [w976 w992 w1007 w1041 w1049 w1050 _]
      tunnel: w952 -> [w975 w991 w1008 w1040 _ w1051 _]
      tunnel: [_ _ _ -1 _ _ _] -> w950
      tunnel: w949 -> [_ _ w996 _ _ _ _]
      tunnel: "ESP patch" -> [w973 w982 w995 _ _ _ _]
      frame "idle", Default {
        n521 = Index Array(array=w973) -> (element #1=w972:i32, element #2=w969:i32)  [unwired: 3 in, 1 out]
        n522 = local read "ESP_t0"() -> (w979:dbl)
        n523 = call "Read Actual Position.vi"("error in (no error)"=w975, "Axis (1)"=w972, "VISA resource name"=w976) -> ("error out"=w970:errorcluster, "Position (units)"=w974:dbl, "VISA resource name out"=w971:refnum<visa-resource-name>)  [unwired: 2 in]
        "ESP_pos" <- w974
        n524 = call "mm2time.vi"("fs?"=TRUE, "Offset (mm)"=w979, "distance (mm)"=w974) -> ("time in fs/ps seconds"=→"ESP_delay":dbl)
        n525 = call "Read Actual Position.vi"("error in (no error)"=w970, "Axis (1)"=w969, "VISA resource name"=w971) -> ("error out"=w968:errorcluster, "Position (units)"=→"waveplate position":dbl, "VISA resource name out"=w965:refnum<visa-resource-name>)  [unwired: 2 in]
        n526 = call "Read Actual Position.vi"("error in (no error)"=w968, "VISA resource name"=w965) -> ("error out"=w967:errorcluster, "Position (units)"=→"stage2 position":dbl, "VISA resource name out"=w966:refnum<visa-resource-name>)  [unwired: 3 in]
      }
      frame "rel" {
        n527 = Dequeue Element(queue=w983) -> ()  [unwired: 2 in, 4 out]
        n528 = Match Pattern(string=w987, regular expression=":") -> (before substring=w986:string, after substring=w985:string)  [unwired: 1 in, 2 out]
        n529 = Decimal String To Number(string=w986) -> (number=w981:i32)  [unwired: 2 in, 1 out]
        n530 = Fract/Exp String To Number(string=w985) -> (number=w984:dbl)  [unwired: 3 in, 1 out]
        n531 = Index Array(array=w982, index=w981) -> (element=w980:i32)
        n532 = call "Move Relative.vi"("error in (no error)"=w991, "Position (0 units)"=w984, "Axis (1)"=w980, "VISA resource name"=w992) -> ("error out"=w990:errorcluster, "VISA resource name out"=w989:refnum<visa-resource-name>)  [unwired: 2 in]
      }
      frame "abs" {
        n533 = Dequeue Element(queue=w1003) -> ()  [unwired: 2 in, 4 out]
        n534 = Match Pattern(string=w1009, regular expression=":") -> (before substring=w1010:string, after substring=w1000:string)  [unwired: 1 in, 2 out]
        n535 = Match Pattern(string=w1000, regular expression=":") -> (before substring=w999:string, after substring=w998:string)  [unwired: 1 in, 2 out]
        n536 = Decimal String To Number(string=w1010) -> (number=w994:i32)  [unwired: 2 in, 1 out]
        n537 = Fract/Exp String To Number(string=w999) -> (number=w997:dbl)  [unwired: 3 in, 1 out]
        n538 = Index Array(array=w995, index=w994) -> (element=w993:i32)
        n539 = call "Move Absolute.vi"("error in (no error)"=w1008, "Position (0 units)"=w997, "Axis (1)"=w993, "VISA resource name"=w1007) -> ("error out"=w1005:errorcluster, "VISA resource name out"=w1006:refnum<visa-resource-name>)  [unwired: 2 in]
        n540 = case shown="\"wait\"" w998 {
          tunnel: w993 -> [_ w1014]
          tunnel: w1006 -> [w1013 w1030]
          tunnel: w1005 -> [w1012 w1029]
          tunnel: [w1013 w1019] -> w1004
          tunnel: [w1012 w1026] -> w1002
          tunnel: w996 -> [_ w1025]
          frame "", Default {
          }
          frame "wait" {
            n541 = while {
              tunnel: w1014 -> [w1039]
              shift-right: [w1036] -> w1028
              shift-left: w1030 -> [w1038]
              shift-right: [w1035] -> w1027
              shift-left: w1029 -> [w1037]
              stop <- w1034 stop-if-true
              n542 = call "Get Axis Motion Status.vi"("error in (no error)"=w1037, "Axis (1)"=w1039, "VISA resource name"=w1038) -> ("error out"=w1035:errorcluster, "Motion Done"=w1034:bool, "VISA resource name out"=w1036:refnum<visa-resource-name>)  [unwired: 2 in]
            }
            n543 = flat-sequence {
              tunnel: w1028 -> [w1033]
              tunnel: w1027 -> [w1032]
              tunnel: [w1033] -> w1021
              tunnel: [w1032] -> w1020
              frame #0 {
                n544 = Wait (ms)(milliseconds to wait=u32 1000) -> ()  [unwired: 1 out]
              }
            }
            n545 = local read "ESP_t0"() -> (w1023:dbl)
            n546 = call "Read Actual Position.vi"("error in (no error)"=w1020, "Axis (1)"=w1014, "VISA resource name"=w1021) -> ("error out"=w1015:errorcluster, "Position (units)"=w1017:dbl, "VISA resource name out"=w1019:refnum<visa-resource-name>)  [unwired: 2 in]
            n547 = call "mm2time.vi"("fs?"=TRUE, "Offset (mm)"=w1023, "distance (mm)"=w1017) -> ("time in fs/ps seconds"=w1018:dbl)
            n548 = call <vilib>:"Clear Errors.vi"("error in (no error)"=w1015) -> ("error out"=w1016:errorcluster)  [unwired: 5 in, 1 out]
            n549 = local write "ESP_pos"(w1017) -> ()
            n550 = local write "ESP_delay"(w1018) -> ()
            n551 = Send Notification(notification=TRUE, notifier=w1025, error in (no error)=w1016) -> (error out=w1026:errorcluster)  [unwired: 1 out]
          }
        }
      }
      frame "suspend" {
        n552 = Dequeue Element(queue=w1043) -> ()  [unwired: 2 in, 4 out]
      }
      frame "release" {
        n553 = Dequeue Element(queue=w1046) -> (queue out=w1044:refnum<queue>)  [unwired: 2 in, 3 out]
        n554 = call "Close.vi"("VISA resource name"=w1049) -> ("error out"=w1048:errorcluster)  [unwired: 10 in]
        n555 = Enqueue Element(queue=w1044, element="suspend") -> ()  [unwired: 2 in, 3 out]
      }
      frame "close" {
        n556 = Release Queue(queue=w1053) -> ()  [unwired: 2 in, 3 out]
      }
      frame "init" {
        n557 = Dequeue Element(queue=w1058) -> ()  [unwired: 2 in, 4 out]
        n558 = flat-sequence {
          tunnel: [w1061] -> w1055
          tunnel: [w1060] -> w1054
          tunnel: [w1065] -> w1056
          tunnel: [w1066] -> w1057
          tunnel: w1055 -> [w1066]
          tunnel: w1054 -> [w1065]
          frame #0 {
            n559 = local write "ESP_con?"(FALSE ("ESP_con?")) -> ()
          }
          frame #1 {
            n560 = call "Initialize.vi"("VISA resource name"="ESP301 VISA", "Serial Link (RS232)"=enum16{"RS232", "USB"}."RS232") -> ("VISA resource name out"=w1061:refnum<visa-resource-name>, "error out"=w1060:errorcluster)  [unwired: 7 in]
          }
          frame #2 {
            n561 = local write "ESP_con?"(TRUE ("ESP_con?")) -> ()
          }
        }
      }
    }
    "error out" <- w954
  }
  n562 = while {
    tunnel: w23 -> [w1075]
    shift-right: [w1073] -> _
    shift-left: _ -> [w1071]
    shift-right: [w1072] -> _
    shift-left: _ -> [w1070]
    shift-right: [w1068] -> _
    shift-left: 0 -> [w1069]
    tunnel: w8 -> [w1067]
    stop <- w1074 stop-if-true
    # "manip"
    n563 = Preview Queue Element(queue=w1075, timeout in ms (-1)=w1069) -> (queue out=w1078:refnum<queue>, element=w1079:string)  [unwired: 1 in, 2 out]
    n564 = Match Pattern(string=w1079, regular expression=":") -> (before substring=w1077:string, after substring=w1076:string)  [unwired: 1 in, 2 out]
    n565 = case shown="\"init\"" w1077 {
      tunnel: w1078 -> [_ w1091 w1118 w1165 w1203 w1209 w1218 w1223]
      tunnel: w1076 -> [_ _ w1105 w1164 _ _ _ _]
      tunnel: [_ _ _ _ _ _ TRUE _] -> w1074
      tunnel: [w1085 w1093 w1097 w1162 w1205 refnum<k5> refnum ("gateway_connection out") w1216 w1222] -> w1073
      tunnel: [w1084 w1092 w1099 w1161 w1204 w1211 w1215 w1221] -> w1072
      tunnel: w1071 -> [w1087 w1095 w1121 w1155 w1205 w1213 w1216 _]
      tunnel: w1070 -> [w1086 w1094 w1120 w1156 w1204 _ w1215 _]
      tunnel: [_ _ _ _ -1 _ _ _] -> w1068
      tunnel: w1067 -> [_ _ w1096 w1158 _ _ _ _]
      frame "idle", Default {
        n566 = call "sp_manip_get_axis_status.vi"("error in"=w1086, "gateway_connection"=w1087) -> ("error out"=w1084:errorcluster, "axis_out"=w1083:T9, "gateway_connection out"=w1085:refnum<k5>)  [unwired: 5 in, 2 out]
        n567 = for {
          tunnel: w1083 -> [w1090] mode=indexing
          tunnel: [w1089] -> w1082 mode=indexing
          tunnel: [w1088] -> w1081 mode=indexing
          n568 = Unbundle By Name(w1090) -> ("Axis_Position"=w1089:dbl, "moving"=w1088:bool)
        }
        "moving?" <- w1081
        n569 = local write "pos"(w1082) -> ()
      }
      frame "stop" {
        n570 = Dequeue Element(queue=w1091) -> ()  [unwired: 2 in, 4 out]
        n571 = call "sp_manip_abort.vi"("error in"=w1094, "gateway_connection"=w1095) -> ("error out"=w1092:errorcluster, "gateway_connection out"=w1093:refnum<k5>)  [unwired: 6 in, 2 out]
      }
      frame "rel" {
        n572 = Dequeue Element(queue=w1118) -> ()  [unwired: 2 in, 4 out]
        n573 = Match Pattern(string=w1105, regular expression=":") -> (before substring=w1104:string, after substring=w1103:string)  [unwired: 1 in, 2 out]
        n574 = Equal?(x=w1103, y="wait") -> (x = y?=w1101:bool)
        n575 = call "sp_manip_get_axis_status.vi"("error in"=w1120, "gateway_connection"=w1121) -> ("error out"=w1123:errorcluster, "axis_out"=w1110:T9, "gateway_connection out"=w1122:refnum<k5>)  [unwired: 5 in, 2 out]
        n576 = Scan From String(format string="%g_%g_%g_%g_%g_%g", input string=w1104) -> (output 1=w1117:dbl, output 2=w1116:dbl, output 3=w1115:dbl, output 4=w1114:dbl, output 5=w1113:dbl, output 6=w1112:dbl)  [unwired: 8 in, 3 out]
        n577 = for {
          tunnel: w1110 -> [w1150] mode=indexing
          tunnel: [w1149] -> w1108 mode=indexing
          tunnel: [w1148] -> w1109 mode=indexing
          n578 = Unbundle By Name(w1150) -> ("Axis_Name"=w1149:string, "Axis_Position"=w1148:dbl)
        }
        n579 = Build Array(w1117, w1116, w1115, w1114, w1113, w1112) -> (w1111:dbl[])
        n580 = Add(x=w1109, y=w1111) -> (x+y=w1107:dbl[])
        n581 = call "sp_manip_start_move.vi"("error in"=w1123, "target positions"=w1107, "axis names"=w1108, "gateway_connection"=w1122) -> ("error out"=w1100:errorcluster, "gateway_connection out"=w1098:refnum<k5>)  [unwired: 4 in, 2 out]
        n582 = case shown="True" w1101 {
          tunnel: w1100 -> [w1124 w1135]
          tunnel: [w1124 w1134] -> w1099
          tunnel: w1098 -> [w1125 w1136]
          tunnel: [w1125 w1128] -> w1097
          tunnel: w1096 -> [_ w1133]
          frame False {
          }
          frame True {
            n583 = while {
              tunnel: w1136 -> [w1142]
              tunnel: w1135 -> [w1141]
              tunnel: [w1140] -> w1129
              tunnel: [w1139] -> w1127
              stop <- w1143 continue-if-true
              n584 = call "sp_manip_get_axis_status.vi"("error in"=w1141, "gateway_connection"=w1142) -> ("error out"=w1139:errorcluster, "axis_out"=w1145:T9, "gateway_connection out"=w1140:refnum<k5>)  [unwired: 5 in, 2 out]
              n585 = for {
                tunnel: w1145 -> [w1147] mode=indexing
                tunnel: [w1146] -> w1144 mode=indexing
                n586 = Unbundle By Name(w1147) -> ("moving"=w1146:bool)
              }
              n587 = Or Array Elements(Boolean array=w1144) -> (logical OR=w1143:bool)
            }
            n588 = call "sp_manip_get_axis_status.vi"("error in"=w1127, "gateway_connection"=w1129) -> ("error out"=w1126:errorcluster, "axis_out"=w1131:T9, "gateway_connection out"=w1128:refnum<k5>)  [unwired: 5 in, 2 out]
            n589 = for {
              tunnel: w1131 -> [w1138] mode=indexing
              tunnel: [w1137] -> w1130 mode=indexing
              n590 = Unbundle By Name(w1138) -> ("Axis_Position"=w1137:dbl)
            }
            n591 = Send Notification(notification=TRUE, notifier=w1133, error in (no error)=w1126) -> (error out=w1134:errorcluster)  [unwired: 1 out]
            n592 = local write "dest"(w1130) -> ()
          }
        }
      }
      frame "abs" {
        n593 = Dequeue Element(queue=w1165) -> ()  [unwired: 2 in, 4 out]
        n594 = call "sp_manip_get_axis_status.vi"("error in"=w1156, "gateway_connection"=w1155) -> ("error out"=w1151:errorcluster, "axis_out"=w1154:T9, "gateway_connection out"=w1152:refnum<k5>)  [unwired: 5 in, 2 out]
        n595 = Match Pattern(string=w1164, regular expression=":") -> (before substring=w1168:string, after substring=w1167:string)  [unwired: 1 in, 2 out]
        n596 = Equal?(x=w1167, y="wait") -> (x = y?=w1157:bool)
        n597 = for {
          tunnel: w1154 -> [w1178] mode=indexing
          tunnel: [w1177] -> w1153 mode=indexing
          n598 = Unbundle By Name(w1178) -> ("Axis_Name"=w1177:string)
        }
        n599 = Scan From String(format string="%g_%g_%g_%g_%g_%g", input string=w1168) -> (output 1=w1174:dbl, output 2=w1173:dbl, output 3=w1172:dbl, output 4=w1171:dbl, output 5=w1170:dbl, output 6=w1169:dbl)  [unwired: 8 in, 3 out]
        n600 = Build Array(w1174, w1173, w1172, w1171, w1170, w1169) -> (w1176:dbl[])
        n601 = call "sp_manip_start_move.vi"("error in"=w1151, "target positions"=w1176, "axis names"=w1153, "gateway_connection"=w1152) -> ("error out"=w1160:errorcluster, "gateway_connection out"=w1159:refnum<k5>)  [unwired: 4 in, 2 out]
        n602 = case shown="True" w1157 {
          tunnel: w1160 -> [w1179 w1190]
          tunnel: [w1179 w1189] -> w1161
          tunnel: w1159 -> [w1180 w1191]
          tunnel: [w1180 w1182] -> w1162
          tunnel: w1158 -> [_ w1188]
          frame False {
          }
          frame True {
            n603 = while {
              tunnel: w1191 -> [w1197]
              tunnel: w1190 -> [w1196]
              tunnel: [w1195] -> w1184
              tunnel: [w1194] -> w1183
              stop <- w1198 continue-if-true
              n604 = call "sp_manip_get_axis_status.vi"("error in"=w1196, "gateway_connection"=w1197) -> ("error out"=w1194:errorcluster, "axis_out"=w1200:T9, "gateway_connection out"=w1195:refnum<k5>)  [unwired: 5 in, 2 out]
              n605 = for {
                tunnel: w1200 -> [w1202] mode=indexing
                tunnel: [w1201] -> w1199 mode=indexing
                n606 = Unbundle By Name(w1202) -> ("moving"=w1201:bool)
              }
              n607 = Or Array Elements(Boolean array=w1199) -> (logical OR=w1198:bool)
            }
            n608 = call "sp_manip_get_axis_status.vi"("error in"=w1183, "gateway_connection"=w1184) -> ("error out"=w1181:errorcluster, "axis_out"=w1186:T9, "gateway_connection out"=w1182:refnum<k5>)  [unwired: 5 in, 2 out]
            n609 = for {
              tunnel: w1186 -> [w1193] mode=indexing
              tunnel: [w1192] -> w1185 mode=indexing
              n610 = Unbundle By Name(w1193) -> ("Axis_Position"=w1192:dbl)
            }
            n611 = local write "pos"(w1185) -> ()
            n612 = Send Notification(notification=TRUE, notifier=w1188, error in (no error)=w1181) -> (error out=w1189:errorcluster)  [unwired: 1 out]
          }
        }
      }
      frame "suspend" {
        n613 = Dequeue Element(queue=w1203) -> ()  [unwired: 2 in, 4 out]
      }
      frame "release" {
        n614 = Dequeue Element(queue=w1209) -> (queue out=w1207:refnum<queue>)  [unwired: 2 in, 3 out]
        n615 = call "sp_manip_disconnect.vi"("gateway_connection"=w1213) -> ("error out"=w1212:errorcluster, "gateway_connection_out"=w1214:refnum<k5>)  [unwired: 7 in, 2 out]
        n616 = call "tcp_gateway_close_connection.vi"("error in"=w1212, "server_connection"=w1214) -> ("error out"=w1211:errorcluster)  [unwired: 5 in]
        n617 = Enqueue Element(queue=w1207, element="suspend") -> ()  [unwired: 2 in, 3 out]
      }
      frame "close" {
        n618 = Release Queue(queue=w1218) -> ()  [unwired: 2 in, 3 out]
      }
      frame "init" {
        n619 = Dequeue Element(queue=w1223) -> ()  [unwired: 2 in, 4 out]
        n620 = flat-sequence {
          tunnel: [w1226] -> w1220
          tunnel: [w1225] -> w1219
          tunnel: [w1236] -> w1221
          tunnel: [w1237] -> w1222
          tunnel: w1220 -> [w1237]
          tunnel: w1219 -> [w1236]
          frame #0 {
            n621 = local write "manip_con?"(FALSE ("manip_con?")) -> ()
          }
          frame #1 {
            n622 = call "tcp_gateway_open_connection.vi"() -> ("gateway_connection"=w1229:refnum<k5>, "error out"=w1228:errorcluster)  [unwired: 5 in, 3 out]
            n623 = call "sp_manip_connect.vi"("error in"=w1228, "gateway_connection"=w1229) -> ("error out"=w1225:errorcluster, "axis_out"=w1227:T9, "gateway_connection out"=w1226:refnum<k5>)  [unwired: 5 in, 2 out]
            n624 = for {
              tunnel: w1227 -> [w1234] mode=indexing
              tunnel: [w1233] -> w1230 mode=indexing
              tunnel: [w1232] -> w1231 mode=indexing
              n625 = Unbundle By Name(w1234) -> ("Axis_Name"=w1233:string, "Axis_Position"=w1232:dbl)
            }
            "axis" <- w1230
            "pos" <- w1231
            n626 = local write "dest"(w1231) -> ()
          }
          frame #2 {
            n627 = local write "manip_con?"(TRUE ("manip_con?")) -> ()
          }
        }
      }
    }
    "error out 2" <- w1072
  }
  n628 = while {
    tunnel: w22 -> [w1251]
    shift-right: [w1240] -> _
    shift-left: 0 -> [w1249]
    shift-right: [w1248] -> _
    shift-left: _ -> [w1247]
    shift-right: [w1246] -> _
    shift-left: _ -> [w1245]
    shift-right: [w1244] -> _
    shift-left: u32 0 ("pHandle") -> [w1243]
    tunnel: w20 -> [w1242]
    tunnel: w8 -> [w1241]
    tunnel: w1 -> [w1239]
    stop <- w1250 stop-if-true
    # "phoib"
    n629 = Preview Queue Element(queue=w1251, timeout in ms (-1)=w1249) -> (queue out=w1254:refnum<queue>, element=w1255:string)  [unwired: 1 in, 2 out]
    n630 = Wait Until Next ms Multiple(millisecond multiple=u32 1000) -> ()  [unwired: 1 out]
    n631 = Match Pattern(string=w1255, regular expression=":") -> (before substring=w1253:string, after substring=w1252:string)  [unwired: 1 in, 2 out]
    n632 = case shown="\"standby\"" w1253 {
      tunnel: w1254 -> [_ w1319 w1374 w1391 w1409 w1423 w1428 w1433]
      tunnel: w1252 -> [_ _ w1370 _ _ _ _ _]
      tunnel: [_ _ _ _ _ TRUE _ _] -> w1250
      tunnel: [w1274 w1321 w1339 w1394 w1407 w1421 w1427 w1430] -> w1248
      tunnel: w1247 -> [w1284 w1310 w1360 w1396 w1408 w1421 w1427 _]
      tunnel: [w1273 w1320 w1355 w1393 w1406 w1419 w1425 w1429] -> w1246
      tunnel: w1245 -> [w1282 w1309 _ w1395 _ w1419 w1425 _]
      tunnel: [w1271 w1307 w1338 w1392 w1405 w1420 w1426 w1432] -> w1244
      tunnel: w1243 -> [w1271 w1307 w1358 w1392 w1404 w1420 w1426 _]
      tunnel: w1242 -> [w1272 w1300 w1336 _ _ _ _ _]
      tunnel: w1241 -> [_ _ w1354 _ _ _ _ _]
      tunnel: [_ _ _ _ _ _ -1 _] -> w1240
      tunnel: w1239 -> [w1259 _ _ _ _ _ _ _]
      frame "idle", Default {
        n633 = call "SL2_AD_DLL_Phoibos_GetDeviceState.vi"("dll_path"=w1284, "pHandle_in"=w1271, "dev_type"=DEF_dev_type."devA (analyzer)", "error in"=w1282) -> ("path out"=w1270:path, "state"=w1262:T3, "error out"=w1269:errorcluster)  [unwired: 2 in]
        "state" <- w1262
        n634 = Format Into String(w1262) -> (resulting string=w1263:string)  [unwired: 3 in, 1 out]
        n635 = Format Date/Time String(time format string (%c)="%H:%M:%S") -> (date/time string=w1257:string)  [unwired: 2 in]
        n636 = Concatenate Strings(w1257, "\t", w1263, "\r\n") -> (w1260:string)
        n637 = Write to Text File(file (use dialog)=w1259, text=w1260) -> ()  [unwired: 2 in, 3 out]
        n638 = for {
          tunnel: w1271 -> [w1291]
          tunnel: w1272 -> [w1289] mode=indexing
          tunnel: [w1288] -> w1281 mode=indexing
          tunnel: [w1287] -> w1274
          shift-right: [w1286] -> w1273
          shift-left: w1269 -> [w1290]
          tunnel: w1270 -> [w1285]
          n639 = call "SL2_AD_DLL_Phoibos_GetVoltage.vi"("error in"=w1290, "voltage_name"=w1289, "pHandle"=w1291, "dll path in"=w1285) -> ("error out"=w1286:errorcluster, "value"=w1288:dbl, "dll path out"=w1287:path)  [unwired: 3 in]
        }
        n640 = Index Array(array=w1281) -> (element #1=→"phoib_I_1":dbl, element #2=→"phoib_I_2":dbl, element #3=→"phoib_I_3":dbl, element #4=→"phoib_I_4":dbl, element #5=→"phoib_I_5":dbl, element #6=→"phoib_I_6":dbl, element #7=→"phoib_I_7":dbl, element #8=→"phoib_I_8":dbl, element #9=→"phoib_I_9":dbl, element #10=→"phoib_I_10":dbl)  [unwired: 10 in]
      }
      frame "set" {
        n641 = Dequeue Element(queue=w1319) -> ()  [unwired: 2 in, 4 out]
        n642 = Add(x=u32[] [251749632, 251749633, 251749634, 251749635, 251749636, 251749637, 251749638, 251749639, 251749640, 251749641, 251749642, 251749643, 251749644, 251749645, 251749646, 251749647, 251749648, 251749649, 251749650, 251749651, 251749652, 251749653, 251749654, 251749655, 251749656, 251749657, 251749658, 251749659, 251749660, 251749661, 251749662, 251749663, 251749664, 251749665, 251749666, 251749667, 251749668, 251749669, 251749670, 251749671, 251749672, 251749673, 251749674, 251749675, 251749676, 251749677, 251749678, 251749679, 251749680, 251749681, 251749682, 251749683, 251749684, 251749685, 251749686, 251749687, 251749688, 251749689, 251749690, 251749691, 251749692, 251749693, 251749694, 251749695, 251749696] ("modeIDs"), y=9984) -> (x+y=w1293:u32[])
        n643 = Multiply(x="ana_voltrange", y=12) -> (x*y=w1316:i32)
        n644 = Add(x="ana_mode", y=w1316) -> (x+y=w1313:i32)
        n645 = Index Array(array=w1293, index=w1313) -> (element=w1311:u32)
        n646 = Build Array("phoib_I_1s", "phoib_I_2s", "phoib_I_3s", "phoib_I_4s", "phoib_I_5s", "phoib_I_6s", "phoib_I_7s", "phoib_I_8s", "phoib_I_9s", "phoib_I_10s") -> (w1299:dbl[])
        n647 = call "SL2_AD_DLL_Phoibos_SetDeviceMode.vi"("pHandle"=w1307, "error in"=w1309, "value"=w1311, "dev_type"=DEF_dev_type."devA (analyzer)", "dll path in"=w1310) -> ("error out"=w1298:errorcluster, "dll path out"=w1308:path)  [unwired: 4 in]
        n648 = for {
          tunnel: w1307 -> [w1327]
          shift-right: [w1334] -> w1321
          shift-left: w1308 -> [w1331]
          tunnel: w1300 -> [w1326] mode=indexing
          tunnel: w1299 -> [w1325] mode=indexing
          shift-right: [w1333] -> w1320
          shift-left: w1298 -> [w1329]
          n649 = call "SL2_AD_DLL_Phoibos_GetVoltageRange.vi"("error in"=w1329, "voltage_name"=w1326, "pHandle"=w1327, "dll path in"=w1331) -> ("error out"=w1328:errorcluster, "min"=w1323:dbl, "max"=w1324:dbl, "dll path out"=w1330:path)  [unwired: 2 in]
          n650 = In Range and Coerce(upper limit=w1324, x=w1325, lower limit=w1323) -> (coerced(x)=w1322:dbl)  [unwired: 1 out]
          n651 = call "SL2_AD_DLL_Phoibos_SetVoltage.vi"("commit"=TRUE, "pHandle"=w1327, "error in"=w1328, "value"=w1322, "voltageName"=w1326, "dll path in"=w1330) -> ("error out"=w1333:errorcluster, "dll path out"=w1334:path)  [unwired: 3 in]
        }
      }
      frame "setsgl" {
        n652 = Dequeue Element(queue=w1374) -> ()  [unwired: 2 in, 4 out]
        n653 = Match Pattern(string=w1370, regular expression=":") -> (before substring=w1363:string, after substring=w1372:string)  [unwired: 1 in, 2 out]
        n654 = Equal?(x=w1372, y="wait") -> ()  [unwired: 1 out]
        n655 = Match Pattern(string=w1363, regular expression=":") -> (before substring=w1337:string, after substring=w1362:string)  [unwired: 1 in, 2 out]
        n656 = Fract/Exp String To Number(string=w1362) -> (number=w1361:dbl)  [unwired: 3 in, 1 out]
        n657 = call "SL2_AD_DLL_Phoibos_GetVoltageRange.vi"("voltage_name"=w1337, "pHandle"=w1358, "dll path in"=w1360) -> ("error out"=w1367:errorcluster, "min"=w1365:dbl, "max"=w1366:dbl, "dll path out"=w1368:path)  [unwired: 3 in]
        n658 = In Range and Coerce(upper limit=w1366, x=w1361, lower limit=w1365) -> (coerced(x)=w1356:dbl)  [unwired: 1 out]
        n659 = call "SL2_AD_DLL_Phoibos_SetVoltage.vi"("commit"=TRUE, "pHandle"=w1358, "error in"=w1367, "value"=w1356, "voltageName"=w1337, "dll path in"=w1368) -> ("error out"=w1357:errorcluster, "dll path out"=w1359:path)  [unwired: 3 in]
        n660 = while {
          tunnel: w1359 -> [w1390]
          tunnel: w1358 -> [w1384]
          tunnel: w1337 -> [w1389]
          tunnel: w1357 -> [w1388]
          tunnel: w1356 -> [w1387]
          tunnel: [w1384] -> w1338
          tunnel: [w1383] -> w1340
          tunnel: [w1382] -> w1342
          stop <- w1385 stop-if-true
          n661 = call "SL2_AD_DLL_Phoibos_GetVoltage.vi"("error in"=w1388, "voltage_name"=w1389, "pHandle"=w1384, "dll path in"=w1390) -> ("error out"=w1382:errorcluster, "value"=w1386:dbl, "dll path out"=w1383:path)  [unwired: 3 in]
          n662 = Equal?(x=w1387, y=w1386) -> (x = y?=w1385:bool)
        }
        n663 = for {
          tunnel: w1338 -> [w1381]
          tunnel: [w1379] -> w1343 mode=indexing
          tunnel: [w1378] -> w1339
          shift-right: [w1377] -> w1341
          shift-left: w1342 -> [w1380]
          tunnel: w1340 -> [w1376]
          tunnel: w1336 -> [w1375] mode=indexing
          n664 = call "SL2_AD_DLL_Phoibos_GetVoltage.vi"("error in"=w1380, "voltage_name"=w1375, "pHandle"=w1381, "dll path in"=w1376) -> ("error out"=w1377:errorcluster, "value"=w1379:dbl, "dll path out"=w1378:path)  [unwired: 3 in]
        }
        n665 = Index Array(array=w1343) -> (element #1=w1344:dbl, element #2=w1345:dbl, element #3=w1346:dbl, element #4=w1347:dbl, element #5=w1348:dbl, element #6=w1352:dbl, element #7=w1349:dbl, element #8=w1350:dbl, element #9=w1351:dbl, element #10=w1335:dbl)  [unwired: 10 in]
        n666 = local write "phoib_I_1"(w1344) -> ()
        n667 = local write "phoib_I_2"(w1345) -> ()
        n668 = local write "phoib_I_3"(w1346) -> ()
        n669 = local write "phoib_I_4"(w1347) -> ()
        n670 = local write "phoib_I_5"(w1348) -> ()
        n671 = local write "phoib_I_6"(w1352) -> ()
        n672 = local write "phoib_I_7"(w1349) -> ()
        n673 = local write "phoib_I_8"(w1350) -> ()
        n674 = local write "phoib_I_9"(w1351) -> ()
        n675 = local write "phoib_I_10"(w1335) -> ()
        n676 = Send Notification(notification=TRUE, notifier=w1354, error in (no error)=w1341) -> (error out=w1355:errorcluster)  [unwired: 1 out]
      }
      frame "standby" {
        w1397 = T3 0 items=["Off"=-1, "Standby"=0, "On"=1] ("state")
        n677 = Dequeue Element(queue=w1391) -> ()  [unwired: 2 in, 4 out]
        n678 = call "SL2_AD_DLL_Phoibos_SetDeviceState.vi"("pHandle_in"=w1392, "error in"=w1395, "state"=w1397, "dev_type"=DEF_dev_type."devA (analyzer)", "dll_path"=w1396) -> ("error out"=w1393:errorcluster, "path out"=w1394:path)  [unwired: 2 in]
      }
      frame "release" {
        n679 = Dequeue Element(queue=w1409) -> (queue out=w1399:refnum<queue>)  [unwired: 2 in, 3 out]
        n680 = flat-sequence {
          tunnel: w1408 -> [w1410]
          tunnel: w1404 -> [w1411]
          tunnel: [w1414] -> w1403
          tunnel: [w1413] -> w1402
          tunnel: [u32 0] -> w1401
          tunnel: [w1416] -> w1405
          tunnel: [w1417] -> w1406
          tunnel: [w1418] -> w1407
          tunnel: w1403 -> [w1418]
          tunnel: w1402 -> [w1417]
          tunnel: w1401 -> [w1416]
          frame #0 {
            n681 = call "SL2_AD_DLL_Phoibos_Shutdown.vi"("pHandle"=w1411, "dll path in"=w1410) -> ("error out"=w1413:errorcluster, "dll path out"=w1414:path)  [unwired: 4 in]
          }
          frame #1 {
            n682 = local write "phoib_con?"(FALSE ("phoib_con?")) -> ()
          }
        }
        n683 = Enqueue Element(queue=w1399, element="suspend") -> ()  [unwired: 2 in, 3 out]
      }
      frame "close" {
        n684 = Release Queue(queue=w1423) -> ()  [unwired: 2 in, 3 out]
      }
      frame "suspend" {
        n685 = Dequeue Element(queue=w1428) -> ()  [unwired: 2 in, 4 out]
      }
      frame "init" {
        n686 = Dequeue Element(queue=w1433) -> ()  [unwired: 2 in, 4 out]
        n687 = flat-sequence {
          tunnel: [w1440] -> w1431
          tunnel: [w1436] -> w1430
          tunnel: [w1435] -> w1429
          tunnel: [w1448] -> w1432
          tunnel: w1431 -> [w1448]
          frame #0 {
            n688 = local write "phoib_con?"(FALSE ("phoib_con?")) -> ()
          }
          frame #1 {
            w1439 = DEF_dev_type."devA (analyzer)" ("dev_type")
            n689 = call "GetSL2AD_VI_dllPath.vi"() -> ("error"=w1443:errorcluster, "Path"=w1444:path)  [unwired: 9 in, 1 out]
            n690 = call "SL2_AD_DLL_List_Devices.vi"("error in"=w1443, "dev_type"=w1439, "dll path in"=w1444) -> ("error out"=w1437:errorcluster, "devices"=w1446:string[], "dll path out"=w1438:path)  [unwired: 2 in]
            n691 = Index Array(array=w1446) -> (element=w1445:string)  [unwired: 1 in]
            n692 = call "SL2_AD_DLL_Phoibos_Initialize.vi"("error in"=w1437, "analyzerId"=w1445, "dll_path"=w1438) -> ("error out"=w1441:errorcluster, "pHandle"=w1440:u32, "path out"=w1442:path)  [unwired: 2 in]
            n693 = call "SL2_AD_DLL_Phoibos_ListDeviceModes.vi"("dll path in"=w1442, "dev_type"=w1439, "pHandle"=w1440, "error in"=w1441) -> ("dll path out"=w1436:path, "error out"=w1435:errorcluster)  [unwired: 1 in, 2 out]
          }
          frame #2 {
            n694 = local write "phoib_con?"(TRUE ("phoib_con?")) -> ()
          }
        }
      }
    }
    "phoib_error" <- w1246
  }
  n695 = while {
    tunnel: w9 -> [w1458]
    tunnel: w8 -> [w1452]
    shift-right: [w1451] -> _
    shift-left: 0 -> [w1450]
    stop <- w1449 stop-if-true
    # "temp"
    n696 = Preview Queue Element(queue=w1458, timeout in ms (-1)=w1450) -> (queue out=w1453:refnum<queue>, element=w1457:string)  [unwired: 1 in, 2 out]
    n697 = Match Pattern(string=w1457, regular expression=":") -> (before substring=w1456:string, after substring=w1455:string)  [unwired: 1 in, 2 out]
    n698 = case shown="\"ramp\"" w1456 {
      tunnel: w1455 -> [w1464 _ _ _ _]
      tunnel: w1453 -> [w1459 w1484 w1485 _ w1498]
      tunnel: w1452 -> [w1460 _ _ _ _]
      tunnel: [_ _ _ _ -1] -> w1451
      tunnel: [_ TRUE _ _ _] -> w1449
      frame "ramp" {
        n699 = Dequeue Element(queue=w1459) -> ()  [unwired: 2 in, 4 out]
        n700 = Match Pattern(string=w1464, regular expression=":") -> (before substring=w1463:string, after substring=w1467:string)  [unwired: 1 in, 2 out]
        n701 = Equal?(x=w1467, y="wait") -> (x = y?=w1461:bool)
        n702 = Scan From String(input string=w1463) -> (output 1=w1462:dbl)  [unwired: 4 in, 3 out]
        n703 = flat-sequence {
          tunnel: w1462 -> [w1469]
          tunnel: w1461 -> [w1471]
          tunnel: w1460 -> [w1481]
          frame #0 {
            n704 = local read "LS310  EPICS SP"() -> (w1468:string)
            n705 = call-poly <userlib>:"CaLabPut.vi"("Value"=w1469, "PV Name"=w1468) -> ()  [unwired: 6 in, 4 out]
          }
          frame #1 {
            n706 = Wait (ms)(milliseconds to wait=500) -> ()  [unwired: 1 out]
          }
          frame #2 {
            n707 = case shown="True" w1471 {
              frame False {
              }
              frame True {
                n708 = while {
                  stop <- w1477 stop-if-true
                  n709 = local read "Status EPICS chanel"() -> (w1479:string)
                  n710 = Wait (ms)(milliseconds to wait=500) -> ()  [unwired: 1 out]
                  n711 = call-poly <userlib>:"CaLabGet.vi"("PV Name"=w1479) -> ("1rst Value (string)"=w1480:string)  [unwired: 8 in, 6 out]
                  n712 = Equal?(x=w1480, y="Inside Range") -> (x = y?=w1477:bool)
                  n713 = local read "LS310  EPICS chanel A"() -> (w1473:string)
                  n714 = local read "LS310  EPICS chanel B"() -> (w1472:string)
                  n715 = call-poly <userlib>:"CaLabGet.vi"("PV Name"=w1473) -> ("1rst Value (number)"=w1474:dbl)  [unwired: 8 in, 6 out]
                  n716 = call-poly <userlib>:"CaLabGet.vi"("PV Name"=w1472) -> ("1rst Value (number)"=w1475:dbl)  [unwired: 8 in, 6 out]
                  n717 = local write "TB"(w1475) -> ()
                  n718 = local write "TA"(w1474) -> ()
                }
              }
            }
          }
          frame #3 {
            n719 = Send Notification(notification=TRUE, notifier=w1481) -> ()  [unwired: 1 in, 2 out]
          }
        }
      }
      frame "close" {
        n720 = Release Queue(queue=w1484) -> ()  [unwired: 2 in, 3 out]
      }
      frame "init" {
        n721 = Dequeue Element(queue=w1485) -> ()  [unwired: 2 in, 4 out]
      }
      frame "idle", Default {
        n722 = local read "LS310  EPICS chanel A"() -> (w1496:string)
        n723 = local read "LS310  EPICS chanel B"() -> (w1495:string)
        n724 = local read "LS310  EPICS SP"() -> (w1486:string)
        n725 = local read "Status EPICS chanel"() -> (w1494:string)
        n726 = local read "LS310  EPICS Heater"() -> (w1493:string)
        n727 = call-poly <userlib>:"CaLabGet.vi"("PV Name"=w1496) -> ("1rst Value (number)"=→"TA":dbl)  [unwired: 8 in, 6 out]
        n728 = call-poly <userlib>:"CaLabGet.vi"("PV Name"=w1495) -> ("1rst Value (number)"=→"TB":dbl)  [unwired: 8 in, 6 out]
        n729 = call-poly <userlib>:"CaLabGet.vi"("PV Name"=w1486) -> ("1rst Value (number)"=→"Readback":dbl)  [unwired: 8 in, 6 out]
        n730 = call-poly <userlib>:"CaLabGet.vi"("PV Name"=w1494) -> ("1rst Value (string)"=w1490:string)  [unwired: 8 in, 6 out]
        n731 = call-poly <userlib>:"CaLabGet.vi"("PV Name"=w1493) -> ()  [unwired: 8 in, 7 out]
        n732 = Equal?(x=w1490, y="Inside Range") -> (x = y?=→"In Range":bool)
      }
      frame "suspend" {
        n733 = Dequeue Element(queue=w1498) -> ()  [unwired: 2 in, 4 out]
      }
    }
  }
  n734 = while {
    tunnel: w6 -> [w1508]
    tunnel: w8 -> [w1502]
    shift-right: [w1501] -> _
    shift-left: _ -> [w1500]
    stop <- w1499 stop-if-true
    # "temp"
    n735 = Preview Queue Element(queue=w1508, timeout in ms (-1)=w1500) -> (queue out=w1503:refnum<queue>, element=w1507:string)  [unwired: 1 in, 2 out]
    n736 = Match Pattern(string=w1507, regular expression=":") -> (before substring=w1506:string, after substring=w1505:string)  [unwired: 1 in, 2 out]
    n737 = case shown="\"idle\", Default" w1506 {
      tunnel: w1505 -> [w1515 _ _ _ _]
      tunnel: w1503 -> [w1510 w1535 w1536 _ w1540]
      tunnel: w1502 -> [w1511 _ _ _ _]
      tunnel: [_ _ _ _ -1] -> w1501
      tunnel: [_ TRUE _ _ _] -> w1499
      frame "abs" {
        n738 = Dequeue Element(queue=w1510) -> ()  [unwired: 2 in, 4 out]
        n739 = Match Pattern(string=w1515, regular expression=":") -> (before substring=w1514:string, after substring=w1518:string)  [unwired: 1 in, 2 out]
        n740 = Equal?(x=w1518, y="wait") -> (x = y?=w1512:bool)
        n741 = Scan From String(input string=w1514) -> (output 1=w1513:dbl)  [unwired: 4 in, 3 out]
        n742 = flat-sequence {
          tunnel: w1513 -> [w1519]
          tunnel: [w1519] -> w1509
          tunnel: w1512 -> [w1522]
          tunnel: w1509 -> [w1521]
          tunnel: w1511 -> [w1532]
          frame #0 {
            n743 = local read "WattPilot EPICS chanel set"() -> (w1520:string)
            n744 = call-poly <userlib>:"CaLabPut.vi"("Value"=w1519, "PV Name"=w1520) -> ()  [unwired: 6 in, 4 out]
          }
          frame #1 {
            n745 = case shown="True" w1522 {
              tunnel: w1521 -> [_ w1523]
              frame False {
              }
              frame True {
                n746 = while {
                  tunnel: w1523 -> [w1528]
                  stop <- w1525 stop-if-true
                  n747 = local read "WattPilot EPICS chanel readback"() -> (w1530:string)
                  n748 = Wait (ms)(milliseconds to wait=500) -> ()  [unwired: 1 out]
                  n749 = call-poly <userlib>:"CaLabGet.vi"("PV Name"=w1530) -> ("1rst Value (number)"=w1529:dbl)  [unwired: 8 in, 6 out]
                  n750 = Subtract(x=w1529, y=w1528) -> (x-y=w1527:dbl)
                  n751 = Absolute Value(x=w1527) -> (abs(x)=w1526:dbl)
                  n752 = local write "Readback_wattpilot"(w1529) -> ()
                  n753 = Less?(x=w1526, y=0.1) -> (x < y?=w1525:bool)
                }
              }
            }
          }
          frame #2 {
            n754 = Send Notification(notification=TRUE, notifier=w1532) -> ()  [unwired: 1 in, 2 out]
          }
        }
      }
      frame "close" {
        n755 = Release Queue(queue=w1535) -> ()  [unwired: 2 in, 3 out]
      }
      frame "init" {
        n756 = Dequeue Element(queue=w1536) -> ()  [unwired: 2 in, 4 out]
      }
      frame "idle", Default {
        n757 = local read "WattPilot EPICS chanel readback"() -> (w1538:string)
        n758 = call-poly <userlib>:"CaLabGet.vi"("PV Name"=w1538) -> ("1rst Value (number)"=→"Readback_wattpilot":dbl)  [unwired: 8 in, 6 out]
      }
      frame "suspend" {
        n759 = Dequeue Element(queue=w1540) -> ()  [unwired: 2 in, 4 out]
      }
    }
  }
  n760 = while {
    tunnel: w25 -> [w1567]
    shift-right: [w1561] -> _
    shift-left: _ -> [w1560]
    shift-right: [w1559] -> _
    shift-left: _ -> [w1557]
    shift-right: [w1558] -> _
    shift-left: _ -> [w1556]
    shift-right: [w1553] -> _
    shift-left: 0 -> [w1554]
    shift-right: [w1552] -> _
    shift-left: _ -> [w1551]
    shift-right: [w1550] -> _
    shift-left: _ -> [w1549]
    tunnel: w34 -> [w1548]
    shift-right: [w1547] -> _
    shift-left: _ -> [w1546]
    shift-right: [w1544] -> _
    shift-left: _ -> [w1543]
    shift-right: [w1542] -> _
    shift-left: _ -> [w1541]
    i -> [w1545]
    stop <- w1555 stop-if-true
    # "cam"
    n761 = Preview Queue Element(queue=w1567, timeout in ms (-1)=w1554) -> (queue out=w1566:refnum<queue>, element=w1565:string)  [unwired: 1 in, 2 out]
    n762 = Match Pattern(string=w1565, regular expression=":") -> (before substring=w1562:string, after substring=w1563:string)  [unwired: 1 in, 2 out]
    n763 = case shown="\"close\"" w1562 {
      tunnel: w1566 -> [w1579 w1611 w1644 w1657 _ w1745 w1775 w1840]
      tunnel: w1563 -> [_ _ _ _ _ _ _ _]
      tunnel: [w1573 w1598 w1643 w1655 w1698 w1742 w1760 w1838] -> w1561
      tunnel: w1560 -> [_ _ w1643 w1655 w1698 w1742 w1760 w1838]
      tunnel: [w1578 w1612 u64 0 ("Hout") w1654 w1702 w1743 w1770 w1837] -> w1559
      tunnel: [w1580 w1613 w1640 w1653 w1703 w1744 w1761 w1836] -> w1558
      tunnel: w1557 -> [_ w1615 w1642 w1654 w1705 w1747 w1772 w1837]
      tunnel: w1556 -> [_ w1614 _ w1653 w1704 w1746 w1771 w1836]
      tunnel: [_ _ _ TRUE _ _ _ _] -> w1555
      tunnel: [_ _ -1 _ _ _ _ -1] -> w1553
      tunnel: [w1572 w1599 _ _ w1712 _ _ _] -> w1552
      tunnel: w1551 -> [w1572 w1599 _ _ w1711 _ _ _]
      tunnel: [w1573 w1601 w1638 w1652 w1707 w1736 w1773 w1835] -> w1550
      tunnel: w1549 -> [_ w1601 w1638 w1652 w1707 _ w1773 w1835]
      tunnel: w1548 -> [_ _ _ _ _ _ w1764 _]
      tunnel: [w1570 w1596 w1637 w1650 w1665 w1733 w1767 w1834] -> w1547
      tunnel: w1546 -> [w1570 w1596 w1637 w1650 w1700 w1733 w1767 w1834]
      tunnel: w1545 -> [_ _ _ _ w1673 _ _ _]
      tunnel: [w1571 w1597 w1636 w1651 w1699 w1732 w1766 w1833] -> w1544
      tunnel: w1543 -> [w1571 w1597 w1636 w1651 w1672 w1732 w1766 w1833]
      tunnel: [w1569 w1593 refnum<k21> refnum ("task out") w1649 w1658 w1731 w1757 w1832] -> w1542
      tunnel: w1541 -> [_ w1593 w1635 w1649 w1658 w1731 w1758 w1832]
      frame "init" {
        w1573 = u16[][] []
        n764 = flat-sequence {
          tunnel: [w1582] -> w1577
          tunnel: [w1583] -> w1576
          tunnel: [w1591] -> w1578
          tunnel: [w1592] -> w1580
          tunnel: w1577 -> [w1592]
          tunnel: w1576 -> [w1591]
          frame #0 {
            n765 = local write "cam_con?"(FALSE ("cam_con?")) -> ()
          }
          frame #1 {
            n766 = call "SCInitBoard.vi"("boardnr"="board number") -> ("Hout"=w1586:u32, "error out"=w1587:errorcluster)  [unwired: 1 in, 1 out]
            n767 = call "SCSetupCamera.vi"("Handle"=w1586, "error in (no error)"=w1587) -> ("Hout"=w1588:u64, "error out"=w1589:errorcluster)  [unwired: 1 out]
            n768 = call "SCStopCOC.vi"("error in (no error)"=w1589, "Stop mode"=0, "Handle"=w1588) -> ("error out"=w1582:errorcluster, "Hout"=w1583:u64)
          }
          frame #2 {
            n769 = local write "cam_con?"(TRUE ("cam_con?")) -> ()
          }
        }
        n770 = Dequeue Element(queue=w1579) -> (queue out=w1575:refnum<queue>)  [unwired: 2 in, 3 out]
        n771 = Enqueue Element At Opposite End(queue=w1575, element="set") -> ()  [unwired: 2 in, 3 out]
        n772 = call-poly <vilib>:"DAQmx Create Virtual Channel.vi"("lines"=tag "Dev3/port0/line0") -> ("task out"=w1569:refnum<k21>)  [unwired: 13 in, 1 out]
      }
      frame "set" {
        n773 = Dequeue Element(queue=w1611) -> ()  [unwired: 2 in, 4 out]
        n774 = call "SCStopCOC.vi"("error in (no error)"=w1614, "Stop mode"=0, "Handle"=w1615) -> ("error out"=w1630:errorcluster, "Hout"=w1629:u64)
        n775 = Bundle By Name(cluster=cluster{"Delay":dbl, "Exposure ":dbl} {"Delay"=0.0, "Exposure "=0.0} ("Delay and exposure"), "Exposure"="cam_exp") -> (w1608:cluster{"Delay":dbl, "Exposure ":dbl})
        n776 = Bundle By Name(cluster=T11 {"Camera type"=0, "Operating mode\nHP & QE / HS & DiCam Pro "=0, "Frame trigger \n(High Performance and QE only)"=0, "Sequence trigger"=0, "Low Light\n(QE only)"=FALSE, "Gain"=FALSE, "Horzontal\nbinning"=0, "Vertical\nbinning "=0, "ROI Left"=1, "ROI Right"=20, "ROI Top"=1, "ROI Bottom"=15} ("Camera controls"), "Operating mode\nHP & QE / HS & DiCam Pro"="Operating mode\nHP & QE / HS & DiCam Pro", "Horzontal\nbinning"="binning", "Vertical\nbinning"="binning", "ROI Left"="ROI Left", "ROI Right"="ROI Right", "ROI Top"="ROI Top", "ROI Bottom"="ROI Bottom", "Gain"="gain", "Frame trigger \n(High Performance and QE only)"="Frame trigger \n(High Performance and QE only)") -> (w1625:T11)
        n777 = call "New delay and exposure forma.vi"("Operating mode\nHP & QE / HS & DiCam Pro"="Operating mode\nHP & QE / HS & DiCam Pro", "Delay and exposure"=w1608) -> ("Output table"=w1626:string)  [unwired: 3 in]
        n778 = call "SCSetCoC.vi"("error in (no error)"=w1630, "Delay and exposure table"=w1626, "Camera controls"=w1625, "Handle"=w1629) -> ("error out"=w1618:errorcluster, "Hout"=w1617:u64)  [unwired: 1 out]
        n779 = call "SCGetImageSize.vi"("Handle"=w1617, "error in (no error)"=w1618) -> ("Hout"=w1616:u64, "error out"=w1600:errorcluster, "Horizontal size"=w1605:i32, "Vertical size"=w1604:i32)  [unwired: 2 out]
        n780 = Greater?(x=w1605, y=w1604) -> (0:w1606:bool)
        n781 = Initialize Array(u16 0 ("dimension size"), w1604, w1605) -> (w1598:u16[][])
        n782 = call "SCRun.vi"("error in (no error)"=w1600, "Run mode"=0, "Handle"=w1616) -> ("error out"=w1613:errorcluster, "Hout"=w1612:u64)  [unwired: 1 out]
        n783 = Select(t=w1605, s=w1606, f=w1604) -> (s? t:f=w1603:i32)
        n784 = property on="mainimg" class="IntGraph (strict)"("XScale.Maximum"=w1603, "YScale.Maximum"=w1603) -> ()  [unwired: 2 in, 2 out]
      }
      frame "release" {
        n785 = Dequeue Element(queue=w1644) -> (queue out=w1631:refnum<queue>)  [unwired: 2 in, 3 out]
        n786 = flat-sequence {
          tunnel: w1642 -> [w1646]
          tunnel: [w1645] -> w1639
          tunnel: [w1648] -> w1640
          tunnel: w1639 -> [w1648]
          frame #0 {
            n787 = call "SCCloseBoard.vi"("Handle"=w1646) -> ("error out"=w1645:errorcluster)  [unwired: 1 in, 2 out]
          }
          frame #1 {
            n788 = local write "cam_con?"(FALSE ("cam_con?")) -> ()
          }
        }
        n789 = Enqueue Element(queue=w1631, element="suspend") -> ()  [unwired: 2 in, 3 out]
        n790 = call <vilib>:"DAQmx Clear Task.vi"("task in"=w1635) -> ()  [unwired: 14 in, 1 out]
      }
      frame "close" {
        n791 = Release Queue(queue=w1657) -> ()  [unwired: 2 in, 3 out]
      }
      frame "idle", Default {
        n792 = call "grabimg.vi"("array in"=w1698, "error in"=w1704, "Hin"=w1705) -> ("error out"=w1703:errorcluster, "imgdata"=w1701:i32[][], "Hout"=w1702:u64)  [unwired: 6 in]
        n793 = local read "lower threshold"() -> (w1696:i32)
        n794 = case shown="True" "cam_dark?" {
          tunnel: w1707 -> [_ w1730]
          tunnel: [w1727 w1729] -> w1697
          tunnel: w1701 -> [w1727 w1728]
          frame False {
          }
          frame True {
            n795 = Subtract(x=w1728, y=w1730) -> (x-y=w1729:dbl[][])
          }
        }
        n796 = call "filtr_b.vi"("threshold"=w1696, "input array"=w1697) -> ("output array"=w1688:dbl[][])  [unwired: 9 in]
        n797 = call <vilib>:"High Resolution Relative Seconds.vi"() -> ("relative seconds"=w1712:dbl)
        n798 = Subtract(x=w1712, y=w1711) -> (x-y=w1710:dbl)
        n799 = Array Size(array=w1688) -> (size(s)=w1687:i32[])
        n800 = Reciprocal(x=w1710) -> (1/x=→"cam_fps":dbl)
        n801 = Index Array(array=w1687) -> (element #1=w1682:i32, element #2=w1681:i32)  [unwired: 2 in]
        n802 = Subtract(x=w1673, y=w1672) -> (x-y=w1671:i32)
        n803 = Less Or Equal?(x="pics2avg", y=w1671) -> (x <= y?=w1694:bool)
        n804 = And(x="reset every n pics", y=w1694) -> (x .and. y?=w1692:bool)
        n805 = Not(x=w1692) -> (.not. x?=w1691:bool)
        n806 = call-poly <vilib>:"Ramp Pattern.vi"("start"=0.0, "end"=w1682, "samples"=w1682) -> ("Ramp Pattern"=w1677:dbl[])  [unwired: 7 in, 1 out]
        n807 = call-poly <vilib>:"Ramp Pattern.vi"("start"=0.0, "end"=w1681, "samples"=w1681) -> ("Ramp Pattern"=w1678:dbl[])  [unwired: 7 in, 1 out]
        n808 = property on="mainimg" class="IntGraph (strict)"() -> ("CrsrLis"=w1670:T5)  [unwired: 2 in, 2 out]
        n809 = And(x="cam_liveavg", y=w1691) -> (x .and. y?=w1689:bool)
        n810 = case shown="False" w1689 {
          tunnel: w1688 -> [w1717 w1723]
          tunnel: [w1717 w1720] -> w1665
          tunnel: w1700 -> [_ w1725]
          tunnel: w1673 -> [w1718 _]
          tunnel: [w1718 w1726] -> w1699
          tunnel: w1672 -> [_ w1726]
          tunnel: w1671 -> [_ w1719]
          frame False {
          }
          frame True {
            n811 = Multiply(x=w1725, y=w1719) -> (x*y=w1724:dbl[][])
            n812 = Increment(x=w1719) -> (x+1=w1721:i32)
            n813 = Add(x=w1724, y=w1723) -> (x+y=w1722:dbl[][])
            n814 = Divide(x=w1722, y=w1721) -> (x/y=w1720:dbl[][])
          }
        }
        "mainimg" <- w1665
        n815 = Index Array(array=w1670) -> (element #1=w1668:T12, element #2=w1669:T12)  [unwired: 2 in]
        n816 = Unbundle By Name(w1668) -> ("Position.X"=w1662:dbl, "Position.Y"=w1664:dbl)
        n817 = Unbundle By Name(w1669) -> ("Position.X"=w1666:dbl, "Position.Y"=w1667:dbl)
        n818 = Array Max & Min(array=w1665) -> (max value=→"max":dbl)  [unwired: 3 out]
        n819 = Subtract(x=w1667, y=w1664) -> (x-y=w1663:dbl)
        n820 = Subtract(x=w1666, y=w1662) -> (x-y=w1661:dbl)
        n821 = Array Subset(array=w1665, index (row)=w1664, length (row)=w1663) -> (w1676:dbl[][])  [unwired: 2 in]
        n822 = Array Subset(array=w1665, index (col)=w1662, length (col)=w1661) -> (w1674:dbl[][])  [unwired: 2 in]
        n823 = Array Subset(array=w1665, index (row)=w1664, length (row)=w1663, index (col)=w1662, length (col)=w1661) -> (w1660:dbl[][])
        n824 = Transpose 2D Array(2D array=w1676) -> (transposed array=w1675:dbl[][])
        n825 = Add Array Elements(numeric array=w1660) -> (sum=→"sum" →"Waveform Chart":dbl)
        n826 = for {
          tunnel: w1674 -> [w1714] mode=indexing
          tunnel: [w1713] -> w1684 mode=indexing
          n827 = Add Array Elements(numeric array=w1714) -> (sum=w1713:dbl)
        }
        n828 = for {
          tunnel: w1675 -> [w1716] mode=indexing
          tunnel: [w1715] -> w1683 mode=indexing
          n829 = Add Array Elements(numeric array=w1716) -> (sum=w1715:dbl)
        }
        n830 = Bundle("Ramp Pattern"=w1678, w1683) -> (→"G2 X":cluster{"Ramp Pattern":dbl[], dbl[]})  [unwired: 1 in]
        n831 = Bundle(w1684, "Ramp Pattern"=w1677) -> (→"G2 Y":cluster{dbl[], "Ramp Pattern":dbl[]})  [unwired: 1 in]
      }
      frame "dark" {
        n832 = Dequeue Element(queue=w1745) -> ()  [unwired: 2 in, 4 out]
        n833 = Array Size(array=w1742) -> (size(s)=w1741:i32[])
        n834 = Index Array(array=w1741) -> (element #1=w1740:i32, element #2=w1739:i32)  [unwired: 2 in]
        n835 = Initialize Array(0.0 ("element"), w1740, w1739) -> (w1737:dbl[][])
        n836 = for {
          N: "dark avg" -> [_]
          tunnel: w1747 -> [w1755]
          tunnel: w1746 -> [w1754]
          tunnel: [w1753] -> w1744
          tunnel: w1742 -> [w1752]
          tunnel: [w1751] -> w1743
          shift-right: [w1748] -> w1735
          shift-left: w1737 -> [w1749]
          n837 = call "grabimg.vi"("array in"=w1752, "error in"=w1754, "Hin"=w1755) -> ("error out"=w1753:errorcluster, "imgdata"=w1750:i32[][], "Hout"=w1751:u64)  [unwired: 6 in]
          n838 = Add(x=w1750, y=w1749) -> (x+y=w1748:dbl[][])
        }
        n839 = Divide(x=w1735, y="dark avg") -> (x/y=w1736:dbl[][])
      }
      frame "snap" {
        n840 = Dequeue Element(queue=w1775) -> ()  [unwired: 2 in, 4 out]
        n841 = local read "cam_dark?"() -> (w1774:bool)
        n842 = local read "cam_avgs"() -> (w1769:i32)
        n843 = To Double Precision Float(number=w1760) -> (double precision float=w1759:dbl[][])
        n844 = Equal To 0?(x="aq.mode") -> (x = 0?=w1762:bool)
        n845 = Get Date/Time In Seconds() -> (seconds since 1Jan1904=w1765:timestamp)
        n846 = for {
          N: w1769 -> [w1787]
          shift-right: [w1804] -> w1770
          shift-left: w1772 -> [w1806]
          shift-right: [w1792] -> w1768
          shift-left: w1771 -> [w1805]
          tunnel: w1774 -> [w1802]
          tunnel: w1773 -> [w1801]
          tunnel: w1760 -> [w1800]
          tunnel: w1765 -> [w1796]
          tunnel: w1762 -> [w1780]
          shift-right: [w1788] -> w1756
          shift-left: w1759 -> [w1789]
          shift-right: [w1778] -> w1757
          shift-left: w1758 -> [w1778]
          i -> [w1776]
          stop <- "abort acq." stop-if-true
          n847 = call "grabimg.vi"("array in"=w1800, "error in"=w1805, "Hin"=w1806) -> ("error out"=w1792:errorcluster, "imgdata"=w1803:i32[][], "Hout"=w1804:u64)  [unwired: 6 in]
          n848 = local read "lower threshold"() -> (w1783:i32)
          n849 = Increment(x=w1776) -> (x+1=w1785:i32)
          "acq. imgs" <- w1785
          n850 = Get Date/Time In Seconds() -> (seconds since 1Jan1904=w1799:timestamp)
          n851 = case shown="True" w1802 {
            tunnel: w1803 -> [w1828 w1831]
            tunnel: w1801 -> [_ w1830]
            tunnel: [w1828 w1829] -> w1782
            frame False {
            }
            frame True {
              n852 = Subtract(x=w1831, y=w1830) -> (x-y=w1829:dbl[][])
            }
          }
          n853 = Divide(x=w1785, y=w1787) -> (x/y=→"snap_prog":dbl)
          n854 = Subtract(x=w1799, y=w1796) -> (x-y=w1798:dbl)
          n855 = call "filtr_b.vi"("threshold"=w1783, "input array"=w1782) -> ("output array"=w1781:dbl[][])  [unwired: 9 in]
          n856 = Divide(x=w1798, y=w1776) -> (x/y=w1794:dbl)
          n857 = Multiply(x=w1794, y=w1787) -> (x*y=w1797:dbl)
          n858 = Reciprocal(x=w1794) -> (1/x=w1793:dbl)
          n859 = case shown="True" "count?" {
            tunnel: w1781 -> [w1819 w1821]
            tunnel: "e-size" -> [_ w1823]
            tunnel: w1783 -> [_ w1822]
            tunnel: [w1819 w1820] -> w1779
            frame False {
            }
            frame True {
              n860 = Array Size(array=w1821) -> (size(s)=w1825:i32[])
              n861 = call "findr.vi"("thresh"=w1822, "esize"=w1823, "inp array"=w1821) -> ("locs"=w1824:i32[][])  [unwired: 8 in]
              n862 = Index Array(array=w1825) -> (element #1=w1827:i32, element #2=w1826:i32)  [unwired: 2 in]
              n863 = call "drawe.vi"("Ysize"=w1827, "Xsize"=w1826, "pos array"=w1824) -> ("img out"=w1820:i32[][])  [unwired: 8 in]
            }
          }
          n864 = Add(x=w1797, y=w1796) -> (x+y=→"ETA":timestamp)
          n865 = local write "cam_fps"(w1793) -> ()
          n866 = local write "mainimg"(w1781) -> ()
          n867 = case shown="True" w1780 {
            tunnel: w1779 -> [w1809 w1817]
            tunnel: w1789 -> [w1811 w1816]
            tunnel: [w1810 w1814] -> w1788
            tunnel: [w1808 w1813] -> w1777
            tunnel: w1776 -> [w1807 w1812]
            frame False {
              n868 = Add(x=w1809, y=w1811) -> (x+y=w1810:dbl[][])
              n869 = Increment(x=w1807) -> (x+1=w1808:i32)
            }
            frame True {
              n870 = Multiply(x=w1816, y=w1812) -> (x*y=w1818:dbl[][])
              n871 = Increment(x=w1812) -> (x+1=w1813:i32)
              n872 = Add(x=w1817, y=w1818) -> (x+y=w1815:dbl[][])
              n873 = Divide(x=w1815, y=w1813) -> (x/y=w1814:dbl[][])
            }
          }
          "Pics L" <- w1777
          n874 = local write "sideimg"(w1788) -> ()
        }
        n875 = Enqueue Element(queue=w1764, element=w1756, error in (no error)=w1768) -> (error out=w1761:errorcluster)  [unwired: 1 in, 2 out]
      }
      frame "suspend" {
        n876 = Dequeue Element(queue=w1840) -> ()  [unwired: 2 in, 4 out]
      }
    }
    "cam_error" <- w1558
  }
